vi "NM GlobalTest.vi"() -> ()   [LabVIEW 2010]
uses:
  C:/Program Files/National Instruments/LabVIEW 2010/vi.lib/ULx/ULx_LV.dll
  Program Files/National Instruments/LabVIEW 2010/vi.lib/ULx/ULx_LV.dll
  <vilib>/ULx/Create Channel.llb/ULx Create Channel (AI-Voltage-Basic).vi
  <vilib>/ULx/Create Channel.llb/ULx Create Channel (AI-Current-Basic).vi
  <vilib>/ULx/Create Channel.llb/ULx Create Channel (AI-Temperature).vi
  <vilib>/ULx/Create Channel.llb/ULx Create Channel (AO-Voltage-Basic).vi
  <vilib>/ULx/Create Channel.llb/ULx Create Channel (AO-Current-Basic).vi
  <vilib>/ULx/Create Channel.llb/ULx Create Channel (DI-Digital Input).vi
  <vilib>/ULx/Create Channel.llb/ULx Create Channel (DO-Digital Output).vi
  <vilib>/ULx/Create Channel.llb/ULx Create Channel (CI-Frequency).vi
  <vilib>/ULx/Create Channel.llb/ULx Create Channel (CI-Period).vi
  <vilib>/ULx/Create Channel.llb/ULx Create Channel (CI-Count Edges).vi
  <vilib>/ULx/Create Channel.llb/ULx Create Channel (CI-Position-Angular Encoder).vi
  <vilib>/ULx/Create Channel.llb/ULx Create Channel (CO-Pulse Generation-Frequency).vi
  <vilib>/ULx/Create Channel.llb/ULx Create Channel (CO-Pulse Generation-Time).vi
  <vilib>/ULx/Create Channel.llb/ULx Create Channel (CO-Pulse Generation-Ticks).vi
  <vilib>/ULx/Create Channel.llb/ULx Create Channel (CompI-Analog Input-Voltage).vi
  <vilib>/ULx/Create Channel.llb/ULx Create Channel (CompI-Analog Input-Temperature).vi
  <vilib>/ULx/Create Channel.llb/ULx Create Channel (CompI-Digital Input).vi
  <vilib>/ULx/Create Channel.llb/ULx Create Channel (CompI-Counter Input-Count Edges).vi
  <vilib>/ULx/Create Channel.llb/ULx Create Channel (CompO-Analog Output-Voltage).vi
  <vilib>/ULx/Create Channel.llb/ULx Create Channel (CompO-Digital Output).vi
  <vilib>/ULx/Timing.llb/ULx Timing (Sample Clock).vi
  <vilib>/ULx/Timing.llb/ULx Timing (Use Waveform).vi
  <vilib>/ULx/Timing.llb/ULx Timing (Implicit).vi
  <vilib>/ULx/Trigger.llb/ULx Basic Trigger (None).vi
  <vilib>/ULx/Trigger.llb/ULx Basic Trigger (Digital Edge).vi
  <vilib>/ULx/Trigger.llb/ULx Basic Trigger (Digital Level).vi
  <vilib>/ULx/Trigger.llb/ULx Basic Trigger (Analog Edge).vi
  <vilib>/ULx/Trigger.llb/ULx Basic Trigger (Digital Pattern).vi
  <vilib>/ULx/Trigger.llb/ULx Gated Trigger (None).vi
  <vilib>/ULx/Trigger.llb/ULx Gated Trigger (Digital Level).vi
  <vilib>/ULx/Trigger.llb/ULx Gated Trigger (Analog Level).vi
  <vilib>/ULx/Trigger.llb/ULx Gated Trigger (Analog Window).vi
  <vilib>/ULx/Trigger.llb/ULx Gated Trigger (Analog Hysteresis).vi
  <vilib>/ULx/Trigger.llb/ULx Composite Trigger Start (None).vi
  <vilib>/ULx/Trigger.llb/ULx Composite Trigger Start (ExtTTL).vi
  <vilib>/ULx/Trigger.llb/ULx Composite Trigger Start (Analog HW).vi
  <vilib>/ULx/Trigger.llb/ULx Composite Trigger Start (Analog SW).vi
  <vilib>/ULx/Trigger.llb/ULx Composite Trigger Start (Digital Pattern).vi
  <vilib>/ULx/Trigger.llb/ULx Composite Trigger Start (Counter).vi
  <vilib>/ULx/Trigger.llb/ULx Composite Trigger Stop (None).vi
  <vilib>/ULx/Trigger.llb/ULx Composite Trigger Stop (Analog SW).vi
  <vilib>/ULx/Trigger.llb/ULx Composite Trigger Stop (Digital Pattern).vi
  <vilib>/ULx/Trigger.llb/ULx Composite Trigger Stop (Counter).vi
  <vilib>/ULx/Write.llb/ULx Write (Analog 1D DBL 1Chan 1Samp).vi
  <vilib>/ULx/Write.llb/ULx Write (Analog Wfm 1Chan 1Samp).vi
  <vilib>/ULx/Write.llb/ULx Write (Analog 1D DBL 1Chan NSamp).vi
  <vilib>/ULx/Write.llb/ULx Write (Analog Wfm 1Chan NSamp).vi
  <vilib>/ULx/Write.llb/ULx Write (Analog 1D DBL NChan 1Samp).vi
  <vilib>/ULx/Write.llb/ULx Write (Analog 1D Wfm NChan 1Samp).vi
  <vilib>/ULx/Write.llb/ULx Write (Analog 2D DBL NChan NSamp).vi
  <vilib>/ULx/Write.llb/ULx Write (Analog 1D Wfm NChan NSamp).vi
  <vilib>/ULx/Write.llb/ULx Write (Digital 1D Bool NChan 1Samp 1Line).vi
  <vilib>/ULx/Write.llb/ULx Write (Digital 2D Bool NChan 1Samp NLine).vi
  <vilib>/ULx/Write.llb/ULx Write (Digital 1D U8 NChan 1Samp).vi
  <vilib>/ULx/Write.llb/ULx Write (Digital 1D U16 NChan 1Samp).vi
  <vilib>/ULx/Write.llb/ULx Write (Digital 1D U32 NChan 1Samp).vi
  <vilib>/ULx/Write.llb/ULx Write (Digital 1D Wfm NChan 1Samp).vi
  <vilib>/ULx/Write.llb/ULx Write (Digital 2D U8 NChan NSamp).vi
  <vilib>/ULx/Write.llb/ULx Write (Digital 2D U16 NChan NSamp).vi
  <vilib>/ULx/Write.llb/ULx Write (Digital 2D U32 NChan NSamp).vi
  <vilib>/ULx/Write.llb/ULx Write (Digital 1D Wfm NChan NSamp).vi
  <vilib>/ULx/Write.llb/ULx Write (Digital Bool 1Line 1Point).vi
  <vilib>/ULx/Write.llb/ULx Write (Digital 1D Bool 1Chan 1Samp).vi
  <vilib>/ULx/Write.llb/ULx Write (Digital U8 1Chan 1Samp).vi
  <vilib>/ULx/Write.llb/ULx Write (Digital U16 1Chan 1Samp).vi
  <vilib>/ULx/Write.llb/ULx Write (Digital U32 1Chan 1Samp).vi
  <vilib>/ULx/Write.llb/ULx Write (Digital Wfm 1Chan 1Samp).vi
  <vilib>/ULx/Write.llb/ULx Write (Digital 1D U8 1Chan NSamp).vi
  <vilib>/ULx/Write.llb/ULx Write (Digital 1D U16 1Chan NSamp).vi
  <vilib>/ULx/Write.llb/ULx Write (Digital 1D U32 1Chan NSamp).vi
  <vilib>/ULx/Write.llb/ULx Write (Digital Wfm 1Chan NSamp).vi
  <vilib>/ULx/Write.llb/ULx Write (Counter 1D Frequency NChan 1Samp).vi
  <vilib>/ULx/Write.llb/ULx Write (Counter 1D Time NChan 1Samp).vi
  <vilib>/ULx/Write.llb/ULx Write (Counter 1D Ticks NChan 1Samp).vi
  <vilib>/ULx/Write.llb/ULx Write (Counter Frequency 1Chan 1Samp).vi
  <vilib>/ULx/Write.llb/ULx Write (Counter Time 1Chan 1Samp).vi
  <vilib>/ULx/Write.llb/ULx Write (Counter Ticks 1Chan 1Samp).vi
  <vilib>/ULx/Write.llb/ULx Write (Composite 2D  NChan NSamp).vi
  <vilib>/ULx/Write.llb/ULx Write (Composite 1D Wfm NChan NSamp).vi
  <vilib>/ULx/Read.llb/ULx Read (Analog DBL 1Chan 1Samp).vi
  <vilib>/ULx/Read.llb/ULx Read (Analog Wfm 1Chan 1Samp).vi
  <vilib>/ULx/Read.llb/ULx Read (Analog 1D DBL 1Chan NSamp).vi
  <vilib>/ULx/Read.llb/ULx Read (Analog Wfm 1Chan NSamp).vi
  <vilib>/ULx/Read.llb/ULx Read (Analog 1D DBL NChan 1Samp).vi
  <vilib>/ULx/Read.llb/ULx Read (Analog 1D Wfm NChan 1Samp).vi
  <vilib>/ULx/Read.llb/ULx Read (Analog 2D DBL NChan NSamp).vi
  <vilib>/ULx/Read.llb/ULx Read (Analog 1D Wfm NChan NSamp).vi
  <vilib>/ULx/Read.llb/ULx Read (Digital 1D Bool NChan 1Samp 1Line).vi
  <vilib>/ULx/Read.llb/ULx Read (Digital 2D Bool NChan 1Samp NLine).vi
  <vilib>/ULx/Read.llb/ULx Read (Digital 1D U8 NChan 1Samp).vi
  <vilib>/ULx/Read.llb/ULx Read (Digital 1D U16 NChan 1Samp).vi
  <vilib>/ULx/Read.llb/ULx Read (Digital 1D U32 NChan 1Samp).vi
  <vilib>/ULx/Read.llb/ULx Read (Digital 1D Wfm NChan 1Samp).vi
  <vilib>/ULx/Read.llb/ULx Read (Digital 2D U8 NChan NSamp).vi
  <vilib>/ULx/Read.llb/ULx Read (Digital 2D U16 NChan NSamp).vi
  <vilib>/ULx/Read.llb/ULx Read (Digital 2D U32 NChan NSamp).vi
  <vilib>/ULx/Read.llb/ULx Read (Digital 1D Wfm NChan NSamp).vi
  <vilib>/ULx/Read.llb/ULx Read (Digital Bool 1Line 1Point).vi
  <vilib>/ULx/Read.llb/ULx Read (Digital 1D Bool 1Chan 1Samp).vi
  <vilib>/ULx/Read.llb/ULx Read (Digital U8 1Chan 1Samp).vi
  <vilib>/ULx/Read.llb/ULx Read (Digital U16 1Chan 1Samp).vi
  <vilib>/ULx/Read.llb/ULx Read (Digital U32 1Chan 1Samp).vi
  <vilib>/ULx/Read.llb/ULx Read (Digital Wfm 1Chan 1Samp).vi
  <vilib>/ULx/Read.llb/ULx Read (Digital 1D U8 1Chan NSamp).vi
  <vilib>/ULx/Read.llb/ULx Read (Digital 1D U16 1Chan NSamp).vi
  <vilib>/ULx/Read.llb/ULx Read (Digital 1D U32 1Chan NSamp).vi
  <vilib>/ULx/Read.llb/ULx Read (Digital Wfm 1Chan NSamp).vi
  <vilib>/ULx/Read.llb/ULx Read (Counter DBL 1Chan 1Samp).vi
  <vilib>/ULx/Read.llb/ULx Read (Counter U32 1Chan 1Samp).vi
  <vilib>/ULx/Read.llb/ULx Read (Counter 1D DBL 1Chan NSamp).vi
  <vilib>/ULx/Read.llb/ULx Read (Counter 1D U32 1Chan NSamp).vi
  <vilib>/ULx/Read.llb/ULx Read (Counter 1D DBL NChan 1Samp).vi
  <vilib>/ULx/Read.llb/ULx Read (Counter 1D U32 NChan 1Samp).vi
  <vilib>/ULx/Read.llb/ULx Read (Counter 2D DBL NChan NSamp).vi
  <vilib>/ULx/Read.llb/ULx Read (Counter 2D U32 NChan NSamp).vi
  <vilib>/ULx/Read.llb/ULx Read (Composite 2D NChan NSamp).vi
  <vilib>/ULx/Read.llb/ULx Read (Composite 1DWfm NChan NSamp).vi
panel:
  in  "Plots and Errors":enum32{"Error", "Plots"}(tab)
  out "message 2":string
  out "Single Channel\n  1-D Array":dbl[](graph)
  out "Multi-channel\n  2-D Array":dbl[][](graph)
  out "Single Channel \n  Waveform":waveform(dbl)(graph)
  out "Multi-channel\n  Waveform":waveform(dbl)[](graph)
  out "Multi-channel\n  Unsigned 8-bit":u8[][](graph)
  out "Multi-channel\n  Unsigned 32-bit":u32[][](graph)
  out "Multi-channel\n  Unsigned 16-bit":u16[][](graph)
  out "Single Channel\n  Unsigned 8-bit":u8[](graph)
  out "Single Channel\n  Unsigned 16-bit":u16[](graph)
  out "Single Channel\n  Unsigned 32-bit":u32[](graph)
  out "Single\n  Channel\n  Waveform":digitalwaveform(graph)
  out "Multi-\n  channel\n  Waveform":digitalwaveform[](graph)
  in  "Once":bool
  out "Stop Time":u32
  in  "Once":bool=TRUE
  in  "Once":bool=TRUE
  in  "Once":bool=TRUE
  in  "Active Channels":string
  in  "Data":bool
  in  "Tab Control 2":enum32{"Page 2"}(tab)
  in  "freq":dbl=5.0 format="%.2f"
  in  "sig type":T1(ring)
  in  "ampl":dbl=4.0 format="%0.2p"
  in  "samps":dbl=1000.0 format="%#.4p"
  in  "Chans":u32=1
  in  "offset":dbl format="%0.2p"
  in  "Tab Control 3":enum32{"Page 2"}(tab)
  in  "index":i32
  in  "freq":dbl=5.0 format="%0.2p"
  in  "atude":dbl=4.0 format="%0.2p"
  in  "signal type":T1(ring)
  in  "samples":dbl=100.0 max=40000.0
  in  "Mod Array":bool
  in  "Change":bool
  out "TC":bool
  in  "NI\nTC":bool
  out "task \ndone?":bool
  in  "Once":bool=TRUE
  in  "Once":bool=TRUE
  in  "Once":bool=TRUE
  out "Props":bool
  in  "Props":bool
  in  "GetSet":enum32{"Get Properties", "Set Properties"}(tab)
  out "Done":bool
  out "ErrorCode":i32
  in  "GetLev":T2(tab)
  out "AutoStart":bool
  in  "Avail":bool=TRUE
  out "Available Samples":u32 format="%#.4p"
  in  "AutoS":bool=TRUE
  out "CurrReadPos":dbl format="%#_4p"
  in  "Position":bool=TRUE
  out "OverWrite (Obs)":bool=TRUE
  in  "OWrite":bool
  out "ReadAllAvailSamp":bool
  in  "ReadAll":bool=TRUE
  out "TotalPerAcquired":dbl format="%#_3p"
  in  "Total":bool=TRUE
  out "RawData":bool
  out "NumberOfBoolsPer":u32
  in  "Raw":bool=TRUE
  in  "Bools":bool=TRUE
  in  "Read when Available Samples is greater than this":u32=1000 format="%#.4p"
  in  "y 2":bool
  out "AutoStatus":bool
  out "String 2":string="> this."
  in  "Space 2":bool=TRUE
  in  "WrtPos":bool=TRUE
  out "CurrentWritePosition":u32 format="%#.3p"
  out "Regenerate":bool
  in  "Reg 2":bool=TRUE
  out "SpaceAvailable":u32 format="%#.4p"
  out "Generated":dbl format="%#_4p"
  in  "Space":bool=TRUE
  in  "Gen":bool=TRUE
  out "BooleansPer":u32
  in  "Bools 2":bool=TRUE
  in  "GetWProps":enum32{"ULx", "DAQmx"}(tab)
  in  "RelTo":bool=TRUE
  in  "Offset 2":bool=TRUE
  out "CWP - Generated":u32 format="%#.4p"
  in  "Start when \"SpaceAvailable\"":u32=700 format="%#.4p"
  in  "TrigLib":enum32{"ULx", "DAQmx"}(tab)
  in  "GtULxTrgP":enum32{"Basic", "Gated", "Start", "Stop"}(tab)
  in  "Edge":bool=TRUE
  out "Edge":i32
  in  "Type":bool=TRUE
  out "Type":i32
  in  "Other":bool=TRUE
  out "AnalogLevel":dbl
  out "DigitalLevel":i32
  out "PretriggerCount":i32
  out "Slope":i32
  out "AnalogLevel":dbl
  out "DigitalLevel":i32
  out "When":i32
  out "WindowBottom":dbl
  out "WindowTop":dbl
  out "HighThreshold":dbl
  out "LowThreshold":dbl
  out "Position":i32
  out "Type":i32
  out "Hysteresis":i32
  out "AnalogHWSense":i32
  out "AnalogSWSense":i32
  out "CounterChannelSense":i32
  out "DigitalPatternSense":i32
  out "ExtTTLSense":i32
  out "Level":dbl
  out "TriggerChannelStr":string
  out "PretriggerCount":i32
  out "Channel":i32
  out "Variance":dbl
  out "Type":i32
  out "AnalogSWSense":i32
  out "CounterChannelSense":i32
  out "DigitalPatternSense":i32
  out "Level":dbl
  out "Channel":i32
  out "TriggerChannelStr":string
  out "Type":i32
  out "Variance":dbl
  out "Mode":i32
  in  "GetmxTrgPrp":enum32{"Start", "Pause", "Reference"}(tab)
  in  "GetTmgPrp":enum32{"ULx", "DAQmx"}(tab)
  in  "Burst":bool=TRUE
  out "BurstIO":bool
  in  "SIO":bool=TRUE
  out "SingleIO":bool
  out "DI.Word Xfer":bool
  in  "DiWord":bool=TRUE
  out "DO.Word Xfer":bool
  in  "DoWord":bool=TRUE
  out "Timing.ActualRate":sgl format="%#.6p"
  in  "Actual Rate":bool=TRUE
  out "DI.DWord (obs)":bool
  out "DO.DWord (obs)":bool
  in  "UFlow":bool=TRUE
  out "Channel.AI.Temp.Units":i32
  in  "Units":bool=TRUE
  in  "GetCiPrp":enum32{"ULx", "DAQmx"}(tab)
  in  "CIType":T3(tab)
  out "MeasurementTime":dbl
  out "StartingEdge":i32
  out "Units":i32
  out "Units":i32
  out "StartingEdge":i32
  out "MeasurementTime":dbl
  out "MccDirection":i32
  out "Edge":i32
  out "InitialCount":u32
  out "Gate Function":i32
  out "Max":u64
  out "Range Limit":bool
  out "Min":u64
  out "Output":bool
  out "Val 0":u64
  out "Val 1":u64
  out "Recycle":bool
  out "InvertGate":bool
  out "ClearOnRead":bool
  out "InitialState":i32
  out "DecodingType":i32
  out "InitialAngle":dbl
  out "PulsesPerRev":i32
  out "Units":i32
  out "ZIndexMode":i32
  in  "GetmxCIPrp":T3(tab)
  in  "GetCOPrp":enum32{"ULx", "DAQmx"}(tab)
  out "Frequency":dbl
  out "DutyCycle":dbl
  out "HighTicks":u32
  out "LowTicks":u32
  out "HighTime":dbl
  out "LowTime":dbl
  in  "Chans":bool=TRUE
  in  "Done 2":bool=TRUE
  in  "Err":bool=TRUE
  in  "Restart\nWhen\nDone":bool
  out "IT Done":bool
  out "NumChans":u32
  out "DevName":string
  in  "SetLev":T2(tab)=enum."Write"
  in  "Read.AutoStart":bool
  in  "Auto":bool
  in  "OWrite":bool
  in  "Overwrite (Obs)":bool=TRUE
  in  "ReadAll 2":bool
  in  "ReadAllAvailSamp":bool
  in  "AutoStatus 2":bool=TRUE
  in  "CurrentWritePosition":u32
  in  "WrtPos":bool
  in  "Regenerate":bool
  in  "Reg":bool
  in  "SetWProps":enum32{"ULx", "DAQmx"}(tab)
  in  "Rel":bool
  in  "Offset 3":bool
  in  "BurstIO 3":bool
  in  "SingleIO 3":bool
  in  "DIWord":bool
  in  "DIWord":bool
  in  "DOWord 2":bool
  in  "DOWord":bool
  in  "DIDWord":bool
  in  "DODWord":bool
  in  "MinMax":bool
  in  "Set Dir":bool
  in  "Gate":bool
  in  "ClearOnRead 2":bool
  in  "ClearOnRead":bool
  in  "RangeLimit":bool
  in  "RangeLimOn":bool
  in  "MaxLimit":u64
  in  "MinLimit":u64
  in  "Output":bool
  in  "Out0":u64
  in  "Out1":u64
  in  "OutputOn":bool
  in  "Recycle":bool
  in  "NoRecycle":bool
  in  "Gate Function 2":i32(ring) items=["Disabled", "Gate Counter", "Trigger Counter", "Count Direction", "Clear Count"]
  in  "Invert Gate":bool
  in  "Invert Gate":bool
  in  "MccDirection":i32
  in  "Mcc Direction":bool
  in  "MccEdge":i32
  in  "Mcc Edge":bool
  in  "Initial State":i32
  in  "Init State":bool
  in  "DutyCycle":dbl=0.5
  in  "Frequency":dbl=1.0 format="%_3f"
  in  "Freq 3":bool
  in  "Duty":bool
  out "Wait":bool
  in  "timeout":dbl=10.0 format="%.1g"
  in  "Wait":bool
  in  "Loop":u32=10
  in  "Clear\nError":bool
  out "Start 2":bool
  in  "Start":bool
  in  "Start":bool
  in  "Clear":bool
  in  "Stop":bool
  out "Idle 3":bool
  in  "Idle 2":bool
  in  "timeout":dbl=10.0 format="%.1g"
  in  "ReadType":T4(tab)
  in  "ARead":T5(tab)=enum."sCnS1D"
  out "data 35":dbl format="%_8g"
  out "data 36":waveform(dbl)={"t0"=timestamp(3286981568.47913 s since 1904-01-01), "dt"=10.0, "Y"=[0.0], "attributes"=variant("NI_ChannelName"=variant(string ""))}
  out "data 37":dbl[](array[numeric])
  in  "samples per":i32=-1
  out "data 38":waveform(dbl)
  in  "samples per":i32=-1
  out "data 39":dbl[](array[numeric])
  out "data 40":waveform(dbl)[](array[waveform])
  out "data 41":dbl[][](array[numeric])
  in  "samples per":i32=-1
  out "data 42":waveform(dbl)[](array[waveform])
  in  "samples per":i32=-1
  in  "nCOrsCDin":enum32{"Multi-Channel", " Single Channel"}(tab)
  in  "nCDIn":T6(tab)
  out "data 47":bool[](array[boolean])
  out "data 48":bool[][](array[boolean])
  out "data 49":u8[](array[numeric]) format="%x"
  out "data 50":u16[](array[numeric]) format="%x"
  out "data 51":u32[](array[numeric]) format="%x"
  out "data 52":digitalwaveform[](array[waveform])
  out "data 53":u8[][](array[numeric]) format="%x"
  in  "samples per":i32=-1
  out "data 54":u16[][](array[numeric]) format="%x"
  in  "samples per":i32=-1
  out "data 55":u32[][](array[numeric]) format="%x"
  in  "samples per":i32=-1
  out "data 56":digitalwaveform[](array[waveform])
  in  "samples per":i32=-1
  in  "sCDin":T7(tab)
  out "data 57":bool
  out "data 58":bool[](array[boolean])
  out "data 59":u8 format="%x"
  out "data 60":u16 format="%x"
  out "data 43":u32 format="%08x"
  out "data 62":digitalwaveform(waveform)
  out "data 63":u8[](array[numeric]) format="%x"
  in  "samples per":i32=-1
  out "data 64":u16[](array[numeric]) format="%x"
  in  "samples per":i32=-1
  out "data 65":u32[](array[numeric]) format="%x"
  in  "samples per":i32=-1
  out "data 66":digitalwaveform(waveform)
  in  "samples per":i32=-1
  in  "CtrRead":T8(tab)
  out "data 67":dbl format="%#_10f"
  out "Gauge":dbl(knob) scale=0.0..360.0
  out "data 68":u32 format="%x"
  out "data 69":dbl[](array[numeric]) format="%_6g"
  in  "samples per":i32=-1
  out "data 70":u32[](array[numeric])
  in  "samples per":i32=-1
  out "data 71":dbl[](array[numeric])
  out "data 72":u32[](array[numeric])
  out "data 73":dbl[][](array[numeric])
  in  "samples per":i32=-1
  out "data 74":u32[][](array[numeric])
  in  "samples per":i32=-1
  in  "CompRd":enum32{"2D", "1D Waveform"}(tab)
  out "analog data 4":dbl[][](array[numeric])
  out "digital data 3":u32[][](array[numeric]) format="%#.0f"
  out "counter data":u32[][](array[numeric])
  in  "Dig/Ctr":bool
  out "analog data 3":waveform(dbl)[](array[waveform])
  out "digital data 4":digitalwaveform[](array[waveform])
  in  "samples":i32=-1
  out "Read":bool
  in  "Read":bool
  in  "Item":u32=10
  out "Clear":bool
  out "Stop":bool
  out "Status":bool
  out "Write":bool
  out "Start":bool
  out "Trigger":bool
  out "Timing":bool
  out "CreateChans":bool
  in  "Start":bool
  in  "Clear":bool
  in  "Stop":bool
  out "String":string
  in  "TO":dbl=10.0 format="%.1g"
  out "Written":u32 format="%#.6p"
  in  "AutoStart":bool
  in  "If Cleared":bool=TRUE
  in  "Once":bool=TRUE
  in  "CreateChans":bool=TRUE
  in  "TaskType 2":T4(tab)
  in  "AWrite":T9(tab)=enum."sCnS1D"
  in  "data 2":dbl(slide) min=-5.05 max=5.05 scale=-5.05..5.05
  in  "data":waveform(dbl)={"t0"=timestamp(0 s since 1904-01-01), "dt"=0.0, "Y"=[]}
  out "data 3":dbl[](array[numeric]) format="%0.2f"
  out "data 4":waveform(dbl)
  in  "data 5":dbl[](array[numeric]) format="%0.2f"
  in  "data 6":waveform(dbl)[](array[waveform])
  out "data 7":dbl[][](array[numeric])
  out "data 8":waveform(dbl)[](array[waveform])
  in  "nOrsDChan":enum32{"Multi-Channel", "Single Channel"}(tab)
  in  "nDWrite":T6(tab)
  in  "data 12":bool[](array[boolean])
  in  "data 13":bool[][](array[boolean])
  in  "data 14":u8[](array[numeric]) format="%x"
  in  "data 15":u16[](array[numeric]) format="%x"
  in  "data 16":u32[](array[numeric]) format="%x"
  in  "data 17":digitalwaveform[](array[waveform])
  in  "data 18":u8[][](array[numeric]) format="%x"
  in  "data 19":u16[][](array[numeric])
  in  "data 20":u32[][](array[numeric]) format="%x"
  in  "data 21":digitalwaveform[](array[waveform])
  in  "sDWrite":T7(tab)
  in  "data 22":bool
  in  "data 23":bool[](array[boolean])
  in  "data 24":u8 format="%x"
  in  "data 25":u16 format="%x"
  in  "data 26":u32 format="%x"
  in  "data 27":digitalwaveform(waveform)={"t0"=timestamp(0 s since 1904-01-01), "dt"=0.0, "Y"={"transitions"=[], "data"=[]}, "error"={"status"=FALSE, "code"=37421928, "source"=""}}
  out "data 28":u8[](array[numeric])
  out "data 29":u16[](array[numeric]) format="%x"
  out "data 30":u32[](array[numeric]) format="%x"
  in  "data 31":digitalwaveform(waveform)={"t0"=timestamp(0 s since 1904-01-01), "dt"=0.0, "Y"={"transitions"=[], "data"=[]}, "error"={"status"=FALSE, "code"=37421928, "source"=""}}
  in  "nOrsCChan":enum32{"Multi-Channel", "Single Channel"}(tab)=enum."Single Channel"
  in  "nCtrWrite":enum32{"Frequency", "Time", "Ticks"}(tab)
  in  "data 32":cluster{"duty cycle":dbl, "frequency":dbl}[](array[cluster])
  in  "data 34":cluster{"high time":dbl, "low time":dbl}[](array[cluster])
  in  "data 33":cluster{"high ticks":u32, "low ticks":u32}[](array[cluster])
  in  "sCtrWrite":enum32{"Frequency", "Time", "Ticks"}(tab)
  in  "frequency":dbl=1.0 format="%_6g"
  in  "duty cycle":dbl=0.5 format="%_6g"
  in  "high time":dbl=0.01 format="%_6g"
  in  "low time":dbl=0.01 format="%_6g"
  in  "high ticks":u32=100
  in  "low ticks":u32=100
  in  "CompWrite":enum32{"2D", "1D Waveform"}(tab)
  out "DblArray 2":dbl[][](array[numeric])
  out "u32Array":u32[][](array[numeric])
  out "u32Plot":u32[][](graph)
  in  "Plot":bool
  in  "digital data 2":digitalwaveform[](array[waveform])
  out "WfmArray":waveform(dbl)[](array[waveform])
  in  "Write":bool
  in  "SelLib":enum32{"ULx", "DAQMx"}(tab)
  out "NumberOfChannels":u32
  out "Task":i32 format="%x"
  out "ToString":string
  in  "TaskType":T10(tab)
  in  "AChan":enum32{"ULx", "DAQmx"}(tab)
  in  "AnalogType":T11(tab)
  in  "min 3":dbl=-5.0
  in  "max 3":dbl=5.0
  in  "min 2":dbl=-5.0
  in  "max 2":dbl=5.0
  in  "min":dbl=-5.0
  in  "max":dbl=5.0
  in  "physical channels 3":refnum<k21>
  in  "physical channels 2":refnum<k21>
  in  "ULx":refnum<k21>
  in  "min 5":dbl=-0.01 format="%_4f"
  in  "max 5":dbl=0.01 format="%_4g"
  in  "min 4":dbl=-0.01 format="%_4f"
  in  "max 4":dbl=0.01 format="%_4g"
  in  "min":dbl=-0.01 format="%_4f"
  in  "max":dbl=0.01 format="%_4g"
  in  "physical channels 6":refnum<k21>
  in  "physical channels 5":refnum<k21>
  in  "ULx":refnum<k21>
  in  "units 3":i32(ring) items=["degC", "degF", "kelvin", "raw"]
  in  "units 2":i32(ring) items=["degC", "degF", "kelvin", "raw"]
  in  "units":i32(ring) items=["degC", "degF", "kelvin", "raw"]
  in  "physical channels 9":refnum<k21>
  in  "physical channels 8":refnum<k21>
  in  "ULx":refnum<k21>
  in  "physical channels 12":refnum<k21>
  in  "min 7":dbl=-5.0
  in  "max 7":dbl=5.0
  in  "physical channels 11":refnum<k21>
  in  "min 8":dbl=-5.0
  in  "max 8":dbl=5.0
  in  "min":dbl=-5.0
  in  "max":dbl=5.0
  in  "ULx":refnum<k21>
  in  "min 10":dbl=-10.0
  in  "max 10":dbl=10.0
  in  "min 11":dbl=-10.0
  in  "max 11":dbl=10.0
  in  "min":dbl=-10.0
  in  "max":dbl=10.0
  in  "physical channels 15":refnum<k21>
  in  "physical channels 14":refnum<k21>
  in  "ULx":refnum<k21>
  in  "DChan":enum32{"ULx", "DAQmx"}(tab)
  in  "DigitalType":enum32{"Digital Input", "Digital Output"}(tab)
  in  "line grouping 3":i32(ring)=1 items=["OneChannelForEachLine", "OneChannelForAllLines"]
  in  "line grouping 2":i32(ring)=1 items=["OneChannelForEachLine", "OneChannelForAllLines"]
  in  "line grouping":i32(ring)=1 items=["OneChannelForEachLine", "OneChannelForAllLines"]
  in  "lines 3":refnum<k21>
  in  "lines 2":refnum<k21>
  in  "ULx":refnum<k21>
  in  "line grouping 6":i32(ring)=1 items=["OneChannelForEachLine", "OneChannelForAllLines"]
  in  "line grouping 5":i32(ring)=1 items=["OneChannelForEachLine", "OneChannelForAllLines"]
  in  "line grouping":i32(ring)=1 items=["OneChannelForEachLine", "OneChannelForAllLines"]
  in  "lines 6":refnum<k21>
  in  "lines 5":refnum<k21>
  in  "ULx":refnum<k21>
  in  "CtrChan":enum32{"ULx", "DAQmx"}(tab)
  in  "CounterType":T12(tab)
  in  "measure time 3":dbl=0.01 format="%.3f"
  in  "measure time 2":dbl=0.01 format="%.3f"
  in  "measure time":dbl=0.01 format="%.7f"
  in  "starting edge 3":i32(ring) items=["Rising", "Falling"]
  in  "starting edge 2":i32(ring) items=["Rising", "Falling"]
  in  "starting edge":i32(ring) items=["Rising", "Falling"]
  in  "units 6":i32(ring) items=["Hz", "Ticks"]
  in  "units 5":i32(ring) items=["Hz", "Ticks"]
  in  "units":i32(ring) items=["Hz", "Ticks"]
  in  "counters 3":refnum<k21>
  in  "counters 2":refnum<k21>
  in  "ULx":refnum<k21>
  in  "measure time 5":dbl=0.01 format="%.3f"
  in  "measure time 4":dbl=0.01 format="%.3f"
  in  "measure time":dbl=0.01 format="%.5f"
  in  "starting edge 6":i32(ring) items=["Rising", "Falling"]
  in  "starting edge 5":i32(ring) items=["Rising", "Falling"]
  in  "starting edge":i32(ring) items=["Rising", "Falling"]
  in  "units 9":i32(ring) items=["Seconds", "Ticks"]
  in  "units 8":i32(ring) items=["Seconds", "Ticks"]
  in  "units":i32(ring) items=["Seconds", "Ticks"]
  in  "counters 6":refnum<k21>
  in  "counters 5":refnum<k21>
  in  "ULx":refnum<k21>
  in  "edge 3":i32(ring) items=["Rising", "Falling"]
  in  "edge 2":i32(ring) items=["Rising", "Falling"]
  in  "edge":i32(ring) items=["Rising", "Falling"]
  in  "direction 3":i32(ring) items=["CountUp", "CountDown"]
  in  "direction 2":i32(ring) items=["CountUp", "CountDown"]
  in  "initial count 3":u32
  in  "direction":i32(ring) items=["CountUp", "CountDown"]
  in  "initial count 2":u32
  in  "initial count":u32
  in  "counters 9":refnum<k21>
  in  "counters 8":refnum<k21>
  in  "ULx":refnum<k21>
  in  "pulses per 2":u32=360
  in  "initial angle\npulses per":dbl
  in  "type 2":i32(ring) items=["X1", "X2", "X4"]
  in  "index mode 2":i32(ring) items=["Disabled"=0, "LatchCounter"=8, "ResetCounter"=32]
  in  "units 11":i32(ring) items=["Degrees", "Radians", "Ticks"]
  in  "counters 11":refnum<k21>
  in  "initial angle\npulses per":dbl
  in  "pulses per":u32=360
  in  "type":i32(ring) items=["X1", "X2", "X4"]
  in  "index mode":i32(ring) items=["Disabled"=0, "LatchCounter"=8, "ResetCounter"=32]
  in  "units 10":i32(ring) items=["Degrees", "Radians", "Ticks"]
  in  "ULx":refnum<k21>
  in  "duty cycle 3":dbl=0.5 format="%.6f"
  in  "duty cycle 2":dbl=0.5 format="%.6f"
  in  "frequency 3":dbl=1.0 format="%.6f"
  in  "frequency 2":dbl=1.0 format="%.6f"
  in  "duty cycle":dbl=0.5 format="%.6f"
  in  "frequency":dbl=1.0 format="%.6f"
  in  "counters 14":refnum<k21>
  in  "counters 13":refnum<k21>
  in  "ULx":refnum<k21>
  in  "low time 3":dbl=0.01 format="%.6f"
  in  "high time 3":dbl=0.01 format="%.6f"
  in  "low time 2":dbl=0.01 format="%.6f"
  in  "high time 2":dbl=0.01 format="%.6f"
  in  "low time":dbl=0.01 format="%.8f"
  in  "high time":dbl=0.01 format="%.8f"
  in  "counters 19":refnum<k21>
  in  "counters 18":refnum<k21>
  in  "ULx":refnum<k21>
  in  "low ticks 3":u32=100
  in  "high ticks 3":u32=100
  in  "low ticks 2":u32=100
  in  "high ticks 2":u32=100
  in  "low ticks":u32=100
  in  "high ticks":u32=100
  in  "counters 20":refnum<k21>
  in  "counters 16":refnum<k21>
  in  "ULx":refnum<k21>
  in  "CompIn":enum32{"ULx", "DAQmx"}(tab)
  in  "CompType":T13(tab)
  in  "min 12":dbl=-5.0
  in  "max 12":dbl=5.0
  in  "min 9":dbl=-5.0
  in  "max 9":dbl=5.0
  in  "min":dbl=-5.0
  in  "max":dbl=5.0
  in  "physical channels 18":refnum<k21>
  in  "physical channels 17":refnum<k21>
  in  "ULx":refnum<k21>
  in  "units 12":i32(ring) items=["degC", "degF", "kelvin", "raw"]
  in  "units 7":i32(ring) items=["degC", "degF", "kelvin", "raw"]
  in  "units":i32(ring) items=["degC", "degF", "kelvin", "raw"]
  in  "physical channels 21":refnum<k21>
  in  "physical channels 20":refnum<k21>
  in  "ULx":refnum<k21>
  in  "ports 3":refnum<k21>
  in  "ports 2":refnum<k21>
  in  "ULx":refnum<k21>
  in  "edge 6":i32(ring) items=["Rising", "Falling"]
  in  "direction 6":i32(ring) items=["CountUp", "CountDown"]
  in  "initial count 6":u32
  in  "edge 5":i32(ring) items=["Rising", "Falling"]
  in  "direction 5":i32(ring) items=["CountUp", "CountDown"]
  in  "initial count 5":u32
  in  "edge":i32(ring) items=["Rising", "Falling"]
  in  "direction":i32(ring) items=["CountUp", "CountDown"]
  in  "initial count":u32
  in  "counters 23":refnum<k21>
  in  "counters 22":refnum<k21>
  in  "ULx":refnum<k21>
  in  "initial angle\npulses per":dbl
  in  "pulses per 4":dbl=24.0
  in  "type 4":dbl(ring)=2.0 items=["X1", "X2", "X4"]
  in  "z index mode 2":i32(ring) items=["Disabled"=0, "LatchCounter"=8, "ResetCounter"=32]
  in  "units 14":i32(ring) items=["Degrees", "Radians", "Ticks"]
  in  "initial angle\npulses per":dbl
  in  "pulses per 3":dbl=24.0
  in  "type":dbl(ring)=2.0 items=["X1", "X2", "X4"]
  in  "z index mode":i32(ring) items=["Disabled"=0, "LatchCounter"=8, "ResetCounter"=32]
  in  "units":i32(ring) items=["Degrees", "Radians", "Ticks"]
  in  "counters 25":refnum<k21>
  in  "ULx":refnum<k21>
  in  "ULx":refnum<k21>
  in  "physical channels 29":refnum<k21>
  in  "physical channels 30":refnum<k21>
  in  "max":dbl=5.0
  in  "min":dbl=-5.0
  in  "max 15":dbl=5.0
  in  "min 15":dbl=-5.0
  in  "max 18":dbl=5.0
  in  "min 18":dbl=-5.0
  in  "CompOut":enum32{"ULx", "DAQmx"}(tab)
  in  "CompOType":enum32{"AO Volts", "Digital Out", "AO Volts 2"}(tab)
  in  "min 14":dbl=-5.0
  in  "max 14":dbl=5.0
  in  "min 13":dbl=-5.0
  in  "max 13":dbl=5.0
  in  "min":dbl=-5.0
  in  "max":dbl=5.0
  in  "physical channels 24":refnum<k21>
  in  "physical channels 23":refnum<k21>
  in  "ULx":refnum<k21>
  in  "ports 6":refnum<k21>
  in  "ports 5":refnum<k21>
  in  "ULx":refnum<k21>
  in  "min 17":dbl=-5.0
  in  "max 17":dbl=5.0
  in  "min 16":dbl=-5.0
  in  "max 16":dbl=5.0
  in  "min":dbl=-5.0
  in  "max":dbl=5.0
  in  "physical channels 27":refnum<k21>
  in  "physical channels 26":refnum<k21>
  in  "ULx":refnum<k21>
  out "# of Loops":i32
  in  "Status\nLoop":bool
  out "Task Cleared":bool
  out "Task Stopped":bool
  in  "TrigType":enum32{"Basic", "Gated", "Start", "Stop"}(tab)
  in  "BasicType":T14(tab)
  in  "TrgEdge":enum32{"ULx", "DAQmx"}(tab)
  in  "ULx edge":i32(ring) items=["Rising", "Falling"]
  in  "pretrigger samples per channel":u32
  in  "pretrigger samples per channel":u32
  in  "level":i32(ring)=1 items=["Low", "High"]
  in  "chan":refnum<k21>
  in  "sensitivity":i32(ring) items=["AbovePattern", "BelowPattern", "EqualPattern", "NotEqualPattern"]
  in  "pattern":u64=32768 format="%04x"
  in  "mask":u64=65535 format="%04x"
  in  "pretrig samps":u32
  in  "pretrigger samples per channel":u32
  in  "level":dbl
  in  "slope":i32(ring) items=["Rising", "Falling"]
  in  "GatedType":T15(tab)
  in  "Level 3":i32(ring) items=["High", "Low"]
  in  "level":dbl
  in  "position":i32(ring) items=["Above", "Below"]
  in  "top":dbl=0.5
  in  "bottom":dbl
  in  "When":i32(ring) items=["InsideWindow", "OutsideWindow"]
  in  "hyst":i32(ring) items=["Negative", "Positive"]
  in  "low":dbl
  in  "high":dbl=0.5
  in  "StartType":T16(tab)
  in  "trigger sensitivity":i32(ring) items=["RisingEdge", "FallingEdge"]
  in  "variance":dbl
  in  "Level":dbl
  in  "sensitivity":i32(ring) items=["AboveLevel", "BelowLevel", "RisingEdge", "FallingEdge"]
  in  "trigger channel":refnum<k21>
  in  "pretrigger samples":u32
  in  "variance":dbl
  in  "Level":dbl
  in  "sensitivity":i32(ring) items=["AboveLevel", "BelowLevel", "RisingEdge", "FallingEdge"]
  in  "trigger channel":refnum<k21>
  in  "pretrigger samples":u32
  in  "variance":dbl
  in  "level":dbl
  in  "trigger sensitivity":i32(ring) items=["AboveLevel", "BelowLevel", "EqualLevel", "NotEqualLevel"]
  in  "trigger channel":refnum<k21>
  in  "pretrigger samples":u32
  in  "variance":dbl
  in  "level":dbl
  in  "trigger sensitivity":i32(ring) items=["AboveLevel", "BelowLevel", "EqualLevel", "NotEqualLevel"]
  in  "StopType":enum32{"None", "ASftwr", "DPtrn", "Ctr"}(tab)
  in  "trigger channel":refnum<k21>
  in  "variance":dbl
  in  "level":dbl
  in  "trigger sensitivity":i32(ring) items=["AboveLevel", "BelowLevel", "EqualLevel", "NotEqualLevel", "RisingEdge", "FallingEdge"]
  in  "trigger channel":refnum<k21>
  in  "level":dbl
  in  "variance":dbl
  in  "trigger sensitivity":i32(ring) items=["AboveLevel", "BelowLevel", "EqualLevel", "NotEqualLevel", "RisingEdge", "FallingEdge"]
  in  "trigger channel":refnum<k21>
  in  "trigger sensitivity":i32(ring) items=["AboveLevel", "BelowLevel", "EqualLevel", "NotEqualLevel", "RisingEdge", "FallingEdge"]
  in  "level":dbl
  in  "variance":dbl
  in  "Trig":bool caption="(F5)"
  in  "Start":bool
  in  "Timing":bool caption="(F4)"
  in  "Tab Control":enum32{"Clock", "Waveform", "Implicit"}(tab)
  in  "UDClock":enum32{"ULx", "DAQmx"}(tab)
  in  "samples per":i32=1000 format="%#.4p"
  in  "sample mode":i32(ring) items=["FiniteSamples", "ContinuousSamples"]
  in  "clock source":i32(ring) items=["OnboardClock", "ExternalClock", "NoClock"]
  in  "rate":dbl=1000.0 format="%#.4p"
  in  "TmgWfm":enum32{"ULx", "DAQmx"}(tab)
  in  "waveform":waveform(dbl)={"t0"=timestamp(0 s since 1904-01-01), "dt"=0.0, "Y"=[]}
  in  "sample mode 3":i32(ring) items=["FiniteSamples", "ContinuousSamples"]
  in  "TmgImp":enum32{"ULx", "DAQmx"}(tab)
  in  "samples per channel":i32=1000 format="%#.4p"
  in  "sample mode":i32(ring) items=["FiniteSamples", "ContinuousSamples"]
  out "Idle":bool
  in  "Idle":bool=TRUE
  in  "Submit":bool
  in  "stop":bool
  in  "Stop":bool
  in  "Clear":bool
  # "Current Task"
  # "Delays"
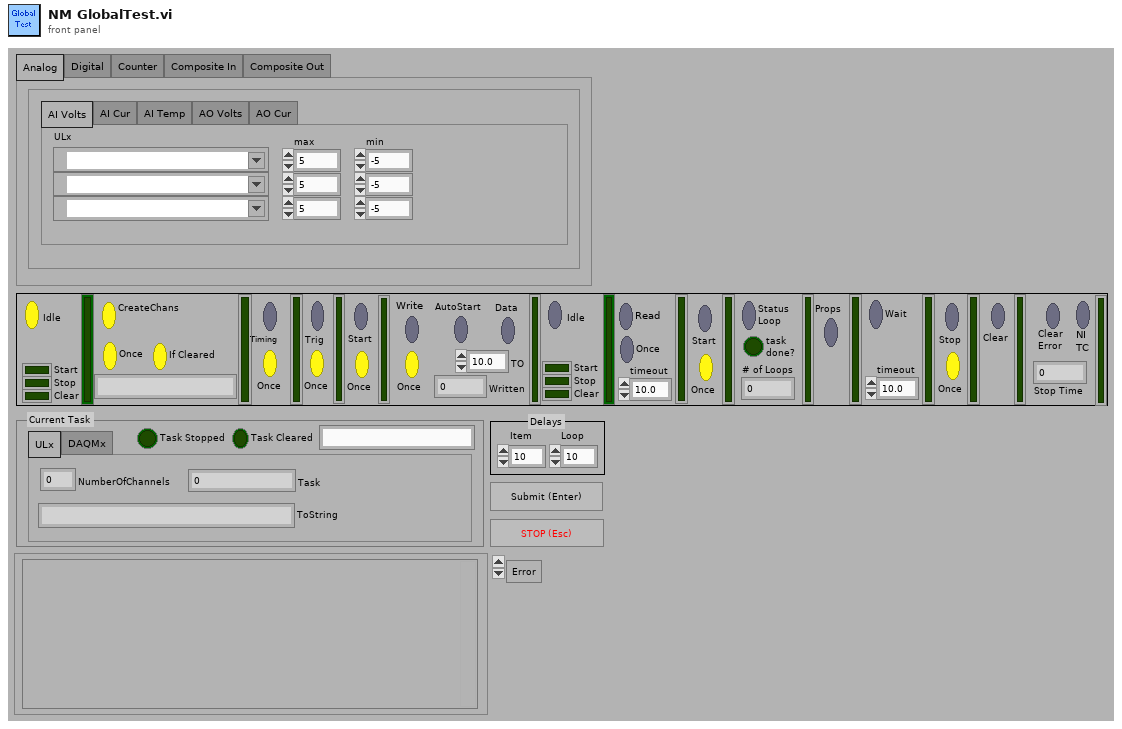
[diagram p1: front panel]
types:
  T1 = enum16{"Sine Wave", "Triangle Wave", "Square Wave", "Sawtooth Wave"}
  T2 = enum32{"Read", "Write", "Trigger", "Timing", "AI", "CI", "CO"}
  T3 = enum32{"Frequency", "Period", "Edges", "Encoder"}
  T4 = enum32{"Analog", "Digital", "Counter", "Composite"}
  T5 = enum32{"sCsSDbl", "sCsSWfm", "sCnS1D", "sCnSWfm", "nCsSDbl", "nCsSWfm", "nCnS2D", "nCnS1DWfm", "2DI16", "2DI32", "2DU16", "2DU32"}
  T6 = enum32{"nCsSBool", "nCsS2D", "nCsSU8", "nCsSU16", "nCsSU32", "nCsSWv", "nCnSU8", "nCnSU16", "nCnSU32", "nCnSWv"}
  T7 = enum32{"sCsSBool", "sCsS1D", "sCsSU8", "sCsSU16", "sCsSU32", "sCsSWv", "sCnSU8", "sCnSU16", "sCnSU32", "sCnSWv"}
  T8 = enum32{"sCsSDbl", "sCsSU32", "sCnSDbl", "sCnSU32", "nCsSDbl", "nCsSU32", "nCnSDbl", "nCnSU32"}
  T9 = enum32{"sCsSDbl", "sCsSWfm", "sCnS1D", "sCnSWfm", "nCsSDbl", "nCsSWfm", "nCnS2D", "nCnS1DWfm", "2DI16", "2DI32", "2DU16"}
  T10 = enum32{"Analog", "Digital", "Counter", "Composite In", "Composite Out"}
  T11 = enum32{"AI Volts", "AI Cur", "AI Temp", "AO Volts", "AO Cur"}
  T12 = enum32{"Freq In", "Period In", "Edge In", "Position In", "Freq Out", "Time Out", "Ticks Out"}
  T13 = enum32{"AI Volts", "AI Temp", "Digital In", "Counter In", "Encoder In", "AI Volts 2"}
  T14 = enum32{"None", "DEdge", "DLevel", "DPtrn", "AEdge"}
  T15 = enum32{"None", "DLevel", "ALevel", "AWindow", "AHyst"}
  T16 = enum32{"None", "ExtTTL", "AHdwr", "ASftwr", "DPtrn", "Ctr"}
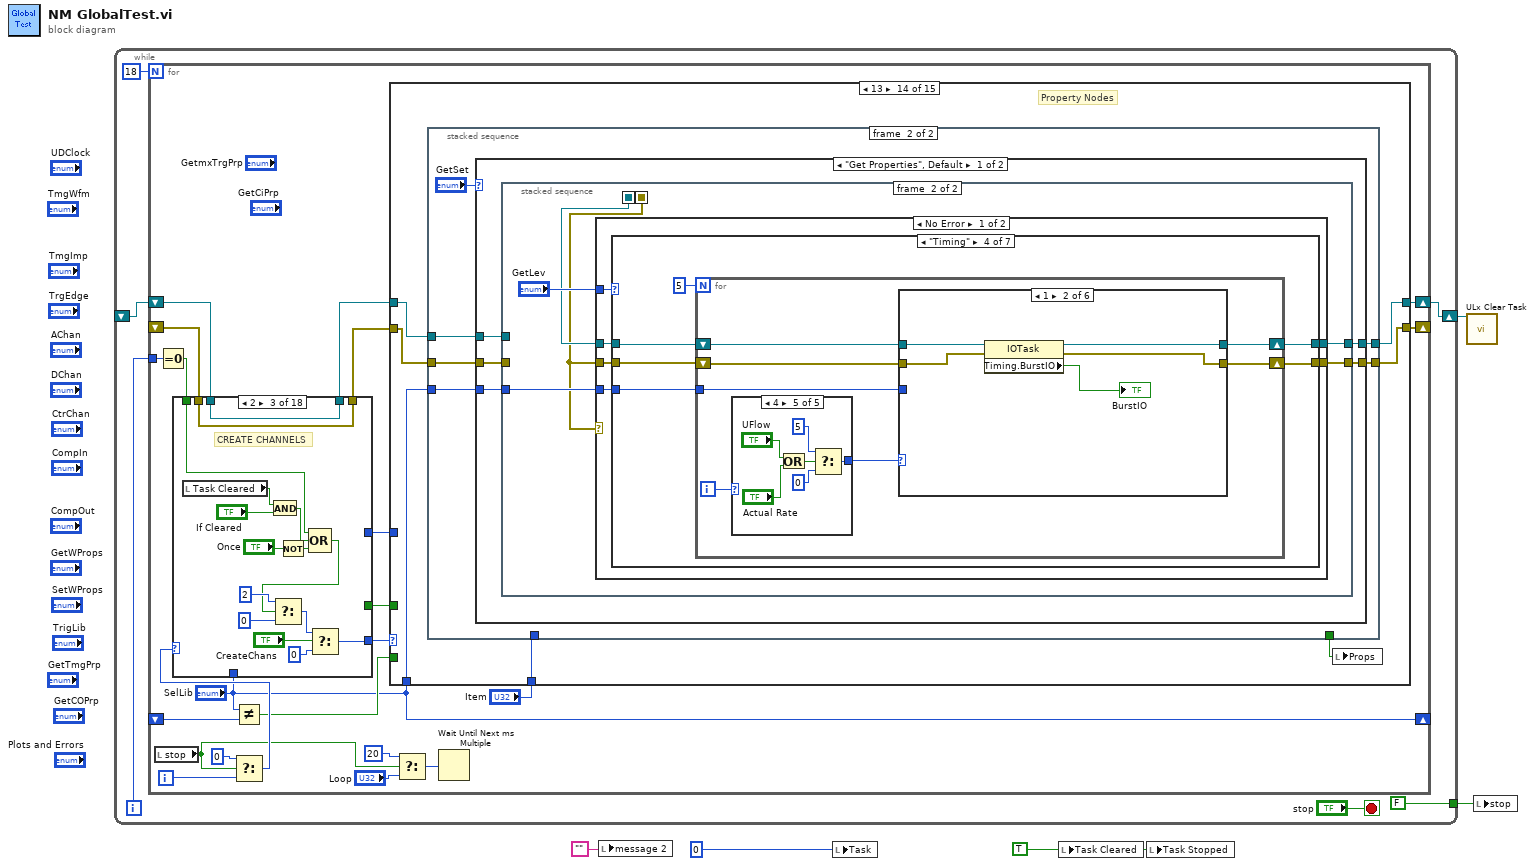
[diagram p0: block diagram]
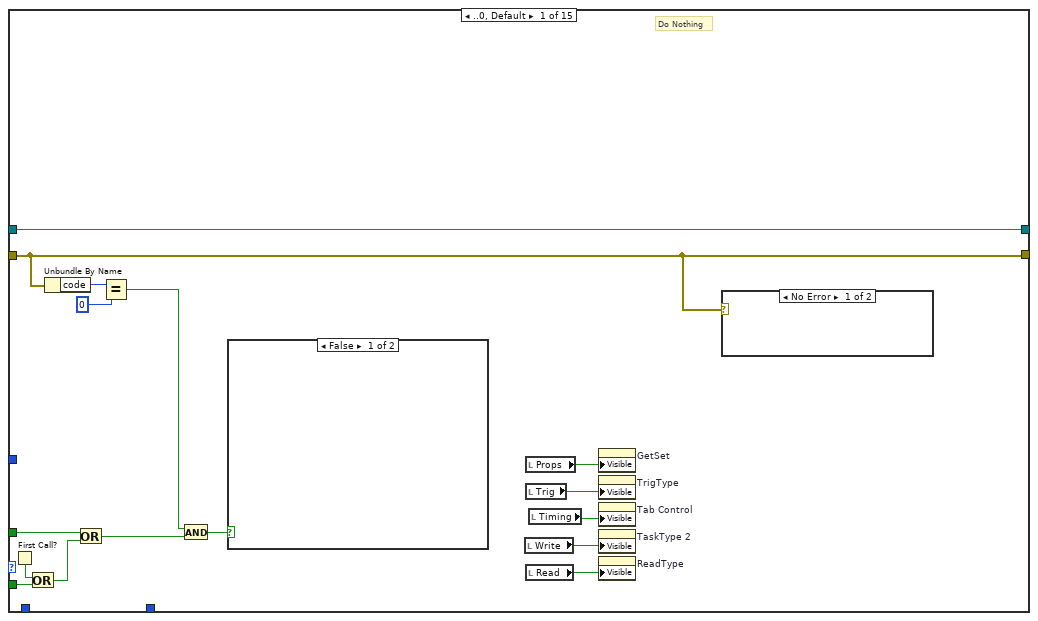
[diagram p2: hidden frame]
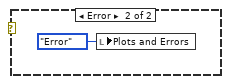
[diagram p3: hidden frame]
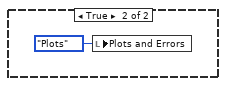
[diagram p4: hidden frame]
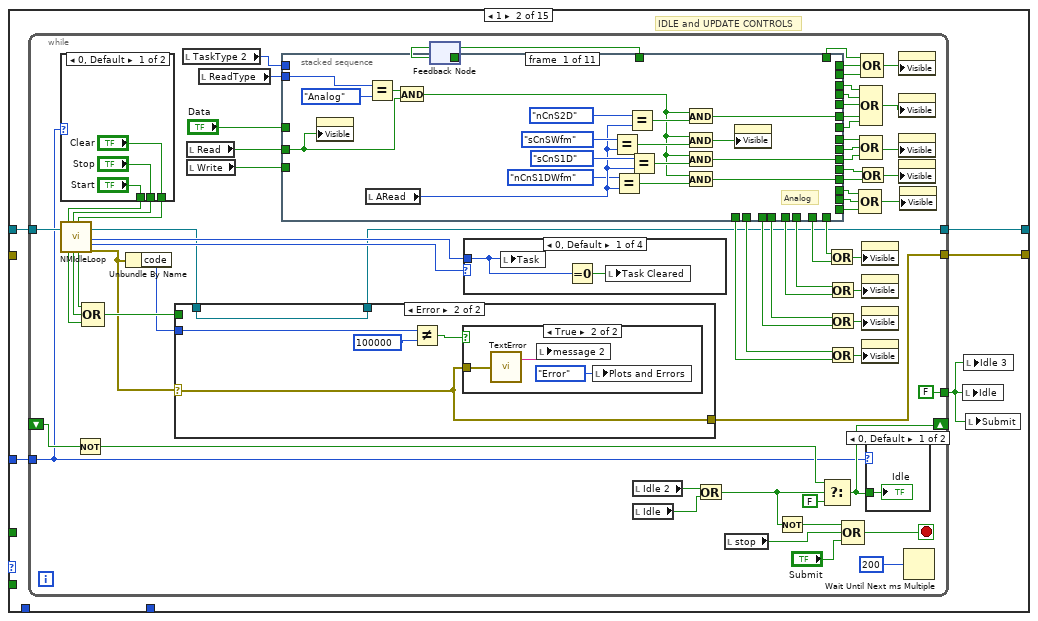
[diagram p5: hidden frame]
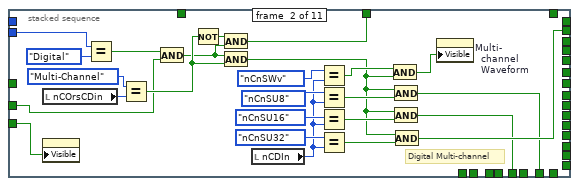
[diagram p6: hidden frame]
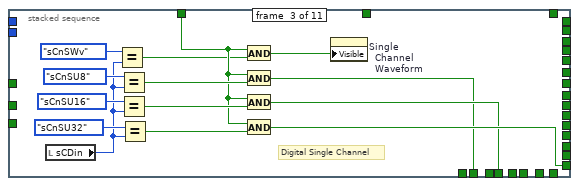
[diagram p7: hidden frame]
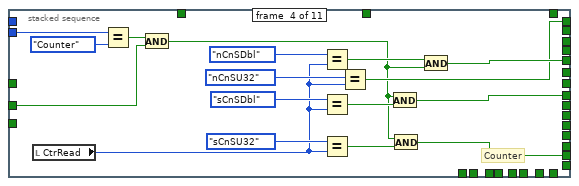
[diagram p8: hidden frame]
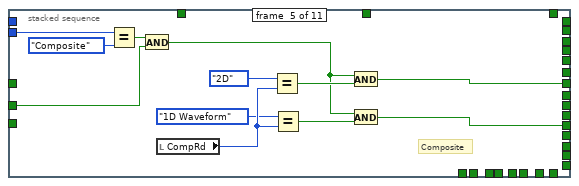
[diagram p9: hidden frame]
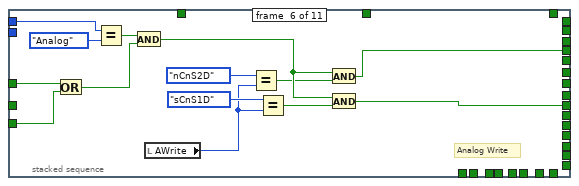
[diagram p10: hidden frame]
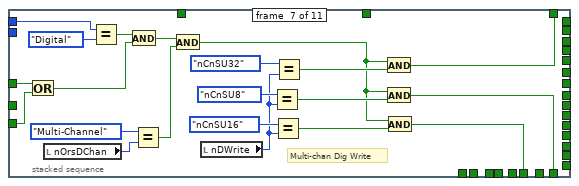
[diagram p11: hidden frame]
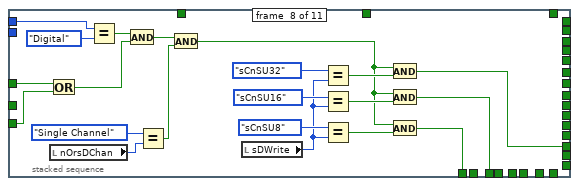
[diagram p12: hidden frame]
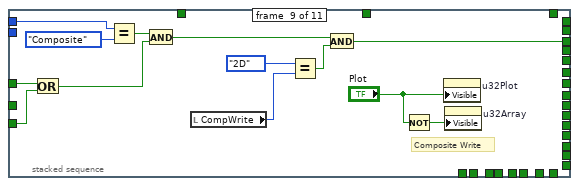
[diagram p13: hidden frame]
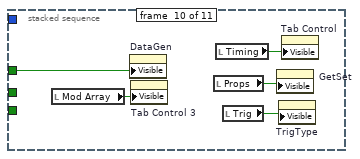
[diagram p14: hidden frame]
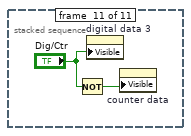
[diagram p15: hidden frame]
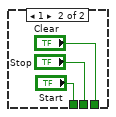
[diagram p16: hidden frame]
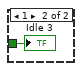
[diagram p17: hidden frame]
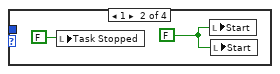
[diagram p18: hidden frame]
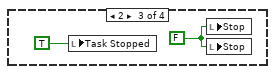
[diagram p19: hidden frame]
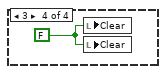
[diagram p20: hidden frame]
diagram:
  w4 = TRUE ("Task Cleared")
  n1 = while {
    tunnel: [FALSE ("stop")] -> w5
    shift-right: [w8] -> w2
    shift-left: _ -> [w6]
    i -> [w9]
    stop <- "stop" stop-if-true
    n2 = for {
      N: 18 -> [_]
      tunnel: w9 -> [w33]
      shift-right: [w30] -> _
      shift-left: _ -> [w20]
      shift-right: [w32] -> w8
      shift-left: w6 -> [w21]
      shift-right: ["SelLib"] -> _
      shift-left: _ -> [w17]
      i -> [w28]
      n3 = local read "stop"() -> (w23:bool)
      n4 = Equal To 0?(x=w33) -> (x = 0?=w22:bool)
      n5 = Not Equal?(x="SelLib", y=w17) -> (x != y?=w16:bool)
      n6 = Select(t=0, s=w23, f=w28) -> (s? t:f=w27:i32)
      n7 = case shown="2" w27 {
        tunnel: [0 ("f") w2825 w2841 3 ("f") w2849 w2855 w2861 w2867 w2873 w2879 w2886 w2893 w2898 w2904 w2911 w2921 w2925 0 ("f")] -> w31
        tunnel: w22 -> [_ _ w2834 _ _ _ _ _ _ _ _ _ _ _ _ _ _ _]
        tunnel: w21 -> [w2818 w2821 w2828 w2843 w2846 w2852 w2858 w2864 w2870 w2877 w2883 w2890 w2896 w2902 w2908 w2919 w2924 w2930]
        tunnel: "SelLib" -> [_ _ _ _ _ _ _ _ _ _ _ _ _ _ _ _ _ _]
        tunnel: w20 -> [w2813 w2822 w2829 w2845 w2847 w2853 w2859 w2865 w2871 w2878 w2884 w2891 w2897 w2903 w2909 w2916 w2929 w2932]
        tunnel: [_ 0 ("f") _ _ _ _ _ _ 1 ("f") _ 1 ("f") _ _ _ _ _ _ _] -> w18
        tunnel: [w2815 w2822 w2829 w2845 w2847 w2853 w2859 w2865 w2871 w2878 w2884 w2891 w2897 w2903 w2909 w2915 w2929 w2931] -> w15
        tunnel: [w2816 _ _ _ _ _ _ _ _ _ _ _ _ _ _ _ _ _] -> w13
        tunnel: [w2814 w2821 w2828 w2843 w2846 w2852 w2858 w2864 w2870 w2877 w2883 w2890 w2896 w2902 w2908 w2914 w2924 w2930] -> w12
        frame 0, Default {
          # "Do Nothing"
          n8 = case shown="Error" w2813 {
            frame No Error {
            }
            frame Error {
              n9 = local write "Idle"(TRUE ("Idle")) -> ()
            }
          }
          n10 = call "ULxTaskInfo.vi"("task in"=w2818, "error in (no error)"=w2813) -> ("task in 2"=w2814:refnum<k24>, "Task"=w2817:i32, "error out"=w2815:errorcluster)  [unwired: 2 out]
          n11 = Equal To 0?(x=w2817) -> (x = 0?=w2816:bool)
          n12 = local write "Task Cleared"(w2816) -> ()
        }
        frame 1 {
          # "IDLE and UPDATE CONTROLS"
          n13 = Select(t=1, s="Idle", f=0) -> (s? t:f=w2825:i32)
        }
        frame 2 {
          # "CREATE CHANNELS"
          n14 = local read "Task Cleared"() -> (w2839:bool)
          n15 = And(x=w2839, y="If Cleared") -> (x .and. y?=w2835:bool)
          n16 = Not(x="Once") -> (.not. x?=w2836:bool)
          n17 = Compound Arithmetic op=OR(w2834, w2835, w2836) -> (w2831:bool)
          n18 = Select(t=2, s=w2831, f=0) -> (s? t:f=w2830:i32)
          n19 = Select(t=w2830, s="CreateChans", f=0) -> (s? t:f=w2841:i32)
        }
        frame 3 {
          # "Channel Info"
        }
        frame 4 {
          # "TIMING"
          n20 = Select(t=4, s="Timing", f=0) -> (s? t:f=w2849:i32)
        }
        frame 5 {
          # "TRIGGERING"
          n21 = Select(t=5, s="Trig", f=0) -> (s? t:f=w2855:i32)
        }
        frame 6 {
          # "START"
          n22 = Select(t=6, s="Start", f=0) -> (s? t:f=w2861:i32)
        }
        frame 7 {
          # "WRITE"
          n23 = Select(t=7, s="Write", f=0) -> (s? t:f=w2867:i32)
        }
        frame 8 {
          # "IDLE and UPDATE CONTROLS"
          n24 = Select(t=1, s="Idle 2", f=0) -> (s? t:f=w2873:i32)
        }
        frame 9 {
          # "READ"
          n25 = Select(t=11, s="Read", f=0) -> (s? t:f=w2879:i32)
        }
        frame 10 {
          # "START"
          n26 = Select(t=6, s="Start", f=0) -> (s? t:f=w2886:i32)
        }
        frame 11 {
          # "STATUS"
          n27 = Select(t=8, s="Status\nLoop", f=0) -> (s? t:f=w2893:i32)
        }
        frame 12 {
          # "Property Nodes"
          n28 = Select(t=13, s="Props", f=0) -> (s? t:f=w2898:i32)
        }
        frame 13 {
          # "WAIT"
          n29 = Select(t=12, s="Wait", f=0) -> (s? t:f=w2904:i32)
        }
        frame 14 {
          # "STOP"
          n30 = Select(t=9, s="Stop", f=0) -> (s? t:f=w2911:i32)
        }
        frame 15 {
          # "CLEAR"
          n31 = call "TextError.vi"("error in"=w2916) -> ("message"=w2918:string)  [unwired: 1 in]
          n32 = local write "message 2"(w2918) -> ()
          n33 = call "ULxTaskInfo.vi"("task in"=w2919, "error in (no error)"=w2916) -> ("task in 2"=w2914:refnum<k24>, "Task"=w2917:i32, "error out"=w2915:errorcluster)  [unwired: 2 out]
          n34 = local write "Task"(w2917) -> ()
          n35 = Select(t=10, s="Clear", f=0) -> (s? t:f=w2921:i32)
        }
        frame 16 {
          # "Task Control"
          n36 = Select(t=14, s="NI\nTC", f=0) -> (s? t:f=w2925:i32)
        }
        frame 17 {
          n37 = case shown="True" "Clear\nError" {
            tunnel: w2932 -> [w2935 w2937]
            tunnel: [w2935 w2936] -> w2931
            frame False {
            }
            frame True {
              n38 = local write "Clear\nError"(FALSE) -> ()
              n39 = call <vilib>:"Clear Errors.vi"("error in (no error)"=w2937) -> ("error out"=w2936:errorcluster)  [unwired: 6 in]
            }
          }
        }
      }
      n40 = case shown="13" w31 {
        tunnel: "SelLib" -> [_ _ w342 w826 w855 w885 _ w1090 w1534 _ _ w1611 w1934 w1958 _]
        tunnel: w12 -> [w49 w56 w341 w829 w854 w887 w1062 w1089 w1538 w1573 w1602 w1613 w1937 w1956 w2809]
        tunnel: [w49 w55 w339 w818 w852 w894 w1054 w1087 w1536 w1570 _ w1610 w1936 w1954 w2809] -> w32
        tunnel: [w38 w52 w340 w817 w851 w893 w1053 w1086 w1535 w1566 w1599 w1609 w1935 w1955 w2804] -> w30
        tunnel: w15 -> [w38 _ w331 w828 w853 w886 w1061 w1088 w1537 w1569 w1601 w1612 w1938 w1957 w2804]
        tunnel: "Item" -> [_ _ w335 _ w849 w883 w1059 w1085 w1533 w1576 w1597 w1608 w1930 w1953 w2806]
        tunnel: w18 -> [_ w54 _ _ _ _ w1058 _ _ _ _ _ _ _ _]
        tunnel: w16 -> [w44 _ _ _ _ _ _ _ _ _ _ _ _ _ _]
        tunnel: w13 -> [w39 _ _ _ _ _ _ _ _ _ _ _ _ _ _]
        frame ..0, Default {
          # "Do Nothing"
          n41 = First Call?() -> (First Call?: T/F=w43:bool)
          n42 = Or(x=w43, y=w44) -> (x .or. y?=w41:bool)
          n43 = Unbundle By Name(w38) -> ("code"=w37:i32)
          n44 = Or(x=w39, y=w41) -> (x .or. y?=w40:bool)
          n45 = Equal?(x=w37, y=0) -> (x = y?=w34:bool)
          n46 = And(x=w34, y=w40) -> (x .and. y?=w35:bool)
          n47 = case shown="False" w35 {
            frame False {
            }
            frame True {
              n48 = local write "Plots and Errors"(enum32{"Error", "Plots"}."Plots" ("Plots and Errors")) -> ()
            }
          }
          n49 = local read "Write"() -> (w48:bool)
          n50 = local read "Props"() -> (w42:bool)
          n51 = local read "Trig"() -> (w46:bool)
          n52 = local read "Read"() -> (w45:bool)
          n53 = local read "Timing"() -> (w47:bool)
          n54 = property on="GetSet" class="TabCtl (strict)"("Visible"=w42) -> ()  [unwired: 2 in, 2 out]
          n55 = property on="TrigType" class="TabCtl (strict)"("Visible"=w46) -> ()  [unwired: 2 in, 2 out]
          n56 = property on="Tab Control" class="TabCtl (strict)"("Visible"=w47) -> ()  [unwired: 2 in, 2 out]
          n57 = property on="TaskType 2" class="TabCtl (strict)"("Visible"=w48) -> ()  [unwired: 2 in, 2 out]
          n58 = property on="ReadType" class="TabCtl (strict)"("Visible"=w45) -> ()  [unwired: 2 in, 2 out]
          n59 = case shown="No Error" w38 {
            frame No Error {
            }
            frame Error {
              n60 = local write "Plots and Errors"(enum32{"Error", "Plots"}."Error" ("Plots and Errors")) -> ()
            }
          }
        }
        frame 1 {
          # "IDLE and UPDATE CONTROLS"
          n61 = while {
            shift-right: [w109] -> _
            shift-left: _ -> [w122]
            tunnel: [FALSE ("f")] -> w53
            tunnel: w56 -> [w112]
            tunnel: [w57] -> w55
            tunnel: w54 -> [w105]
            tunnel: [w60] -> w52
            stop <- w124 stop-if-true
            n62 = case shown="0, Default" w105 {
              tunnel: ["Clear" "Clear"] -> w118
              tunnel: ["Stop" "Stop"] -> w117
              tunnel: ["Start" "Start"] -> w116
              frame 0, Default {
              }
              frame 1 {
              }
            }
            n63 = call "NMIdleLoop.vi"("ULx task in"=w112, "Start"=w116, "ExStop"=w117, "ExClear"=w118) -> ("Task Start"=w113:bool, "Task Stop"=w114:bool, "Task Clear"=w115:bool, "ULx task out"=w61:refnum<k24>, "Task"=w64:i32, "Function"=w110:i32, "error out"=w62:errorcluster)  [unwired: 9 in]
            n64 = Not(x=w122) -> (.not. x?=w121:bool)
            n65 = Compound Arithmetic op=OR(w115, w114, w113) -> (w111:bool)
            n66 = Unbundle By Name(w62) -> ("code"=w63:i32)
            n67 = case shown="Error" w62 {
              selector: w62 -> [w307 w324]
              tunnel: w111 -> [w309 _]
              tunnel: w63 -> [w308 w325]
              tunnel: w61 -> [w303 w323]
              tunnel: [w306 w324] -> w60
              tunnel: [w305 w323] -> w57
              frame No Error {
                n68 = Not A Number/Path/Refnum?(number/path/refnum=w303) -> (NaN/Path/Refnum?=w304:bool)
                n69 = case shown="False" w304 {
                  tunnel: w307 -> [w313 w315]
                  tunnel: w303 -> [w312 w316]
                  tunnel: [w311 w315] -> w306
                  tunnel: [w310 w316] -> w305
                  frame False {
                    n70 = call <vilib>:"ULx Is Task Done.vi"("task in"=w312, "error in"=w313) -> ("task out"=w310:refnum<k24>, "task done?"=w314:bool, "error out"=w311:errorcluster)  [unwired: 11 in]
                    n71 = local write "Task Stopped"(w314) -> ()
                  }
                  frame True {
                  }
                }
                n72 = case shown="True" w309 {
                  tunnel: w306 -> [_ w321]
                  tunnel: w308 -> [_ w318]
                  frame False {
                  }
                  frame True {
                    n73 = Not Equal?(x=w318, y=0) -> (x != y?=w317:bool)
                    n74 = call "TextError.vi"("error in"=w321) -> ("message"=w320:string)  [unwired: 1 in]
                    n75 = local write "message 2"(w320) -> ()
                    n76 = case shown="True" w317 {
                      frame False {
                      }
                      frame True {
                        n77 = local write "Plots and Errors"(enum32{"Error", "Plots"}."Error" ("Plots and Errors")) -> ()
                      }
                    }
                  }
                }
              }
              frame Error {
                n78 = Not Equal?(x=w325, y=100000) -> (x != y?=w326:bool)
                n79 = case shown="True" w326 {
                  tunnel: w324 -> [_ w330]
                  frame False {
                  }
                  frame True {
                    n80 = call "TextError.vi"("error in"=w330) -> ("message"=w329:string)  [unwired: 1 in]
                    n81 = local write "message 2"(w329) -> ()
                    n82 = local write "Plots and Errors"(enum32{"Error", "Plots"}."Error" ("Plots and Errors")) -> ()
                  }
                }
              }
            }
            n83 = local read "TaskType 2"() -> (w92:T4)
            n84 = local read "Read"() -> (w103:bool)
            n85 = local read "Write"() -> (w104:bool)
            n86 = local read "ReadType"() -> (w102:T4)
            n87 = feedback #1() -> (w100:bool)  [unwired: 1 in]
            n88 = stacked-sequence {
              tunnel: w104 -> [_ w155 _ _ _ w213 w227 w249 w269 _ _]
              tunnel: w103 -> [w126 w151 _ w184 w200 _ _ _ _ _ _]
              tunnel: w102 -> [w139 w167 _ w198 w210 _ _ _ _ _ _]
              tunnel: [_ w156 _ _ _ _ _ _ _ _ _] -> w101
              tunnel: w100 -> [_ _ w171 _ _ _ _ _ _ _ _]
              tunnel: [w131 _ _ _ _ _ _ _ _ _ _] -> w89
              tunnel: [_ _ _ w195 _ _ _ _ _ _ _] -> w91
              tunnel: [_ _ w176 _ _ _ _ _ _ _ _] -> w70
              tunnel: [_ _ _ w192 _ _ _ _ _ _ _] -> w69
              tunnel: [w130 _ _ _ _ _ _ _ _ _ _] -> w98
              tunnel: [_ _ _ w189 _ _ _ _ _ _ _] -> w97
              tunnel: [_ w152 _ _ _ _ _ _ _ _ _] -> w80
              tunnel: [_ _ _ w186 _ _ _ _ _ _ _] -> w79
              tunnel: [_ _ _ _ w206 _ _ _ _ _ _] -> w99
              tunnel: [w127 _ _ _ _ _ _ _ _ _ _] -> w94
              tunnel: [_ _ _ _ w202 _ _ _ _ _ _] -> w93
              tunnel: w92 -> [_ _ _ _ _ w224 w244 w264 w279 _ _]
              tunnel: [_ _ _ _ _ w220 _ _ _ _ _] -> w88
              tunnel: [_ _ _ _ _ w215 _ _ _ _ _] -> w87
              tunnel: [_ w150 _ _ _ _ _ _ _ _ _] -> w85
              tunnel: [_ w149 _ _ _ _ _ _ _ _ _] -> w83
              tunnel: [_ _ _ _ _ _ w237 _ _ _ _] -> w86
              tunnel: [_ _ _ _ _ _ w234 _ _ _ _] -> w81
              tunnel: [_ _ _ _ _ _ w229 _ _ _ _] -> w77
              tunnel: [_ _ w175 _ _ _ _ _ _ _ _] -> w75
              tunnel: [_ _ w174 _ _ _ _ _ _ _ _] -> w73
              tunnel: [_ _ _ _ _ _ _ w258 _ _ _] -> w72
              tunnel: [_ _ _ _ _ _ _ w255 _ _ _] -> w71
              tunnel: [_ _ _ _ _ _ _ w250 _ _ _] -> w67
              tunnel: [_ _ _ _ _ _ _ _ w273 _ _] -> w66
              tunnel: "Data" -> [_ _ _ _ _ w214 w228 w248 w270 w281 _]
              frame #0 {
                # "Analog"
                n89 = property on="ReadType" class="TabCtl (strict)"("Visible"=w126) -> ()  [unwired: 2 in, 2 out]
                n90 = local read "ARead"() -> (w129:T5)
                n91 = Equal?(x=w139, y=T4."Analog" ("ReadType")) -> (x = y?=w133:bool)
                n92 = And(x=w133, y=w126) -> (x .and. y?=w132:bool)
                n93 = Equal?(x=T5."sCnSWfm" ("ARead"), y=w129) -> (x = y?=w137:bool)
                n94 = Equal?(x=T5."nCnS1DWfm" ("ARead"), y=w129) -> (x = y?=w134:bool)
                n95 = Equal?(x=T5."nCnS2D" ("ARead"), y=w129) -> (x = y?=w138:bool)
                n96 = Equal?(x=T5."sCnS1D" ("ARead"), y=w129) -> (x = y?=w135:bool)
                n97 = And(x=w132, y=w138) -> (x .and. y?=w130:bool)
                n98 = And(x=w132, y=w137) -> (x .and. y?=w136:bool)
                n99 = And(x=w132, y=w135) -> (x .and. y?=w131:bool)
                n100 = And(x=w132, y=w134) -> (x .and. y?=w127:bool)
                n101 = property on="Single Channel \n  Waveform" class="WFGraph (strict)"("Visible"=w136) -> ()  [unwired: 2 in, 2 out]
              }
              frame #1 {
                # "Digital Multi-channel"
                n102 = local read "nCOrsCDin"() -> (w166:enum32{"Multi-Channel", " Single Channel"})
                n103 = property on="TaskType 2" class="TabCtl (strict)"("Visible"=w155) -> ()  [unwired: 2 in, 2 out]
                n104 = Equal?(x=w167, y=T4."Digital" ("ReadType")) -> (x = y?=w154:bool)
                n105 = Equal?(x=enum32{"Multi-Channel", " Single Channel"}."Multi-Channel" ("nCOrsCDin"), y=w166) -> (x = y?=w158:bool)
                n106 = And(x=w154, y=w151) -> (x .and. y?=w153:bool)
                n107 = Not(x=w158) -> (.not. x?=w157:bool)
                n108 = And(x=w157, y=w153) -> (x .and. y?=w156:bool)
                n109 = And(x=w153, y=w158) -> (x .and. y?=w145:bool)
                n110 = local read "nCDIn"() -> (w148:T6)
                n111 = Equal?(x=T6."nCnSWv" ("nCDIn"), y=w148) -> (x = y?=w146:bool)
                n112 = Equal?(x=T6."nCnSU8" ("nCDIn"), y=w148) -> (x = y?=w163:bool)
                n113 = Equal?(x=T6."nCnSU16" ("nCDIn"), y=w148) -> (x = y?=w159:bool)
                n114 = Equal?(x=T6."nCnSU32" ("nCDIn"), y=w148) -> (x = y?=w161:bool)
                n115 = And(x=w146, y=w145) -> (x .and. y?=w144:bool)
                n116 = And(x=w145, y=w163) -> (x .and. y?=w150:bool)
                n117 = And(x=w145, y=w159) -> (x .and. y?=w149:bool)
                n118 = And(x=w145, y=w161) -> (x .and. y?=w152:bool)
                n119 = property on="Multi-\n  channel\n  Waveform" class="DigitalGraph (strict)"("Visible"=w144) -> ()  [unwired: 2 in, 2 out]
              }
              frame #2 {
                # "Digital Single Channel"
                n120 = local read "sCDin"() -> (w173:T7)
                n121 = Equal?(x=T7."sCnSWv" ("sCDin"), y=w173) -> (x = y?=w170:bool)
                n122 = Equal?(x=T7."sCnSU8" ("sCDin"), y=w173) -> (x = y?=w181:bool)
                n123 = Equal?(x=T7."sCnSU16" ("sCDin"), y=w173) -> (x = y?=w179:bool)
                n124 = Equal?(x=T7."sCnSU32" ("sCDin"), y=w173) -> (x = y?=w177:bool)
                n125 = And(x=w171, y=w170) -> (x .and. y?=w169:bool)
                n126 = And(x=w171, y=w181) -> (x .and. y?=w174:bool)
                n127 = And(x=w171, y=w179) -> (x .and. y?=w175:bool)
                n128 = And(x=w171, y=w177) -> (x .and. y?=w176:bool)
                n129 = property on="Single\n  Channel\n  Waveform" class="DigitalGraph (strict)"("Visible"=w169) -> ()  [unwired: 2 in, 2 out]
              }
              frame #3 {
                # "Counter"
                n130 = local read "CtrRead"() -> (w187:T8)
                n131 = Equal?(x=w198, y=T4."Counter" ("ReadType")) -> (x = y?=w185:bool)
                n132 = And(x=w185, y=w184) -> (x .and. y?=w183:bool)
                n133 = Equal?(x=T8."nCnSDbl" ("CtrRead"), y=w187) -> (x = y?=w190:bool)
                n134 = Equal?(x=T8."sCnSDbl" ("CtrRead"), y=w187) -> (x = y?=w196:bool)
                n135 = Equal?(x=T8."sCnSU32" ("CtrRead"), y=w187) -> (x = y?=w193:bool)
                n136 = Equal?(x=T8."nCnSU32" ("CtrRead"), y=w187) -> (x = y?=w186:bool)
                n137 = And(x=w183, y=w196) -> (x .and. y?=w195:bool)
                n138 = And(x=w183, y=w193) -> (x .and. y?=w192:bool)
                n139 = And(x=w190, y=w183) -> (x .and. y?=w189:bool)
              }
              frame #4 {
                # "Composite"
                n140 = Equal?(x=w210, y=T4."Composite" ("ReadType")) -> (x = y?=w209:bool)
                n141 = And(x=w209, y=w200) -> (x .and. y?=w201:bool)
                n142 = local read "CompRd"() -> (w205:enum32{"2D", "1D Waveform"})
                n143 = Equal?(x=enum32{"2D", "1D Waveform"}."2D" ("CompRd"), y=w205) -> (x = y?=w207:bool)
                n144 = Equal?(x=enum32{"2D", "1D Waveform"}."1D Waveform" ("CompRd"), y=w205) -> (x = y?=w203:bool)
                n145 = And(x=w201, y=w207) -> (x .and. y?=w206:bool)
                n146 = And(x=w201, y=w203) -> (x .and. y?=w202:bool)
              }
              frame #5 {
                # "Analog Write"
                n147 = Or(x=w214, y=w213) -> (x .or. y?=w212:bool)
                n148 = Equal?(x=w224, y=T4."Analog" ("TaskType 2")) -> (x = y?=w222:bool)
                n149 = And(x=w222, y=w212) -> (x .and. y?=w217:bool)
                n150 = local read "AWrite"() -> (w218:T9)
                n151 = Equal?(x=T9."nCnS2D" ("AWrite"), y=w218) -> (x = y?=w216:bool)
                n152 = Equal?(x=T9."sCnS1D" ("AWrite"), y=w218) -> (x = y?=w221:bool)
                n153 = And(x=w217, y=w216) -> (x .and. y?=w215:bool)
                n154 = And(x=w217, y=w221) -> (x .and. y?=w220:bool)
              }
              frame #6 {
                # "Multi-chan Dig Write"
                n155 = Or(x=w228, y=w227) -> (x .or. y?=w226:bool)
                n156 = local read "nOrsDChan"() -> (w242:enum32{"Multi-Channel", "Single Channel"})
                n157 = Equal?(x=w244, y=T4."Digital" ("TaskType 2")) -> (x = y?=w245:bool)
                n158 = And(x=w245, y=w226) -> (x .and. y?=w238:bool)
                n159 = Equal?(x=enum32{"Multi-Channel", "Single Channel"}."Multi-Channel" ("nOrsDChan"), y=w242) -> (x = y?=w239:bool)
                n160 = And(x=w238, y=w239) -> (x .and. y?=w230:bool)
                n161 = local read "nDWrite"() -> (w232:T6)
                n162 = Equal?(x=T6."nCnSU8" ("nDWrite"), y=w232) -> (x = y?=w240:bool)
                n163 = Equal?(x=T6."nCnSU16" ("nDWrite"), y=w232) -> (x = y?=w236:bool)
                n164 = Equal?(x=T6."nCnSU32" ("nDWrite"), y=w232) -> (x = y?=w231:bool)
                n165 = And(x=w230, y=w231) -> (x .and. y?=w229:bool)
                n166 = And(x=w230, y=w240) -> (x .and. y?=w237:bool)
                n167 = And(x=w230, y=w236) -> (x .and. y?=w234:bool)
              }
              frame #7 {
                n168 = Or(x=w248, y=w249) -> (x .or. y?=w247:bool)
                n169 = local read "nOrsDChan"() -> (w262:enum32{"Multi-Channel", "Single Channel"})
                n170 = Equal?(x=w264, y=T4."Digital" ("TaskType 2")) -> (x = y?=w266:bool)
                n171 = And(x=w266, y=w247) -> (x .and. y?=w265:bool)
                n172 = Equal?(x=enum32{"Multi-Channel", "Single Channel"}."Single Channel" ("nOrsDChan"), y=w262) -> (x = y?=w261:bool)
                n173 = And(x=w265, y=w261) -> (x .and. y?=w251:bool)
                n174 = local read "sDWrite"() -> (w252:T7)
                n175 = Equal?(x=T7."sCnSU32" ("sDWrite"), y=w252) -> (x = y?=w254:bool)
                n176 = Equal?(x=T7."sCnSU16" ("sDWrite"), y=w252) -> (x = y?=w257:bool)
                n177 = Equal?(x=T7."sCnSU8" ("sDWrite"), y=w252) -> (x = y?=w259:bool)
                n178 = And(x=w251, y=w254) -> (x .and. y?=w250:bool)
                n179 = And(x=w251, y=w257) -> (x .and. y?=w255:bool)
                n180 = And(x=w251, y=w259) -> (x .and. y?=w258:bool)
              }
              frame #8 {
                # "Composite Write"
                n181 = Or(x=w270, y=w269) -> (x .or. y?=w268:bool)
                n182 = Equal?(x=w279, y=T4."Composite" ("TaskType 2")) -> (x = y?=w278:bool)
                n183 = And(x=w278, y=w268) -> (x .and. y?=w274:bool)
                n184 = local read "CompWrite"() -> (w276:enum32{"2D", "1D Waveform"})
                n185 = Equal?(x=enum32{"2D", "1D Waveform"}."2D" ("CompWrite"), y=w276) -> (x = y?=w275:bool)
                n186 = And(x=w274, y=w275) -> (x .and. y?=w273:bool)
                n187 = Not(x="Plot") -> (.not. x?=w272:bool)
                n188 = property on="u32Plot" class="WFGraph (strict)"("Visible"="Plot") -> ()  [unwired: 2 in, 2 out]
                n189 = property on="u32Array" class="Arr (strict)"("Visible"=w272) -> ()  [unwired: 2 in, 2 out]
              }
              frame #9 {
                n190 = local read "Mod Array"() -> (w283:bool)
                n191 = property on="DataGen" class="TabCtl (strict)"("Visible"=w281) -> ()  [unwired: 2 in, 2 out]
                n192 = property on="Tab Control 3" class="TabCtl (strict)"("Visible"=w283) -> ()  [unwired: 2 in, 2 out]
                n193 = local read "Props"() -> (w284:bool)
                n194 = local read "Timing"() -> (w285:bool)
                n195 = local read "Trig"() -> (w282:bool)
                n196 = property on="GetSet" class="TabCtl (strict)"("Visible"=w284) -> ()  [unwired: 2 in, 2 out]
                n197 = property on="TrigType" class="TabCtl (strict)"("Visible"=w282) -> ()  [unwired: 2 in, 2 out]
                n198 = property on="Tab Control" class="TabCtl (strict)"("Visible"=w285) -> ()  [unwired: 2 in, 2 out]
              }
              frame #10 {
                n199 = Not(x="Dig/Ctr") -> (.not. x?=w286:bool)
                n200 = property on="digital data 3" class="Arr (strict)"("Visible"="Dig/Ctr") -> ()  [unwired: 2 in, 2 out]
                n201 = property on="counter data" class="Arr (strict)"("Visible"=w286) -> ()  [unwired: 2 in, 2 out]
              }
            }
            n202 = feedback-in #1(w101) -> ()
            n203 = case shown="0, Default" w110 {
              tunnel: w64 -> [w296 _ _ _]
              frame 0, Default {
                n204 = local write "Task"(w296) -> ()
                n205 = Equal To 0?(x=w296) -> (x = 0?=w297:bool)
                n206 = local write "Task Cleared"(w297) -> ()
              }
              frame 1 {
                w299 = FALSE ("Start 2")
                n207 = local write "Task Stopped"(FALSE ("Task Stopped")) -> ()
                n208 = local write "Start"(w299) -> ()
                n209 = local write "Start"(w299) -> ()
              }
              frame 2 {
                w301 = FALSE ("Stop")
                n210 = local write "Task Stopped"(TRUE ("Task Stopped")) -> ()
                n211 = local write "Stop"(w301) -> ()
                n212 = local write "Stop"(w301) -> ()
              }
              frame 3 {
                w302 = FALSE ("Clear")
                n213 = local write "Clear"(w302) -> ()
                n214 = local write "Clear"(w302) -> ()
              }
            }
            n215 = local read "Idle 2"() -> (w106:bool)
            n216 = local read "Idle"() -> (w108:bool)
            n217 = Or(x=w106, y=w108) -> (x .or. y?=w107:bool)
            n218 = local read "stop"() -> (w59:bool)
            n219 = Not(x=w107) -> (.not. x?=w58:bool)
            n220 = Select(t=w121, s=w107, f=FALSE) -> (s? t:f=w109:bool)
            n221 = Or(x=w86, y=w85) -> (x .or. y?=w84:bool)
            n222 = Or(x=w81, y=w83) -> (x .or. y?=w82:bool)
            n223 = Or(x=w75, y=w71) -> (x .or. y?=w76:bool)
            n224 = Or(x=w73, y=w72) -> (x .or. y?=w74:bool)
            n225 = Compound Arithmetic op=OR(w58, w59, "Submit") -> (w124:bool)
            n226 = Or(x=w93, y=w94) -> (x .or. y?=w95:bool)
            n227 = Compound Arithmetic op=OR(w67, w69, w70) -> (w68:bool)
            n228 = Compound Arithmetic op=OR(w66, w87, w97, w98, w99) -> (w96:bool)
            n229 = Compound Arithmetic op=OR(w91, w88, w89) -> (w90:bool)
            n230 = Compound Arithmetic op=OR(w77, w79, w80) -> (w78:bool)
            n231 = property on="Multi-channel\n  Unsigned 8-bit" class="WFGraph (strict)"("Visible"=w84) -> ()  [unwired: 2 in, 2 out]
            n232 = property on="Multi-channel\n  Unsigned 16-bit" class="WFGraph (strict)"("Visible"=w82) -> ()  [unwired: 2 in, 2 out]
            n233 = property on="Single Channel\n  Unsigned 16-bit" class="WFGraph (strict)"("Visible"=w76) -> ()  [unwired: 2 in, 2 out]
            n234 = property on="Single Channel\n  Unsigned 8-bit" class="WFGraph (strict)"("Visible"=w74) -> ()  [unwired: 2 in, 2 out]
            n235 = case shown="0, Default" w105 {
              tunnel: w109 -> [w294 w295]
              frame 0, Default {
                "Idle" <- w294
              }
              frame 1 {
                "Idle 3" <- w295
              }
            }
            n236 = property on="Multi-channel\n  Unsigned 32-bit" class="WFGraph (strict)"("Visible"=w78) -> ()  [unwired: 2 in, 2 out]
            n237 = property on="Multi-channel\n  2-D Array" class="WFGraph (strict)"("Visible"=w96) -> ()  [unwired: 2 in, 2 out]
            n238 = property on="Single Channel\n  1-D Array" class="WFGraph (strict)"("Visible"=w90) -> ()  [unwired: 2 in, 2 out]
            n239 = property on="Multi-channel\n  Waveform" class="WFGraph (strict)"("Visible"=w95) -> ()  [unwired: 2 in, 2 out]
            n240 = property on="Single Channel\n  Unsigned 32-bit" class="WFGraph (strict)"("Visible"=w68) -> ()  [unwired: 2 in, 2 out]
            n241 = Wait Until Next ms Multiple(millisecond multiple=u32 200) -> ()  [unwired: 1 out]
          }
          n242 = local write "Idle"(w53) -> ()
          n243 = local write "Idle 3"(w53) -> ()
          n244 = local write "Submit"(w53) -> ()
        }
        frame 2 {
          # "CREATE CHANNELS"
          n245 = case shown="\"Counter\"" "TaskType" {
            tunnel: [w354 w457 w492 w638 w750] -> w339
            tunnel: [w353 w456 w494 w639 w752] -> w338
            tunnel: [w352 w455 w493 w640 w751] -> w337
            tunnel: w342 -> [_ _ _ _ _]
            tunnel: w341 -> [_ _ _ _ _]
            tunnel: [w351 w454 w491 w637 w749] -> w332
            tunnel: w331 -> [w343 _ _ _ _]
            frame "Analog", Default {
              n246 = case shown="\"AI Cur\"" "AnalogType" {
                tunnel: [w360 w387 w405 w424 w443] -> w352
                tunnel: [w359 w388 w406 w425 w444] -> w353
                tunnel: [w358 w394 w412 w431 w450] -> w354
                tunnel: ["ULx" "ULx" "ULx" "ULx" "ULx"] -> w351
                tunnel: [-5.0 ("min") -5.0 ("min") -5.0 ("min") "min" "min"] -> w345
                tunnel: [5.0 ("max") 5.0 ("max") 5.0 ("max") "max" "max"] -> w346
                tunnel: w343 -> [_ _ _ _ _]
                frame "AI Volts", Default {
                  n247 = call-poly <vilib>:"ULx Create Virtual Channel.vi"("maximum value"="max", "minimum value"="min", "physical channels"="ULx") -> ("task out"=w375:refnum<k24>, "error out"=w365:errorcluster)  [unwired: 11 in]
                  n248 = call "TrapBlankChan.vi"("error in (no error)"=w365) -> ("error out"=w364:errorcluster)  [unwired: 9 in, 1 out]
                  n249 = call-poly <vilib>:"ULx Create Virtual Channel.vi"("task in"=w375, "maximum value"="max 2", "minimum value"="min 2", "physical channels"="physical channels 2", "error in"=w364) -> ("task out"=w374:refnum<k24>, "error out"=w363:errorcluster)  [unwired: 9 in]
                  n250 = call "TrapBlankChan.vi"("error in (no error)"=w363) -> ("error out"=w362:errorcluster)  [unwired: 9 in, 1 out]
                  n251 = call-poly <vilib>:"ULx Create Virtual Channel.vi"("task in"=w374, "maximum value"="max 3", "minimum value"="min 3", "physical channels"="physical channels 3", "error in"=w362) -> ("task out"=w358:refnum<k24>, "error out"=w361:errorcluster)  [unwired: 9 in]
                  n252 = call "TrapBlankChan.vi"("error in (no error)"=w361) -> ("message"=w360:string, "error out"=w359:errorcluster)  [unwired: 9 in]
                }
                frame "AI Cur" {
                  n253 = call-poly <vilib>:"ULx Create Virtual Channel.vi"("maximum value"="max", "minimum value"="min", "physical channels"="ULx") -> ("task out"=w396:refnum<k24>, "error out"=w393:errorcluster)  [unwired: 11 in]
                  n254 = call "TrapBlankChan.vi"("error in (no error)"=w393) -> ("error out"=w392:errorcluster)  [unwired: 9 in, 1 out]
                  n255 = call-poly <vilib>:"ULx Create Virtual Channel.vi"("task in"=w396, "maximum value"="max 4", "minimum value"="min 4", "physical channels"="physical channels 5", "error in"=w392) -> ("task out"=w395:refnum<k24>, "error out"=w391:errorcluster)  [unwired: 9 in]
                  n256 = call "TrapBlankChan.vi"("error in (no error)"=w391) -> ("error out"=w390:errorcluster)  [unwired: 9 in, 1 out]
                  n257 = call-poly <vilib>:"ULx Create Virtual Channel.vi"("task in"=w395, "maximum value"="max 5", "minimum value"="min 5", "physical channels"="physical channels 6", "error in"=w390) -> ("task out"=w394:refnum<k24>, "error out"=w389:errorcluster)  [unwired: 9 in]
                  n258 = call "TrapBlankChan.vi"("error in (no error)"=w389) -> ("message"=w387:string, "error out"=w388:errorcluster)  [unwired: 9 in]
                }
                frame "AI Temp" {
                  n259 = call-poly <vilib>:"ULx Create Virtual Channel.vi"("physical channels"="ULx", "units"="units") -> ("task out"=w414:refnum<k24>, "error out"=w411:errorcluster)  [unwired: 12 in]
                  n260 = call "TrapBlankChan.vi"("error in (no error)"=w411) -> ("error out"=w410:errorcluster)  [unwired: 9 in, 1 out]
                  n261 = call-poly <vilib>:"ULx Create Virtual Channel.vi"("task in"=w414, "physical channels"="physical channels 8", "units"="units 2", "error in"=w410) -> ("task out"=w413:refnum<k24>, "error out"=w409:errorcluster)  [unwired: 10 in]
                  n262 = call "TrapBlankChan.vi"("error in (no error)"=w409) -> ("error out"=w408:errorcluster)  [unwired: 9 in, 1 out]
                  n263 = call-poly <vilib>:"ULx Create Virtual Channel.vi"("task in"=w413, "physical channels"="physical channels 9", "units"="units 3", "error in"=w408) -> ("task out"=w412:refnum<k24>, "error out"=w407:errorcluster)  [unwired: 10 in]
                  n264 = call "TrapBlankChan.vi"("error in (no error)"=w407) -> ("message"=w405:string, "error out"=w406:errorcluster)  [unwired: 9 in]
                }
                frame "AO Volts" {
                  n265 = call-poly <vilib>:"ULx Create Virtual Channel.vi"("maximum value"="max", "minimum value"="min", "physical channels"="ULx") -> ("task out"=w433:refnum<k24>, "error out"=w430:errorcluster)  [unwired: 11 in]
                  n266 = call "TrapBlankChan.vi"("error in (no error)"=w430) -> ("error out"=w429:errorcluster)  [unwired: 9 in, 1 out]
                  n267 = call-poly <vilib>:"ULx Create Virtual Channel.vi"("task in"=w433, "maximum value"="max 8", "minimum value"="min 8", "physical channels"="physical channels 11", "error in"=w429) -> ("task out"=w432:refnum<k24>, "error out"=w428:errorcluster)  [unwired: 9 in]
                  n268 = call "TrapBlankChan.vi"("error in (no error)"=w428) -> ("error out"=w427:errorcluster)  [unwired: 9 in, 1 out]
                  n269 = call-poly <vilib>:"ULx Create Virtual Channel.vi"("task in"=w432, "maximum value"="max 7", "minimum value"="min 7", "physical channels"="physical channels 12", "error in"=w427) -> ("task out"=w431:refnum<k24>, "error out"=w426:errorcluster)  [unwired: 9 in]
                  n270 = call "TrapBlankChan.vi"("error in (no error)"=w426) -> ("message"=w424:string, "error out"=w425:errorcluster)  [unwired: 9 in]
                }
                frame "AO Cur" {
                  n271 = call-poly <vilib>:"ULx Create Virtual Channel.vi"("maximum value"="max", "minimum value"="min", "physical channels"="ULx") -> ("task out"=w452:refnum<k24>, "error out"=w449:errorcluster)  [unwired: 11 in]
                  n272 = call "TrapBlankChan.vi"("error in (no error)"=w449) -> ("error out"=w448:errorcluster)  [unwired: 9 in, 1 out]
                  n273 = call-poly <vilib>:"ULx Create Virtual Channel.vi"("task in"=w452, "maximum value"="max 11", "minimum value"="min 11", "physical channels"="physical channels 14", "error in"=w448) -> ("task out"=w451:refnum<k24>, "error out"=w447:errorcluster)  [unwired: 9 in]
                  n274 = call "TrapBlankChan.vi"("error in (no error)"=w447) -> ("error out"=w446:errorcluster)  [unwired: 9 in, 1 out]
                  n275 = call-poly <vilib>:"ULx Create Virtual Channel.vi"("task in"=w451, "maximum value"="max 10", "minimum value"="min 10", "physical channels"="physical channels 15", "error in"=w446) -> ("task out"=w450:refnum<k24>, "error out"=w445:errorcluster)  [unwired: 9 in]
                  n276 = call "TrapBlankChan.vi"("error in (no error)"=w445) -> ("message"=w443:string, "error out"=w444:errorcluster)  [unwired: 9 in]
                }
              }
              n277 = Multiply(x=w346, y=1.01) -> (x*y=w348:dbl)
              n278 = Multiply(x=1.01, y=w345) -> (x*y=w347:dbl)
              n279 = property on="data 2" class="Slide (strict)"("Scale.Maximum"=w348) -> ()  [unwired: 2 in, 2 out]
              n280 = property on="data 2" class="Slide (strict)"("Scale.Minimum"=w347) -> ()  [unwired: 2 in, 2 out]
            }
            frame "Digital" {
              n281 = case shown="\"Digital Output\"" "DigitalType" {
                tunnel: [w466 w480] -> w455
                tunnel: [w465 w481] -> w456
                tunnel: [w464 w487] -> w457
                tunnel: ["ULx" "ULx"] -> w454
                frame "Digital Input", Default {
                  n282 = call-poly <vilib>:"ULx Create Virtual Channel.vi"("lines"="ULx", "line grouping"="line grouping") -> ("task out"=w473:refnum<k24>, "error out"=w471:errorcluster)  [unwired: 12 in]
                  n283 = call "TrapBlankChan.vi"("error in (no error)"=w471) -> ("error out"=w470:errorcluster)  [unwired: 9 in, 1 out]
                  n284 = call-poly <vilib>:"ULx Create Virtual Channel.vi"("task in"=w473, "lines"="lines 2", "line grouping"="line grouping 2", "error in"=w470) -> ("task out"=w472:refnum<k24>, "error out"=w469:errorcluster)  [unwired: 10 in]
                  n285 = call "TrapBlankChan.vi"("error in (no error)"=w469) -> ("error out"=w468:errorcluster)  [unwired: 9 in, 1 out]
                  n286 = call-poly <vilib>:"ULx Create Virtual Channel.vi"("task in"=w472, "lines"="lines 3", "line grouping"="line grouping 3", "error in"=w468) -> ("task out"=w464:refnum<k24>, "error out"=w467:errorcluster)  [unwired: 10 in]
                  n287 = call "TrapBlankChan.vi"("error in (no error)"=w467) -> ("message"=w466:string, "error out"=w465:errorcluster)  [unwired: 9 in]
                }
                frame "Digital Output" {
                  n288 = call-poly <vilib>:"ULx Create Virtual Channel.vi"("lines"="ULx", "line grouping"="line grouping") -> ("task out"=w489:refnum<k24>, "error out"=w486:errorcluster)  [unwired: 12 in]
                  n289 = call "TrapBlankChan.vi"("error in (no error)"=w486) -> ("error out"=w485:errorcluster)  [unwired: 9 in, 1 out]
                  n290 = call-poly <vilib>:"ULx Create Virtual Channel.vi"("task in"=w489, "lines"="lines 5", "line grouping"="line grouping 5", "error in"=w485) -> ("task out"=w488:refnum<k24>, "error out"=w484:errorcluster)  [unwired: 10 in]
                  n291 = call "TrapBlankChan.vi"("error in (no error)"=w484) -> ("error out"=w483:errorcluster)  [unwired: 9 in, 1 out]
                  n292 = call-poly <vilib>:"ULx Create Virtual Channel.vi"("task in"=w488, "lines"="lines 6", "line grouping"="line grouping 6", "error in"=w483) -> ("task out"=w487:refnum<k24>, "error out"=w482:errorcluster)  [unwired: 10 in]
                  n293 = call "TrapBlankChan.vi"("error in (no error)"=w482) -> ("message"=w480:string, "error out"=w481:errorcluster)  [unwired: 9 in]
                }
              }
            }
            frame "Counter" {
              n294 = case shown="\"Position In\"" "CounterType" {
                tunnel: [w509 w529 w551 w575 w589 w608 w627] -> w493
                tunnel: [w508 w530 w552 w576 w590 w609 w628] -> w494
                tunnel: [w507 w536 w558 w579 w596 w610 w629] -> w492
                tunnel: ["ULx" "ULx" "ULx" "ULx" "ULx" "ULx" "ULx"] -> w491
                frame "Freq In", Default {
                  n295 = call-poly <vilib>:"ULx Create Virtual Channel.vi"("counters"="ULx", "units"="units", "starting edge"="starting edge", "measurement time"="measure time") -> ("task out"=w516:refnum<k24>, "error out"=w514:errorcluster)  [unwired: 10 in]
                  n296 = call "TrapBlankChan.vi"("error in (no error)"=w514) -> ("error out"=w513:errorcluster)  [unwired: 9 in, 1 out]
                  n297 = call-poly <vilib>:"ULx Create Virtual Channel.vi"("task in"=w516, "counters"="counters 2", "units"="units 5", "error in"=w513, "starting edge"="starting edge 2", "measurement time"="measure time 2") -> ("task out"=w515:refnum<k24>, "error out"=w512:errorcluster)  [unwired: 8 in]
                  n298 = call "TrapBlankChan.vi"("error in (no error)"=w512) -> ("error out"=w511:errorcluster)  [unwired: 9 in, 1 out]
                  n299 = call-poly <vilib>:"ULx Create Virtual Channel.vi"("task in"=w515, "counters"="counters 3", "units"="units 6", "error in"=w511, "starting edge"="starting edge 3", "measurement time"="measure time 3") -> ("task out"=w507:refnum<k24>, "error out"=w510:errorcluster)  [unwired: 8 in]
                  n300 = call "TrapBlankChan.vi"("error in (no error)"=w510) -> ("message"=w509:string, "error out"=w508:errorcluster)  [unwired: 9 in]
                }
                frame "Period In" {
                  n301 = call-poly <vilib>:"ULx Create Virtual Channel.vi"("counters"="ULx", "units"="units", "starting edge"="starting edge", "measurement time"="measure time") -> ("task out"=w538:refnum<k24>, "error out"=w535:errorcluster)  [unwired: 10 in]
                  n302 = call "TrapBlankChan.vi"("error in (no error)"=w535) -> ("error out"=w534:errorcluster)  [unwired: 9 in, 1 out]
                  n303 = call-poly <vilib>:"ULx Create Virtual Channel.vi"("task in"=w538, "counters"="counters 5", "units"="units 8", "error in"=w534, "starting edge"="starting edge 5", "measurement time"="measure time 4") -> ("task out"=w537:refnum<k24>, "error out"=w533:errorcluster)  [unwired: 8 in]
                  n304 = call "TrapBlankChan.vi"("error in (no error)"=w533) -> ("error out"=w532:errorcluster)  [unwired: 9 in, 1 out]
                  n305 = call-poly <vilib>:"ULx Create Virtual Channel.vi"("task in"=w537, "counters"="counters 6", "units"="units 9", "error in"=w532, "starting edge"="starting edge 6", "measurement time"="measure time 5") -> ("task out"=w536:refnum<k24>, "error out"=w531:errorcluster)  [unwired: 8 in]
                  n306 = call "TrapBlankChan.vi"("error in (no error)"=w531) -> ("message"=w529:string, "error out"=w530:errorcluster)  [unwired: 9 in]
                }
                frame "Edge In" {
                  n307 = call-poly <vilib>:"ULx Create Virtual Channel.vi"("initial count"="initial count", "count direction"="direction", "edge"="edge", "counters"="ULx") -> ("task out"=w560:refnum<k24>, "error out"=w557:errorcluster)  [unwired: 10 in]
                  n308 = call "TrapBlankChan.vi"("error in (no error)"=w557) -> ("error out"=w556:errorcluster)  [unwired: 9 in, 1 out]
                  n309 = call-poly <vilib>:"ULx Create Virtual Channel.vi"("task in"=w560, "initial count"="initial count 2", "count direction"="direction 2", "edge"="edge 2", "counters"="counters 8", "error in"=w556) -> ("task out"=w559:refnum<k24>, "error out"=w555:errorcluster)  [unwired: 8 in]
                  n310 = call "TrapBlankChan.vi"("error in (no error)"=w555) -> ("error out"=w554:errorcluster)  [unwired: 9 in, 1 out]
                  n311 = call-poly <vilib>:"ULx Create Virtual Channel.vi"("task in"=w559, "initial count"="initial count 3", "count direction"="direction 3", "edge"="edge 3", "counters"="counters 9", "error in"=w554) -> ("task out"=w558:refnum<k24>, "error out"=w553:errorcluster)  [unwired: 8 in]
                  n312 = call "TrapBlankChan.vi"("error in (no error)"=w553) -> ("message"=w551:string, "error out"=w552:errorcluster)  [unwired: 9 in]
                }
                frame "Position In" {
                  n313 = call-poly <vilib>:"ULx Create Virtual Channel.vi"("decoding type"="type", "pulses per revolution"="pulses per", "initial angle"="initial angle\npulses per", "counters"="ULx", "units"="units 10", "z index mode"="index mode") -> ("task out"=w573:refnum<k24>, "error out"=w578:errorcluster)  [unwired: 8 in]
                  n314 = call "TrapBlankChan.vi"("error in (no error)"=w578) -> ("error out"=w574:errorcluster)  [unwired: 9 in, 1 out]
                  n315 = call-poly <vilib>:"ULx Create Virtual Channel.vi"("task in"=w573, "decoding type"="type 2", "pulses per revolution"="pulses per 2", "initial angle"="initial angle\npulses per", "counters"="counters 11", "units"="units 11", "error in"=w574, "z index mode"="index mode 2") -> ("task out"=w579:refnum<k24>, "error out"=w577:errorcluster)  [unwired: 6 in]
                  n316 = call "TrapBlankChan.vi"("error in (no error)"=w577) -> ("message"=w575:string, "error out"=w576:errorcluster)  [unwired: 9 in]
                }
                frame "Freq Out" {
                  n317 = call-poly <vilib>:"ULx Create Virtual Channel.vi"("frequency"="frequency", "duty cycle"="duty cycle", "counters"="ULx") -> ("task out"=w598:refnum<k24>, "error out"=w595:errorcluster)  [unwired: 11 in]
                  n318 = call "TrapBlankChan.vi"("error in (no error)"=w595) -> ("error out"=w594:errorcluster)  [unwired: 9 in, 1 out]
                  n319 = call-poly <vilib>:"ULx Create Virtual Channel.vi"("task in"=w598, "frequency"="frequency 2", "duty cycle"="duty cycle 2", "counters"="counters 13", "error in"=w594) -> ("task out"=w597:refnum<k24>, "error out"=w593:errorcluster)  [unwired: 9 in]
                  n320 = call "TrapBlankChan.vi"("error in (no error)"=w593) -> ("error out"=w592:errorcluster)  [unwired: 9 in, 1 out]
                  n321 = call-poly <vilib>:"ULx Create Virtual Channel.vi"("task in"=w597, "frequency"="frequency 3", "duty cycle"="duty cycle 3", "counters"="counters 14", "error in"=w592) -> ("task out"=w596:refnum<k24>, "error out"=w591:errorcluster)  [unwired: 9 in]
                  n322 = call "TrapBlankChan.vi"("error in (no error)"=w591) -> ("message"=w589:string, "error out"=w590:errorcluster)  [unwired: 9 in]
                }
                frame "Time Out" {
                  n323 = call-poly <vilib>:"ULx Create Virtual Channel.vi"("high time"="high time", "low time"="low time", "counters"="ULx") -> ("task out"=w617:refnum<k24>, "error out"=w615:errorcluster)  [unwired: 11 in]
                  n324 = call "TrapBlankChan.vi"("error in (no error)"=w615) -> ("error out"=w614:errorcluster)  [unwired: 9 in, 1 out]
                  n325 = call-poly <vilib>:"ULx Create Virtual Channel.vi"("task in"=w617, "high time"="high time 2", "low time"="low time 2", "counters"="counters 18", "error in"=w614) -> ("task out"=w616:refnum<k24>, "error out"=w613:errorcluster)  [unwired: 9 in]
                  n326 = call "TrapBlankChan.vi"("error in (no error)"=w613) -> ("error out"=w612:errorcluster)  [unwired: 9 in, 1 out]
                  n327 = call-poly <vilib>:"ULx Create Virtual Channel.vi"("task in"=w616, "high time"="high time 3", "low time"="low time 3", "counters"="counters 19", "error in"=w612) -> ("task out"=w610:refnum<k24>, "error out"=w611:errorcluster)  [unwired: 9 in]
                  n328 = call "TrapBlankChan.vi"("error in (no error)"=w611) -> ("message"=w608:string, "error out"=w609:errorcluster)  [unwired: 9 in]
                }
                frame "Ticks Out" {
                  n329 = call-poly <vilib>:"ULx Create Virtual Channel.vi"("high ticks"="high ticks", "low ticks"="low ticks", "counters"="ULx") -> ("task out"=w636:refnum<k24>, "error out"=w634:errorcluster)  [unwired: 11 in]
                  n330 = call "TrapBlankChan.vi"("error in (no error)"=w634) -> ("error out"=w633:errorcluster)  [unwired: 9 in, 1 out]
                  n331 = call-poly <vilib>:"ULx Create Virtual Channel.vi"("task in"=w636, "high ticks"="high ticks 2", "low ticks"="low ticks 2", "counters"="counters 16", "error in"=w633) -> ("task out"=w635:refnum<k24>, "error out"=w632:errorcluster)  [unwired: 9 in]
                  n332 = call "TrapBlankChan.vi"("error in (no error)"=w632) -> ("error out"=w631:errorcluster)  [unwired: 9 in, 1 out]
                  n333 = call-poly <vilib>:"ULx Create Virtual Channel.vi"("task in"=w635, "high ticks"="high ticks 3", "low ticks"="low ticks 3", "counters"="counters 20", "error in"=w631) -> ("task out"=w629:refnum<k24>, "error out"=w630:errorcluster)  [unwired: 9 in]
                  n334 = call "TrapBlankChan.vi"("error in (no error)"=w630) -> ("message"=w627:string, "error out"=w628:errorcluster)  [unwired: 9 in]
                }
              }
            }
            frame "Composite In" {
              n335 = stacked-sequence {
                seq-local: [w649 _ _ _ _ _] -> [_ w670 _ _ _ _]
                seq-local: [w648 _ _ _ _ _] -> [_ w669 _ _ _ _]
                seq-local: [_ w668 _ _ _ _] -> [_ _ w684 _ _ _]
                seq-local: [_ w667 _ _ _ _] -> [_ _ w681 _ _ _]
                seq-local: [_ _ w683 _ _ _] -> [_ _ _ w711 _ _]
                seq-local: [_ _ w682 _ _ _] -> [_ _ _ w710 _ _]
                seq-local: [_ _ _ w709 _ _] -> [_ _ _ _ w719 _]
                seq-local: [_ _ _ w708 _ _] -> [_ _ _ _ w721 _]
                seq-local: [_ _ _ _ w719 _] -> [_ _ _ _ _ w730]
                seq-local: [_ _ _ _ w725 _] -> [_ _ _ _ _ w729]
                seq-local: ["ULx" _ _ _ _ _] -> [_ w660 _ _ _ _]
                seq-local: [_ w659 _ _ _ _] -> [_ _ w679 _ _ _]
                seq-local: [_ _ w678 _ _ _] -> [_ _ _ w696 _ _]
                seq-local: [_ _ _ w694 _ _] -> [_ _ _ _ w724 _]
                seq-local: [_ _ _ _ w722 _] -> [_ _ _ _ _ w727]
                tunnel: [_ _ _ _ _ w731] -> w640
                tunnel: [_ _ _ _ _ w732] -> w639
                tunnel: [_ _ _ _ _ w733] -> w638
                tunnel: [_ _ _ _ _ w726] -> w637
                frame #0 {
                  # "Composite Analog Input"
                  n336 = call-poly <vilib>:"ULx Create Virtual Channel.vi"("maximum value"="max", "minimum value"="min", "physical channels"="ULx") -> ("task out"=w658:refnum<k24>, "error out"=w656:errorcluster)  [unwired: 11 in]
                  n337 = call "TrapBlankChan.vi"("error in (no error)"=w656) -> ("error out"=w655:errorcluster)  [unwired: 9 in, 1 out]
                  n338 = call-poly <vilib>:"ULx Create Virtual Channel.vi"("task in"=w658, "maximum value"="max 9", "minimum value"="min 9", "physical channels"="physical channels 17", "error in"=w655) -> ("task out"=w657:refnum<k24>, "error out"=w654:errorcluster)  [unwired: 9 in]
                  n339 = call "TrapBlankChan.vi"("error in (no error)"=w654) -> ("error out"=w653:errorcluster)  [unwired: 9 in, 1 out]
                  n340 = call-poly <vilib>:"ULx Create Virtual Channel.vi"("task in"=w657, "maximum value"="max 12", "minimum value"="min 12", "physical channels"="physical channels 18", "error in"=w653) -> ("task out"=w649:refnum<k24>, "error out"=w652:errorcluster)  [unwired: 9 in]
                  n341 = call "TrapBlankChan.vi"("error in (no error)"=w652) -> ("error out"=w648:errorcluster)  [unwired: 9 in, 1 out]
                }
                frame #1 {
                  # "Composite Temperature Input"
                  n342 = call "StringJoiner.vi"("string 2"="ULx", "string 1"=w660) -> ("concatenated string"=w659:string)
                  n343 = call-poly <vilib>:"ULx Create Virtual Channel.vi"("task in"=w670, "physical channels"="ULx", "units"="units", "error in"=w669) -> ("task out"=w677:refnum<k24>, "error out"=w675:errorcluster)  [unwired: 10 in]
                  n344 = call "TrapBlankChan.vi"("error in (no error)"=w675) -> ("error out"=w674:errorcluster)  [unwired: 9 in, 1 out]
                  n345 = call-poly <vilib>:"ULx Create Virtual Channel.vi"("task in"=w677, "physical channels"="physical channels 20", "units"="units 7", "error in"=w674) -> ("task out"=w676:refnum<k24>, "error out"=w673:errorcluster)  [unwired: 10 in]
                  n346 = call "TrapBlankChan.vi"("error in (no error)"=w673) -> ("error out"=w672:errorcluster)  [unwired: 9 in, 1 out]
                  n347 = call-poly <vilib>:"ULx Create Virtual Channel.vi"("task in"=w676, "physical channels"="physical channels 21", "units"="units 12", "error in"=w672) -> ("task out"=w668:refnum<k24>, "error out"=w671:errorcluster)  [unwired: 10 in]
                  n348 = call "TrapBlankChan.vi"("error in (no error)"=w671) -> ("error out"=w667:errorcluster)  [unwired: 9 in, 1 out]
                }
                frame #2 {
                  # "Composite Digital Input"
                  n349 = call "StringJoiner.vi"("string 2"="ULx", "string 1"=w679) -> ("concatenated string"=w678:string)
                  n350 = call-poly <vilib>:"ULx Create Virtual Channel.vi"("task in"=w684, "ports"="ULx", "error in"=w681) -> ("task out"=w693:refnum<k24>, "error out"=w691:errorcluster)  [unwired: 11 in]
                  n351 = call "TrapBlankChan.vi"("error in (no error)"=w691) -> ("error out"=w690:errorcluster)  [unwired: 9 in, 1 out]
                  n352 = call-poly <vilib>:"ULx Create Virtual Channel.vi"("task in"=w693, "ports"="ports 2", "error in"=w690) -> ("task out"=w692:refnum<k24>, "error out"=w689:errorcluster)  [unwired: 11 in]
                  n353 = call "TrapBlankChan.vi"("error in (no error)"=w689) -> ("error out"=w688:errorcluster)  [unwired: 9 in, 1 out]
                  n354 = call-poly <vilib>:"ULx Create Virtual Channel.vi"("task in"=w692, "ports"="ports 3", "error in"=w688) -> ("task out"=w683:refnum<k24>, "error out"=w687:errorcluster)  [unwired: 11 in]
                  n355 = call "TrapBlankChan.vi"("error in (no error)"=w687) -> ("error out"=w682:errorcluster)  [unwired: 9 in, 1 out]
                }
                frame #3 {
                  # "Composite Counter Edge Input"
                  n356 = call "StringJoiner.vi"("string 2"="ULx", "string 1"=w696) -> ("concatenated string"=w694:string)
                  n357 = call-poly <vilib>:"ULx Create Virtual Channel.vi"("task in"=w711, "initial count"="initial count", "count direction"="direction", "edge"="edge", "counters"="ULx", "error in"=w710) -> ("task out"=w718:refnum<k24>, "error out"=w716:errorcluster)  [unwired: 8 in]
                  n358 = call "TrapBlankChan.vi"("error in (no error)"=w716) -> ("error out"=w715:errorcluster)  [unwired: 9 in, 1 out]
                  n359 = call-poly <vilib>:"ULx Create Virtual Channel.vi"("task in"=w718, "initial count"="initial count 5", "count direction"="direction 5", "edge"="edge 5", "counters"="counters 22", "error in"=w715) -> ("task out"=w717:refnum<k24>, "error out"=w714:errorcluster)  [unwired: 8 in]
                  n360 = call "TrapBlankChan.vi"("error in (no error)"=w714) -> ("error out"=w713:errorcluster)  [unwired: 9 in, 1 out]
                  n361 = call-poly <vilib>:"ULx Create Virtual Channel.vi"("task in"=w717, "initial count"="initial count 6", "count direction"="direction 6", "edge"="edge 6", "counters"="counters 23", "error in"=w713) -> ("task out"=w709:refnum<k24>, "error out"=w712:errorcluster)  [unwired: 8 in]
                  n362 = call "TrapBlankChan.vi"("error in (no error)"=w712) -> ("error out"=w708:errorcluster)  [unwired: 9 in, 1 out]
                }
                frame #4 {
                  # "Composite Encoder Input"
                  n363 = call "StringJoiner.vi"("string 2"="ULx", "string 1"=w724) -> ("concatenated string"=w722:string)
                  n364 = call "TrapBlankChan.vi"("error in (no error)"=w721) -> ("error out"=w720:errorcluster)  [unwired: 9 in, 1 out]
                  n365 = call "TrapBlankChan.vi"("error in (no error)"=w720) -> ("error out"=w725:errorcluster)  [unwired: 9 in, 1 out]
                }
                frame #5 {
                  n366 = call "StringJoiner.vi"("string 2"="ULx", "string 1"=w727) -> ("concatenated string"=w726:string)
                  n367 = call-poly <vilib>:"ULx Create Virtual Channel.vi"("task in"=w730, "maximum value"="max", "minimum value"="min", "physical channels"="ULx", "error in"=w729) -> ("task out"=w748:refnum<k24>, "error out"=w746:errorcluster)  [unwired: 9 in]
                  n368 = call "TrapBlankChan.vi"("error in (no error)"=w746) -> ("error out"=w745:errorcluster)  [unwired: 9 in, 1 out]
                  n369 = call-poly <vilib>:"ULx Create Virtual Channel.vi"("task in"=w748, "maximum value"="max 15", "minimum value"="min 15", "physical channels"="physical channels 29", "error in"=w745) -> ("task out"=w747:refnum<k24>, "error out"=w744:errorcluster)  [unwired: 9 in]
                  n370 = call "TrapBlankChan.vi"("error in (no error)"=w744) -> ("error out"=w743:errorcluster)  [unwired: 9 in, 1 out]
                  n371 = call-poly <vilib>:"ULx Create Virtual Channel.vi"("task in"=w747, "maximum value"="max 18", "minimum value"="min 18", "physical channels"="physical channels 30", "error in"=w743) -> ("task out"=w733:refnum<k24>, "error out"=w742:errorcluster)  [unwired: 9 in]
                  n372 = call "TrapBlankChan.vi"("error in (no error)"=w742) -> ("message"=w731:string, "error out"=w732:errorcluster)  [unwired: 9 in]
                }
              }
            }
            frame "Composite Out" {
              n373 = stacked-sequence {
                seq-local: [w763 _ _] -> [_ w779 _]
                seq-local: [w762 _ _] -> [_ w778 _]
                seq-local: [_ w777 _] -> [_ _ w794]
                seq-local: [_ w776 _] -> [_ _ w793]
                seq-local: ["ULx" _ _] -> [_ w773 _]
                seq-local: [_ w771 _] -> [_ _ w789]
                tunnel: [_ _ w792] -> w750
                tunnel: [_ _ w791] -> w752
                tunnel: [_ _ w790] -> w751
                tunnel: [_ _ w787] -> w749
                frame #0 {
                  # "Composite Analog Output"
                  n374 = call-poly <vilib>:"ULx Create Virtual Channel.vi"("maximum value"="max", "minimum value"="min", "physical channels"="ULx") -> ("task out"=w770:refnum<k24>, "error out"=w768:errorcluster)  [unwired: 11 in]
                  n375 = call "TrapBlankChan.vi"("error in (no error)"=w768) -> ("error out"=w767:errorcluster)  [unwired: 9 in, 1 out]
                  n376 = call-poly <vilib>:"ULx Create Virtual Channel.vi"("task in"=w770, "maximum value"="max 13", "minimum value"="min 13", "physical channels"="physical channels 23", "error in"=w767) -> ("task out"=w769:refnum<k24>, "error out"=w766:errorcluster)  [unwired: 9 in]
                  n377 = call "TrapBlankChan.vi"("error in (no error)"=w766) -> ("error out"=w765:errorcluster)  [unwired: 9 in, 1 out]
                  n378 = call-poly <vilib>:"ULx Create Virtual Channel.vi"("task in"=w769, "maximum value"="max 14", "minimum value"="min 14", "physical channels"="physical channels 24", "error in"=w765) -> ("task out"=w763:refnum<k24>, "error out"=w764:errorcluster)  [unwired: 9 in]
                  n379 = call "TrapBlankChan.vi"("error in (no error)"=w764) -> ("error out"=w762:errorcluster)  [unwired: 9 in, 1 out]
                }
                frame #1 {
                  # "Composite Digital Output"
                  n380 = call "StringJoiner.vi"("string 2"="ULx", "string 1"=w773) -> ("concatenated string"=w771:string)
                  n381 = call-poly <vilib>:"ULx Create Virtual Channel.vi"("task in"=w779, "ports"="ULx", "error in"=w778) -> ("task out"=w786:refnum<k24>, "error out"=w784:errorcluster)  [unwired: 11 in]
                  n382 = call "TrapBlankChan.vi"("error in (no error)"=w784) -> ("error out"=w783:errorcluster)  [unwired: 9 in, 1 out]
                  n383 = call-poly <vilib>:"ULx Create Virtual Channel.vi"("task in"=w786, "ports"="ports 5", "error in"=w783) -> ("task out"=w785:refnum<k24>, "error out"=w782:errorcluster)  [unwired: 11 in]
                  n384 = call "TrapBlankChan.vi"("error in (no error)"=w782) -> ("error out"=w781:errorcluster)  [unwired: 9 in, 1 out]
                  n385 = call-poly <vilib>:"ULx Create Virtual Channel.vi"("task in"=w785, "ports"="ports 6", "error in"=w781) -> ("task out"=w777:refnum<k24>, "error out"=w780:errorcluster)  [unwired: 11 in]
                  n386 = call "TrapBlankChan.vi"("error in (no error)"=w780) -> ("error out"=w776:errorcluster)  [unwired: 9 in, 1 out]
                }
                frame #2 {
                  # "Repeat Composite Analog Output"
                  n387 = call "StringJoiner.vi"("string 2"="ULx", "string 1"=w789) -> ("concatenated string"=w787:string)
                  n388 = call-poly <vilib>:"ULx Create Virtual Channel.vi"("task in"=w794, "maximum value"="max", "minimum value"="min", "physical channels"="ULx", "error in"=w793) -> ("task out"=w809:refnum<k24>, "error out"=w807:errorcluster)  [unwired: 9 in]
                  n389 = call "TrapBlankChan.vi"("error in (no error)"=w807) -> ("error out"=w806:errorcluster)  [unwired: 9 in, 1 out]
                  n390 = call-poly <vilib>:"ULx Create Virtual Channel.vi"("task in"=w809, "maximum value"="max 16", "minimum value"="min 16", "physical channels"="physical channels 26", "error in"=w806) -> ("task out"=w808:refnum<k24>, "error out"=w805:errorcluster)  [unwired: 9 in]
                  n391 = call "TrapBlankChan.vi"("error in (no error)"=w805) -> ("error out"=w804:errorcluster)  [unwired: 9 in, 1 out]
                  n392 = call-poly <vilib>:"ULx Create Virtual Channel.vi"("task in"=w808, "maximum value"="max 17", "minimum value"="min 17", "physical channels"="physical channels 27", "error in"=w804) -> ("task out"=w792:refnum<k24>, "error out"=w803:errorcluster)  [unwired: 9 in]
                  n393 = call "TrapBlankChan.vi"("error in (no error)"=w803) -> ("message"=w790:string, "error out"=w791:errorcluster)  [unwired: 9 in]
                }
              }
            }
          }
          n394 = local write "Active Channels"(w332) -> ()
          n395 = case shown="Error" w338 {
            selector: w338 -> [w813 w816]
            tunnel: [w813 w816] -> w340
            tunnel: w337 -> [_ w815]
            frame No Error {
            }
            frame Error {
              n396 = local write "Plots and Errors"(enum32{"Error", "Plots"}."Error" ("Plots and Errors")) -> ()
              "message 2" <- w815
            }
          }
          n397 = for {
            N: 5 -> [_]
            tunnel: w335 -> [w811]
            tunnel: [FALSE] -> w334
            n398 = Wait Until Next ms Multiple(millisecond multiple=w811) -> ()  [unwired: 1 out]
            "CreateChans" <- TRUE
          }
          n399 = local write "CreateChans"(w334) -> ()
        }
        frame 3 {
          # "Channel Info"
          n400 = Not Equal?(x="", y="Active Channels") -> (x != y?=w822:bool)
          n401 = case shown="True" w822 {
            tunnel: w829 -> [w835 w840]
            tunnel: w828 -> [w834 w839]
            tunnel: [w835 w838] -> w827
            tunnel: [w834 w837] -> w821
            tunnel: w826 -> [_ _]
            tunnel: "Active Channels" -> [_ w836]
            frame False {
            }
            frame True {
              n402 = call "SetActiveChans.vi"("error in (no error)"=w839, "ActiveChannels"=w836, "task in"=w840) -> ("error out"=w837:errorcluster, "task out"=w838:refnum<k24>)
            }
          }
          n403 = local read "SelLib"() -> (w830:enum32{"ULx", "DAQMx"})
          n404 = case shown="\"ULx\", Default" w830 {
            tunnel: w827 -> [w846]
            tunnel: [w844] -> w831
            tunnel: w821 -> [w843]
            tunnel: [w842] -> w819
            tunnel: [w841] -> w820
            frame "ULx", Default {
              n405 = call "ULxTaskInfo.vi"("task in"=w846, "error in (no error)"=w843) -> ("task in 2"=w841:refnum<k24>, "Task"=w845:i32, "error out"=w842:errorcluster)  [unwired: 2 out]
              n406 = Number To Hexadecimal String(2:w845) -> (0:w844:string)  [unwired: 1 in]
            }
          }
          "String" <- w831
          n407 = call "ULxTaskInfo.vi"("task in"=w820, "error in (no error)"=w819) -> ("task in 2"=w818:refnum<k24>, "ToString"=→"ToString":string, "Task"=→"Task":i32, "error out"=w817:errorcluster, "NumberOfChannels"=→"NumberOfChannels":u32)
        }
        frame 4 {
          # "TIMING"
          n408 = for {
            N: 5 -> [_]
            tunnel: w849 -> [w859]
            tunnel: [FALSE] -> w848
            n409 = Wait Until Next ms Multiple(millisecond multiple=w859) -> ()  [unwired: 1 out]
            "Timing" <- TRUE
          }
          n410 = local write "Timing"(w848) -> ()
          n411 = case shown="\"Clock\", Default" "Tab Control" {
            tunnel: w854 -> [w868 w874 w880]
            tunnel: w853 -> [w867 w873 w879]
            tunnel: [w866 w872 w878] -> w852
            tunnel: [w865 w871 w877] -> w851
            tunnel: w855 -> [_ _ _]
            frame "Clock", Default {
              n412 = call-poly <vilib>:"ULx Timing.vi"("task in"=w868, "sample mode"="sample mode", "samples per channel"="samples per", "rate"="rate", "clock source"="clock source", "error in"=w867) -> ("task out"=w866:refnum<k24>, "error out"=w865:errorcluster)  [unwired: 8 in]
            }
            frame "Waveform" {
              n413 = call-poly <vilib>:"ULx Timing.vi"("task in"=w874, "sample mode"="sample mode 3", "waveform"="waveform", "error in"=w873) -> ("task out"=w872:refnum<k24>, "error out"=w871:errorcluster)  [unwired: 10 in]
            }
            frame "Implicit" {
              n414 = call-poly <vilib>:"ULx Timing.vi"("task in"=w880, "sample mode"="sample mode", "samples per channel"="samples per channel", "error in"=w879) -> ("task out"=w878:refnum<k24>, "error out"=w877:errorcluster)  [unwired: 10 in]
            }
          }
          n415 = case shown="True" "Once" {
            frame False {
            }
            frame True {
              n416 = local write "Timing"(FALSE ("Start")) -> ()
            }
          }
        }
        frame 5 {
          # "TRIGGERING"
          n417 = for {
            N: 5 -> [_]
            tunnel: w883 -> [w897]
            tunnel: [FALSE] -> w882
            n418 = Wait Until Next ms Multiple(millisecond multiple=w897) -> ()  [unwired: 1 out]
            "Trigger" <- TRUE
          }
          n419 = case shown="\"Basic\", Default" "TrigType" {
            tunnel: [w903 w942 w974 w1022] -> w893
            tunnel: [w904 w941 w975 w1023] -> w894
            tunnel: "BasicType" -> [w902 _ _ _]
            tunnel: "GatedType" -> [_ w940 _ _]
            tunnel: "StartType" -> [_ _ w976 _]
            tunnel: "StopType" -> [_ _ _ w1024]
            tunnel: w887 -> [w901 w939 w973 w1021]
            tunnel: w886 -> [w900 w938 w972 w1020]
            tunnel: w885 -> [w899 w937 _ _]
            frame "Basic", Default {
              n420 = case shown="\"DPtrn\"" w902 {
                tunnel: [w908 w914 w920 w927 w935] -> w904
                tunnel: [w907 w913 w919 w926 w933] -> w903
                tunnel: w901 -> [w906 w912 w917 w922 w936]
                tunnel: w900 -> [w905 w911 w916 w921 w934]
                tunnel: w899 -> [_ _ _ _ _]
                frame "None", Default {
                  n421 = call-poly <vilib>:"ULx Trigger.vi"("task in"=w906, "error in"=w905) -> ("task out"=w908:refnum<k24>, "error out"=w907:errorcluster)  [unwired: 16 in]
                }
                frame "DEdge" {
                  n422 = call-poly <vilib>:"ULx Trigger.vi"("task in"=w912, "edge"="ULx edge", "error in"=w911, "pretrigger samples per channel"="pretrigger samples per channel") -> ("task out"=w914:refnum<k24>, "error out"=w913:errorcluster)  [unwired: 14 in]
                }
                frame "DLevel" {
                  n423 = call-poly <vilib>:"ULx Trigger.vi"("task in"=w917, "level"="level", "error in"=w916, "pretrigger samples per channel"="pretrigger samples per channel") -> ("task out"=w920:refnum<k24>, "error out"=w919:errorcluster)  [unwired: 14 in]
                }
                frame "AEdge" {
                  n424 = call-poly <vilib>:"ULx Trigger.vi"("task in"=w922, "slope"="slope", "level"="level", "error in"=w921, "pretrigger samples per channel"="pretrigger samples per channel") -> ("task out"=w927:refnum<k24>, "error out"=w926:errorcluster)  [unwired: 13 in]
                }
                frame "DPtrn" {
                  n425 = call-poly <vilib>:"ULx Trigger.vi"("task in"=w936, "trigger channel"="chan", "trigger sensitivity"="sensitivity", "pattern"="pattern", "mask"="mask", "error in"=w934, "pretrigger samples per channel"="pretrig samps") -> ("task out"=w935:refnum<k24>, "error out"=w933:errorcluster)  [unwired: 11 in]
                }
              }
            }
            frame "Gated" {
              n426 = case shown="\"AWindow\"" w940 {
                tunnel: [w945 w951 w957 w963 w971] -> w942
                tunnel: [w946 w950 w956 w964 w970] -> w941
                tunnel: w939 -> [w944 w948 w953 w959 w966]
                tunnel: w938 -> [w943 w947 w952 w958 w965]
                tunnel: w937 -> [_ _ _ _ _]
                frame "None", Default {
                  n427 = call-poly <vilib>:"ULx Trigger.vi"("task in"=w944, "error in"=w943) -> ("task out"=w946:refnum<k24>, "error out"=w945:errorcluster)  [unwired: 16 in]
                }
                frame "DLevel" {
                  n428 = call-poly <vilib>:"ULx Trigger.vi"("task in"=w948, "level"="Level 3", "error in"=w947) -> ("task out"=w950:refnum<k24>, "error out"=w951:errorcluster)  [unwired: 15 in]
                }
                frame "ALevel" {
                  n429 = call-poly <vilib>:"ULx Trigger.vi"("task in"=w953, "position"="position", "level"="level", "error in"=w952) -> ("task out"=w956:refnum<k24>, "error out"=w957:errorcluster)  [unwired: 14 in]
                }
                frame "AWindow" {
                  n430 = call-poly <vilib>:"ULx Trigger.vi"("task in"=w959, "When"="When", "window bottom"="bottom", "window top"="top", "error in"=w958) -> ("task out"=w964:refnum<k24>, "error out"=w963:errorcluster)  [unwired: 13 in]
                }
                frame "AHyst" {
                  n431 = call-poly <vilib>:"ULx Trigger.vi"("task in"=w966, "hysteresis"="hyst", "low threshold"="low", "high threshold"="high", "error in"=w965) -> ("task out"=w970:refnum<k24>, "error out"=w971:errorcluster)  [unwired: 13 in]
                }
              }
            }
            frame "Start" {
              n432 = case shown="\"AHdwr\"" w976 {
                tunnel: [w979 w985 w992 w1000 w1009 w1019] -> w975
                tunnel: [w980 w984 w991 w1001 w1010 w1018] -> w974
                tunnel: w973 -> [w978 w982 w987 w994 w1003 w1012]
                tunnel: w972 -> [w977 w981 w986 w993 w1002 w1011]
                frame "None", Default {
                  n433 = call-poly <vilib>:"ULx Trigger.vi"("task in"=w978, "error in"=w977) -> ("task out"=w979:refnum<k24>, "error out"=w980:errorcluster)  [unwired: 16 in]
                }
                frame "ExtTTL" {
                  n434 = call-poly <vilib>:"ULx Trigger.vi"("task in"=w982, "trigger sensitivity"="trigger sensitivity", "error in"=w981) -> ("task out"=w985:refnum<k24>, "error out"=w984:errorcluster)  [unwired: 15 in]
                }
                frame "AHdwr" {
                  n435 = call-poly <vilib>:"ULx Trigger.vi"("task in"=w987, "trigger sensitivity"="sensitivity", "level"="Level", "variance"="variance", "error in"=w986) -> ("task out"=w992:refnum<k24>, "error out"=w991:errorcluster)  [unwired: 13 in]
                }
                frame "ASftwr" {
                  n436 = call-poly <vilib>:"ULx Trigger.vi"("task in"=w994, "trigger channel"="trigger channel", "trigger sensitivity"="sensitivity", "level"="Level", "variance"="variance", "error in"=w993, "pretrigger samples per channel"="pretrigger samples") -> ("task out"=w1000:refnum<k24>, "error out"=w1001:errorcluster)  [unwired: 11 in]
                }
                frame "DPtrn" {
                  n437 = call-poly <vilib>:"ULx Trigger.vi"("task in"=w1003, "trigger channel"="trigger channel", "trigger sensitivity"="trigger sensitivity", "pattern"="level", "variance"="variance", "error in"=w1002, "pretrigger samples per channel"="pretrigger samples") -> ("task out"=w1009:refnum<k24>, "error out"=w1010:errorcluster)  [unwired: 11 in]
                }
                frame "Ctr" {
                  n438 = call-poly <vilib>:"ULx Trigger.vi"("task in"=w1012, "trigger channel"="trigger channel", "trigger sensitivity"="trigger sensitivity", "count"="level", "variance"="variance", "error in"=w1011, "pretrigger samples per channel"="pretrigger samples") -> ("task out"=w1019:refnum<k24>, "error out"=w1018:errorcluster)  [unwired: 11 in]
                }
              }
            }
            frame "Stop" {
              n439 = case shown="\"None\", Default" w1024 {
                tunnel: [w1028 w1036 w1044 w1052] -> w1023
                tunnel: [w1027 w1035 w1043 w1051] -> w1022
                tunnel: w1021 -> [w1026 w1030 w1038 w1046]
                tunnel: w1020 -> [w1025 w1029 w1037 w1045]
                frame "None", Default {
                  n440 = call-poly <vilib>:"ULx Trigger.vi"("task in"=w1026, "error in"=w1025) -> ("task out"=w1028:refnum<k24>, "error out"=w1027:errorcluster)  [unwired: 16 in]
                }
                frame "ASftwr" {
                  n441 = call-poly <vilib>:"ULx Trigger.vi"("task in"=w1030, "trigger channel"="trigger channel", "trigger sensitivity"="trigger sensitivity", "level"="level", "variance"="variance", "error in"=w1029) -> ("task out"=w1036:refnum<k24>, "error out"=w1035:errorcluster)  [unwired: 12 in]
                }
                frame "DPtrn" {
                  n442 = call-poly <vilib>:"ULx Trigger.vi"("task in"=w1038, "trigger channel"="trigger channel", "trigger sensitivity"="trigger sensitivity", "pattern"="level", "variance"="variance", "error in"=w1037) -> ("task out"=w1044:refnum<k24>, "error out"=w1043:errorcluster)  [unwired: 12 in]
                }
                frame "Ctr" {
                  n443 = call-poly <vilib>:"ULx Trigger.vi"("task in"=w1046, "trigger channel"="trigger channel", "trigger sensitivity"="trigger sensitivity", "count"="level", "variance"="variance", "error in"=w1045) -> ("task out"=w1052:refnum<k24>, "error out"=w1051:errorcluster)  [unwired: 12 in]
                }
              }
            }
          }
          n444 = local write "Trigger"(w882) -> ()
          n445 = case shown="True" "Once" {
            frame False {
            }
            frame True {
              n446 = local write "Trig"(FALSE ("Start")) -> ()
            }
          }
        }
        frame 6 {
          # "START"
          n447 = for {
            N: 5 -> [_]
            tunnel: w1059 -> [w1068]
            tunnel: w1058 -> [w1067]
            tunnel: [FALSE] -> w1057
            n448 = case shown="1" w1067 {
              tunnel: TRUE -> [w1069 w1070]
              frame 0, Default {
                "Start" <- w1069
              }
              frame 1 {
                "Start 2" <- w1070
              }
            }
            n449 = Wait Until Next ms Multiple(millisecond multiple=w1068) -> ()  [unwired: 1 out]
          }
          n450 = call <vilib>:"ULx Start Task.vi"("task in"=w1062, "error in"=w1061) -> ("task out"=w1054:refnum<k24>, "error out"=w1053:errorcluster)  [unwired: 12 in]
          n451 = local write "Start"(w1057) -> ()
          n452 = local write "Start 2"(w1057) -> ()
          n453 = case shown="True" "Once" {
            frame False {
            }
            frame True {
              n454 = local write "Start"(FALSE ("Start")) -> ()
            }
          }
          n455 = case shown="True" "Once" {
            frame False {
            }
            frame True {
              n456 = local write "Start"(FALSE ("Start")) -> ()
            }
          }
        }
        frame 7 {
          # "WRITE"
          n457 = call "Complicated Function Generator.vi"("frequency"="freq", "signal type"="sig type", "offset"="offset", "amplitude"="ampl", "samples"="samps", "bufsize"="samps", "Chans"="Chans") -> ("Wave out"=w1081:waveform(dbl), "WfmArray"=w1079:waveform(dbl)[], "DblArray"=w1080:dbl[][], "DBL Out"=w1076:dbl[])  [unwired: 3 in, 2 out]
          n458 = property on="samples" class="DigNum (strict)"("Maximum"="samps") -> ()  [unwired: 2 in, 2 out]
          n459 = case shown="False" "Mod Array" {
            tunnel: "Chans" -> [_ w1098]
            tunnel: w1076 -> [w1092 w1097]
            tunnel: [w1092 w1093] -> w1075
            frame False {
            }
            frame True {
              n460 = call "Complicated Function Generator.vi"("frequency"="freq", "signal type"="signal type", "amplitude"="atude", "samples"="samples", "bufsize"="samples", "Chans"=w1098) -> ("DBL Out"=w1100:dbl[])  [unwired: 4 in, 5 out]
              n461 = Replace Array Subset(array=w1097, new element=w1100, index="index") -> (w1093:dbl[])
            }
          }
          n462 = stacked-sequence {
            tunnel: w1090 -> [_ w1123]
            tunnel: w1089 -> [_ w1115]
            tunnel: w1088 -> [_ w1114]
            tunnel: [_ w1119] -> w1087
            tunnel: [_ w1118] -> w1086
            tunnel: w1085 -> [w1102 _]
            tunnel: [_ FALSE] -> w1084
            tunnel: w1075 -> [_ w1109]
            tunnel: w1081 -> [_ w1113]
            tunnel: w1080 -> [_ w1112]
            tunnel: w1079 -> [_ w1111]
            tunnel: "samps" -> [_ w1110]
            tunnel: "sig type" -> [_ w1108]
            tunnel: "Chans" -> [_ w1106]
            frame #0 {
              n463 = for {
                N: 5 -> [_]
                tunnel: w1102 -> [w1105]
                n464 = Wait Until Next ms Multiple(millisecond multiple=w1105) -> ()  [unwired: 1 out]
                "Write" <- TRUE ("Write")
              }
            }
            frame #1 {
              n465 = case shown="\"Composite\"" "TaskType 2" {
                tunnel: w1114 -> [w1144 w1225 w1416 w1505]
                tunnel: w1115 -> [w1143 w1224 w1417 w1506]
                tunnel: w1123 -> [w1141 w1223 w1415 w1504]
                tunnel: [w1139 w1220 w1412 w1503] -> w1118
                tunnel: [w1140 w1221 w1413 w1502] -> w1119
                tunnel: "AutoStart" -> [w1138 w1219 w1411 w1501]
                tunnel: [w1137 w1217 w1409 w1499] -> w1121
                tunnel: "TO" -> [w1136 w1218 w1410 w1500]
                tunnel: w1109 -> [w1135 w1216 _ w1495]
                tunnel: w1113 -> [w1134 _ _ _]
                tunnel: w1112 -> [w1133 _ _ w1498]
                tunnel: w1111 -> [w1132 _ _ w1497]
                tunnel: w1110 -> [_ w1215 _ w1496]
                tunnel: w1106 -> [_ _ _ w1493]
                frame "Analog", Default {
                  n466 = case shown="\"nCnS2D\"" "AWrite" {
                    tunnel: [w1151 w1160 w1166 w1173 w1181 w1189 w1197 w1207 w1209 w1212 w1214] -> w1139
                    tunnel: [w1152 w1159 w1165 w1174 w1182 w1190 w1198 w1208 w1210 w1211 w1213] -> w1140
                    tunnel: w1143 -> [w1150 w1158 w1168 w1175 w1184 w1192 w1200 w1206 w1210 w1211 w1213]
                    tunnel: w1144 -> [w1149 w1157 w1167 w1176 w1183 w1191 w1199 w1205 w1209 w1212 w1214]
                    tunnel: w1141 -> [_ _ _ _ _ _ _ _ _ _ _]
                    tunnel: w1138 -> [w1147 w1155 w1164 w1172 w1178 w1186 w1196 w1204 _ _ _]
                    tunnel: [w1145 w1153 w1163 w1171 w1177 w1185 w1195 w1203 _ _ _] -> w1137
                    tunnel: w1136 -> [w1146 w1154 w1162 w1170 w1179 w1187 w1194 w1202 _ _ _]
                    tunnel: w1135 -> [_ _ w1161 _ _ _ _ _ _ _ _]
                    tunnel: w1134 -> [_ _ _ w1169 _ _ _ _ _ _ _]
                    tunnel: w1133 -> [_ _ _ _ _ _ w1193 _ _ _ _]
                    tunnel: w1132 -> [_ _ _ _ _ _ _ w1201 _ _ _]
                    frame "sCsSDbl", Default {
                      n467 = call-poly <vilib>:"ULx Write.vi"("task in"=w1150, "auto start"=w1147, "data"="data 2", "timeout"=w1146, "error in"=w1149) -> ("task out"=w1152:refnum<k24>, "number of samples written per channel"=w1145:u32, "error out"=w1151:errorcluster)  [unwired: 8 in]
                    }
                    frame "sCsSWfm" {
                      n468 = call-poly <vilib>:"ULx Write.vi"("task in"=w1158, "auto start"=w1155, "data"="data", "timeout"=w1154, "error in"=w1157) -> ("task out"=w1159:refnum<k24>, "number of samples written per channel"=w1153:u32, "error out"=w1160:errorcluster)  [unwired: 8 in]
                    }
                    frame "sCnS1D" {
                      n469 = local write "Single Channel\n  1-D Array"(w1161) -> ()
                      n470 = call-poly <vilib>:"ULx Write.vi"("task in"=w1168, "auto start"=w1164, "data"=w1161, "timeout"=w1162, "error in"=w1167) -> ("task out"=w1165:refnum<k24>, "number of samples written per channel"=w1163:u32, "error out"=w1166:errorcluster)  [unwired: 8 in]
                      "data 3" <- w1161
                    }
                    frame "sCnSWfm" {
                      n471 = call-poly <vilib>:"ULx Write.vi"("task in"=w1175, "auto start"=w1172, "data"=w1169, "timeout"=w1170, "error in"=w1176) -> ("task out"=w1174:refnum<k24>, "number of samples written per channel"=w1171:u32, "error out"=w1173:errorcluster)  [unwired: 8 in]
                      "data 4" <- w1169
                    }
                    frame "nCsSDbl" {
                      n472 = call-poly <vilib>:"ULx Write.vi"("task in"=w1184, "auto start"=w1178, "data"="data 5", "timeout"=w1179, "error in"=w1183) -> ("task out"=w1182:refnum<k24>, "number of samples written per channel"=w1177:u32, "error out"=w1181:errorcluster)  [unwired: 8 in]
                    }
                    frame "nCsSWfm" {
                      n473 = call-poly <vilib>:"ULx Write.vi"("task in"=w1192, "auto start"=w1186, "data"="data 6", "timeout"=w1187, "error in"=w1191) -> ("task out"=w1190:refnum<k24>, "number of samples written per channel"=w1185:u32, "error out"=w1189:errorcluster)  [unwired: 8 in]
                    }
                    frame "nCnS2D" {
                      n474 = local write "Multi-channel\n  2-D Array"(w1193) -> ()
                      n475 = call-poly <vilib>:"ULx Write.vi"("task in"=w1200, "auto start"=w1196, "data"=w1193, "timeout"=w1194, "error in"=w1199) -> ("task out"=w1198:refnum<k24>, "number of samples written per channel"=w1195:u32, "error out"=w1197:errorcluster)  [unwired: 8 in]
                      "data 7" <- w1193
                    }
                    frame "nCnS1DWfm" {
                      n476 = call-poly <vilib>:"ULx Write.vi"("task in"=w1206, "auto start"=w1204, "data"=w1201, "timeout"=w1202, "error in"=w1205) -> ("task out"=w1208:refnum<k24>, "number of samples written per channel"=w1203:u32, "error out"=w1207:errorcluster)  [unwired: 8 in]
                      "data 8" <- w1201
                    }
                    frame "2DI16" {
                    }
                    frame "2DI32" {
                    }
                    frame "2DU16" {
                    }
                  }
                }
                frame "Digital" {
                  n477 = case shown="\"Single Channel\"" "nOrsDChan" {
                    tunnel: w1225 -> [w1234 w1326]
                    tunnel: w1224 -> [w1233 w1327]
                    tunnel: w1223 -> [w1232 w1325]
                    tunnel: [w1230 w1324] -> w1221
                    tunnel: [w1229 w1323] -> w1220
                    tunnel: w1219 -> [w1227 w1322]
                    tunnel: w1218 -> [w1228 w1321]
                    tunnel: [w1226 w1320] -> w1217
                    tunnel: w1216 -> [_ w1318]
                    tunnel: w1215 -> [_ w1317]
                    frame "Multi-Channel", Default {
                      n478 = case shown="\"nCsSBool\", Default" "nDWrite" {
                        tunnel: [w1241 w1250 w1257 w1266 w1273 w1281 w1289 w1298 w1305 w1314] -> w1229
                        tunnel: [w1242 w1249 w1258 w1265 w1274 w1282 w1290 w1297 w1306 w1313] -> w1230
                        tunnel: w1232 -> [_ _ _ _ _ _ _ _ _ _]
                        tunnel: w1233 -> [w1240 w1248 w1255 w1263 w1271 w1279 w1287 w1295 w1304 w1312]
                        tunnel: w1234 -> [w1239 w1247 w1256 w1264 w1272 w1280 w1288 w1296 w1303 w1311]
                        tunnel: w1228 -> [w1237 w1245 w1253 w1261 w1269 w1277 w1285 w1293 w1301 w1309]
                        tunnel: w1227 -> [w1236 w1244 w1252 w1260 w1268 w1275 w1284 w1292 w1300 w1308]
                        tunnel: [w1235 w1243 w1251 w1259 w1267 w1276 w1283 w1291 w1299 w1307] -> w1226
                        frame "nCsSBool", Default {
                          n479 = call-poly <vilib>:"ULx Write.vi"("task in"=w1240, "auto start"=w1236, "data"="data 12", "timeout"=w1237, "error in"=w1239) -> ("task out"=w1242:refnum<k24>, "number of samples written per channel"=w1235:u32, "error out"=w1241:errorcluster)  [unwired: 8 in]
                        }
                        frame "nCsS2D" {
                          n480 = call-poly <vilib>:"ULx Write.vi"("task in"=w1248, "auto start"=w1244, "data"="data 13", "timeout"=w1245, "error in"=w1247) -> ("task out"=w1249:refnum<k24>, "number of samples written per channel"=w1243:u32, "error out"=w1250:errorcluster)  [unwired: 8 in]
                        }
                        frame "nCsSU8" {
                          n481 = call-poly <vilib>:"ULx Write.vi"("task in"=w1255, "auto start"=w1252, "data"="data 14", "timeout"=w1253, "error in"=w1256) -> ("task out"=w1258:refnum<k24>, "number of samples written per channel"=w1251:u32, "error out"=w1257:errorcluster)  [unwired: 8 in]
                        }
                        frame "nCsSU16" {
                          n482 = call-poly <vilib>:"ULx Write.vi"("task in"=w1263, "auto start"=w1260, "data"="data 15", "timeout"=w1261, "error in"=w1264) -> ("task out"=w1265:refnum<k24>, "number of samples written per channel"=w1259:u32, "error out"=w1266:errorcluster)  [unwired: 8 in]
                        }
                        frame "nCsSU32" {
                          n483 = call-poly <vilib>:"ULx Write.vi"("task in"=w1271, "auto start"=w1268, "data"="data 16", "timeout"=w1269, "error in"=w1272) -> ("task out"=w1274:refnum<k24>, "number of samples written per channel"=w1267:u32, "error out"=w1273:errorcluster)  [unwired: 8 in]
                        }
                        frame "nCsSWv" {
                          n484 = call-poly <vilib>:"ULx Write.vi"("task in"=w1279, "auto start"=w1275, "data"="data 17", "timeout"=w1277, "error in"=w1280) -> ("task out"=w1282:refnum<k24>, "number of samples written per channel"=w1276:u32, "error out"=w1281:errorcluster)  [unwired: 8 in]
                        }
                        frame "nCnSU8" {
                          n485 = call-poly <vilib>:"ULx Write.vi"("task in"=w1287, "auto start"=w1284, "data"="data 18", "timeout"=w1285, "error in"=w1288) -> ("task out"=w1290:refnum<k24>, "number of samples written per channel"=w1283:u32, "error out"=w1289:errorcluster)  [unwired: 8 in]
                        }
                        frame "nCnSU16" {
                          n486 = call-poly <vilib>:"ULx Write.vi"("task in"=w1295, "auto start"=w1292, "data"="data 19", "timeout"=w1293, "error in"=w1296) -> ("task out"=w1297:refnum<k24>, "number of samples written per channel"=w1291:u32, "error out"=w1298:errorcluster)  [unwired: 8 in]
                        }
                        frame "nCnSU32" {
                          n487 = call-poly <vilib>:"ULx Write.vi"("task in"=w1304, "auto start"=w1300, "data"="data 20", "timeout"=w1301, "error in"=w1303) -> ("task out"=w1306:refnum<k24>, "number of samples written per channel"=w1299:u32, "error out"=w1305:errorcluster)  [unwired: 8 in]
                        }
                        frame "nCnSWv" {
                          n488 = call-poly <vilib>:"ULx Write.vi"("task in"=w1312, "auto start"=w1308, "data"="data 21", "timeout"=w1309, "error in"=w1311) -> ("task out"=w1313:refnum<k24>, "number of samples written per channel"=w1307:u32, "error out"=w1314:errorcluster)  [unwired: 8 in]
                        }
                      }
                    }
                    frame "Single Channel" {
                      n489 = call "AtoDSigConvert.vi"("Samples"=w1317, "Array Input"=w1318) -> ("sCnSu32"=w1315:u32[], "sCnSu16"=w1316:u16[], "sCnSu8"=w1319:u8[])
                      n490 = case shown="\"sCnSWv\"" "sDWrite" {
                        tunnel: [w1335 w1344 w1351 w1360 w1367 w1375 w1383 w1392 w1399 w1408] -> w1323
                        tunnel: [w1336 w1343 w1352 w1359 w1368 w1376 w1384 w1391 w1400 w1407] -> w1324
                        tunnel: w1325 -> [_ _ _ _ _ _ _ _ _ _]
                        tunnel: w1327 -> [w1334 w1342 w1349 w1357 w1365 w1373 w1381 w1389 w1398 w1406]
                        tunnel: w1326 -> [w1333 w1341 w1350 w1358 w1366 w1374 w1382 w1390 w1397 w1405]
                        tunnel: w1322 -> [w1330 w1339 w1346 w1354 w1362 w1371 w1379 w1387 w1395 w1402]
                        tunnel: w1321 -> [w1331 w1338 w1347 w1355 w1363 w1369 w1380 w1388 w1396 w1403]
                        tunnel: [w1329 w1337 w1345 w1353 w1361 w1370 w1378 w1386 w1394 w1401] -> w1320
                        tunnel: w1319 -> [_ _ _ _ _ _ w1377 _ _ _]
                        tunnel: w1316 -> [_ _ _ _ _ _ _ w1385 _ _]
                        tunnel: w1315 -> [_ _ _ _ _ _ _ _ w1393 _]
                        frame "sCsSBool", Default {
                          n491 = call-poly <vilib>:"ULx Write.vi"("task in"=w1334, "auto start"=w1330, "data"="data 22", "timeout"=w1331, "error in"=w1333) -> ("task out"=w1336:refnum<k24>, "number of samples written per channel"=w1329:u32, "error out"=w1335:errorcluster)  [unwired: 8 in]
                        }
                        frame "sCsS1D" {
                          n492 = call-poly <vilib>:"ULx Write.vi"("task in"=w1342, "auto start"=w1339, "data"="data 23", "timeout"=w1338, "error in"=w1341) -> ("task out"=w1343:refnum<k24>, "number of samples written per channel"=w1337:u32, "error out"=w1344:errorcluster)  [unwired: 8 in]
                        }
                        frame "sCsSU8" {
                          n493 = call-poly <vilib>:"ULx Write.vi"("task in"=w1349, "auto start"=w1346, "data"="data 24", "timeout"=w1347, "error in"=w1350) -> ("task out"=w1352:refnum<k24>, "number of samples written per channel"=w1345:u32, "error out"=w1351:errorcluster)  [unwired: 8 in]
                        }
                        frame "sCsSU16" {
                          n494 = call-poly <vilib>:"ULx Write.vi"("task in"=w1357, "auto start"=w1354, "data"="data 25", "timeout"=w1355, "error in"=w1358) -> ("task out"=w1359:refnum<k24>, "number of samples written per channel"=w1353:u32, "error out"=w1360:errorcluster)  [unwired: 8 in]
                        }
                        frame "sCsSU32" {
                          n495 = call-poly <vilib>:"ULx Write.vi"("task in"=w1365, "auto start"=w1362, "data"="data 26", "timeout"=w1363, "error in"=w1366) -> ("task out"=w1368:refnum<k24>, "number of samples written per channel"=w1361:u32, "error out"=w1367:errorcluster)  [unwired: 8 in]
                        }
                        frame "sCsSWv" {
                          n496 = call-poly <vilib>:"ULx Write.vi"("task in"=w1373, "auto start"=w1371, "data"="data 27", "timeout"=w1369, "error in"=w1374) -> ("task out"=w1376:refnum<k24>, "number of samples written per channel"=w1370:u32, "error out"=w1375:errorcluster)  [unwired: 8 in]
                        }
                        frame "sCnSU8" {
                          n497 = local write "Single Channel\n  Unsigned 8-bit"(w1377) -> ()
                          n498 = call-poly <vilib>:"ULx Write.vi"("task in"=w1381, "auto start"=w1379, "data"=w1377, "timeout"=w1380, "error in"=w1382) -> ("task out"=w1384:refnum<k24>, "number of samples written per channel"=w1378:u32, "error out"=w1383:errorcluster)  [unwired: 8 in]
                          "data 28" <- w1377
                        }
                        frame "sCnSU16" {
                          n499 = local write "Single Channel\n  Unsigned 16-bit"(w1385) -> ()
                          n500 = call-poly <vilib>:"ULx Write.vi"("task in"=w1389, "auto start"=w1387, "data"=w1385, "timeout"=w1388, "error in"=w1390) -> ("task out"=w1391:refnum<k24>, "number of samples written per channel"=w1386:u32, "error out"=w1392:errorcluster)  [unwired: 8 in]
                          "data 29" <- w1385
                        }
                        frame "sCnSU32" {
                          n501 = local write "Single Channel\n  Unsigned 32-bit"(w1393) -> ()
                          n502 = call-poly <vilib>:"ULx Write.vi"("task in"=w1398, "auto start"=w1395, "data"=w1393, "timeout"=w1396, "error in"=w1397) -> ("task out"=w1400:refnum<k24>, "number of samples written per channel"=w1394:u32, "error out"=w1399:errorcluster)  [unwired: 8 in]
                          "data 30" <- w1393
                        }
                        frame "sCnSWv" {
                          n503 = call-poly <vilib>:"ULx Write.vi"("task in"=w1406, "auto start"=w1402, "data"="data 31", "timeout"=w1403, "error in"=w1405) -> ("task out"=w1407:refnum<k24>, "number of samples written per channel"=w1401:u32, "error out"=w1408:errorcluster)  [unwired: 8 in]
                        }
                      }
                    }
                  }
                }
                frame "Counter" {
                  n504 = case shown="\"Multi-Channel\", Default" "nOrsCChan" {
                    tunnel: w1417 -> [w1425 w1459]
                    tunnel: w1416 -> [w1424 w1458]
                    tunnel: w1415 -> [w1426 w1457]
                    tunnel: [w1422 w1455] -> w1413
                    tunnel: [w1421 w1454] -> w1412
                    tunnel: w1411 -> [w1420 w1453]
                    tunnel: w1410 -> [w1418 w1452]
                    tunnel: [w1419 w1451] -> w1409
                    frame "Multi-Channel", Default {
                      n505 = case shown="\"Frequency\", Default" "nCtrWrite" {
                        tunnel: w1425 -> [w1434 w1442 w1450]
                        tunnel: w1424 -> [w1433 w1441 w1449]
                        tunnel: w1426 -> [_ _ _]
                        tunnel: [w1431 w1439 w1447] -> w1422
                        tunnel: [w1430 w1438 w1446] -> w1421
                        tunnel: w1420 -> [w1429 w1437 w1445]
                        tunnel: [w1428 w1435 w1443] -> w1419
                        tunnel: w1418 -> [w1427 w1436 w1444]
                        frame "Frequency", Default {
                          n506 = call-poly <vilib>:"ULx Write.vi"("task in"=w1434, "auto start"=w1429, "data"="data 32", "timeout"=w1427, "error in"=w1433) -> ("task out"=w1431:refnum<k24>, "number of samples written per channel"=w1428:u32, "error out"=w1430:errorcluster)  [unwired: 8 in]
                        }
                        frame "Time" {
                          n507 = call-poly <vilib>:"ULx Write.vi"("task in"=w1442, "auto start"=w1437, "data"="data 34", "timeout"=w1436, "error in"=w1441) -> ("task out"=w1439:refnum<k24>, "number of samples written per channel"=w1435:u32, "error out"=w1438:errorcluster)  [unwired: 8 in]
                        }
                        frame "Ticks" {
                          n508 = call-poly <vilib>:"ULx Write.vi"("task in"=w1450, "auto start"=w1445, "data"="data 33", "timeout"=w1444, "error in"=w1449) -> ("task out"=w1447:refnum<k24>, "number of samples written per channel"=w1443:u32, "error out"=w1446:errorcluster)  [unwired: 8 in]
                        }
                      }
                    }
                    frame "Single Channel" {
                      n509 = case shown="\"Frequency\", Default" "sCtrWrite" {
                        tunnel: w1459 -> [w1468 w1477 w1486]
                        tunnel: w1458 -> [w1467 w1476 w1485]
                        tunnel: w1457 -> [_ _ _]
                        tunnel: [w1464 w1473 w1482] -> w1455
                        tunnel: [w1463 w1472 w1481] -> w1454
                        tunnel: w1453 -> [w1462 w1471 w1480]
                        tunnel: w1452 -> [w1461 w1470 w1479]
                        tunnel: [w1460 w1469 w1478] -> w1451
                        frame "Frequency", Default {
                          n510 = call-poly <vilib>:"ULx Write.vi"("task in"=w1468, "auto start"=w1462, "frequency"="frequency", "duty cycle"="duty cycle", "timeout"=w1461, "error in"=w1467) -> ("task out"=w1464:refnum<k24>, "number of samples written per channel"=w1460:u32, "error out"=w1463:errorcluster)  [unwired: 7 in]
                        }
                        frame "Time" {
                          n511 = call-poly <vilib>:"ULx Write.vi"("task in"=w1477, "auto start"=w1471, "high time"="high time", "low time"="low time", "timeout"=w1470, "error in"=w1476) -> ("task out"=w1473:refnum<k24>, "number of samples written per channel"=w1469:u32, "error out"=w1472:errorcluster)  [unwired: 7 in]
                        }
                        frame "Ticks" {
                          n512 = call-poly <vilib>:"ULx Write.vi"("task in"=w1486, "auto start"=w1480, "high ticks"="high ticks", "low ticks"="low ticks", "timeout"=w1479, "error in"=w1485) -> ("task out"=w1482:refnum<k24>, "number of samples written per channel"=w1478:u32, "error out"=w1481:errorcluster)  [unwired: 7 in]
                        }
                      }
                    }
                  }
                }
                frame "Composite" {
                  n513 = local read "ULx"() -> (w1491:refnum<k21>)
                  n514 = local read "ULx"() -> (w1487:refnum<k21>)
                  n515 = call "MultiChanAtoD.vi"("Array Input"=w1495, "Chans"=w1493, "Samples"=w1496) -> ("u32Array"=w1494:u32[][])  [unwired: 1 in, 5 out]
                  n516 = Equal?(x=w1487, y="") -> (x = y?=w1488:bool)
                  n517 = Equal?(x=w1491, y="") -> (x = y?=w1490:bool)
                  n518 = case shown="\"1D Waveform\"" "CompWrite" {
                    tunnel: w1506 -> [w1520 w1531]
                    tunnel: w1505 -> [w1519 w1530]
                    tunnel: w1504 -> [_ _]
                    tunnel: [w1518 w1528] -> w1503
                    tunnel: [w1517 w1529] -> w1502
                    tunnel: w1501 -> [w1516 w1527]
                    tunnel: w1500 -> [w1514 w1526]
                    tunnel: [w1515 w1525] -> w1499
                    tunnel: w1498 -> [w1513 _]
                    tunnel: w1497 -> [_ w1524]
                    tunnel: w1494 -> [w1511 _]
                    tunnel: w1490 -> [w1512 _]
                    tunnel: w1488 -> [w1509 _]
                    frame "2D", Default {
                      n519 = case shown="True" w1509 {
                        tunnel: w1511 -> [w1521 _]
                        tunnel: [w1521 _] -> w1510
                        frame False {
                        }
                        frame True {
                        }
                      }
                      "u32Array" <- w1510
                      "u32Plot" <- w1510
                      n520 = case shown="False" w1512 {
                        tunnel: w1513 -> [w1522 _]
                        tunnel: [w1522 _] -> w1508
                        frame False {
                        }
                        frame True {
                        }
                      }
                      "DblArray 2" <- w1508
                      n521 = local write "Multi-channel\n  2-D Array"(w1508) -> ()
                      n522 = call-poly <vilib>:"ULx Write.vi"("task in"=w1520, "auto start"=w1516, "analog data"=w1508, "digital data"=w1510, "timeout"=w1514, "error in"=w1519) -> ("task out"=w1517:refnum<k24>, "number of samples written per channel"=w1515:u32, "error out"=w1518:errorcluster)  [unwired: 7 in]
                    }
                    frame "1D Waveform" {
                      n523 = call-poly <vilib>:"ULx Write.vi"("task in"=w1531, "auto start"=w1527, "analog data"=w1524, "digital data"="digital data 2", "timeout"=w1526, "error in"=w1530) -> ("task out"=w1529:refnum<k24>, "number of samples written per channel"=w1525:u32, "error out"=w1528:errorcluster)  [unwired: 7 in]
                      "WfmArray" <- w1524
                    }
                  }
                }
              }
              "Written" <- w1121
              n524 = case shown="True" "Change" {
                tunnel: w1108 -> [_ w1124]
                frame False {
                }
                frame True {
                  n525 = Add(x=w1124, y=1) -> (x+y=w1129:i32)
                  n526 = Greater?(x=w1129, y=3 ("x")) -> (0:w1126:bool)
                  n527 = case shown="True" w1126 {
                    tunnel: [w1130 0] -> w1127
                    tunnel: w1129 -> [w1130 _]
                    frame False {
                    }
                    frame True {
                    }
                  }
                  n528 = property on="sig type" class="Enum (strict)"("Value"=w1127) -> ()  [unwired: 2 in, 2 out]
                }
              }
            }
          }
          n529 = case shown="True" "Once" {
            frame False {
            }
            frame True {
              n530 = local write "Write"(FALSE ("Write")) -> ()
            }
          }
          n531 = local write "Write"(w1084) -> ()
        }
        frame 8 {
          # "STATUS"
          n532 = stacked-sequence {
            seq-local: [w1542 _] -> [_ w1550]
            seq-local: [w1541 _] -> [_ w1549]
            tunnel: w1538 -> [w1542 _]
            tunnel: w1537 -> [w1541 _]
            tunnel: w1534 -> [_ w1545]
            tunnel: w1533 -> [w1539 _]
            tunnel: [_ w1548] -> w1536
            tunnel: [_ w1547] -> w1535
            tunnel: [_ FALSE ("Submit")] -> w1532
            frame #0 {
              n533 = for {
                N: 5 -> [_]
                tunnel: w1539 -> [w1543]
                n534 = Wait Until Next ms Multiple(millisecond multiple=w1543) -> ()  [unwired: 1 out]
                "Status" <- TRUE
              }
            }
            frame #1 {
              n535 = while {
                tunnel: w1550 -> [w1560]
                tunnel: w1549 -> [w1559]
                tunnel: [w1558] -> w1548
                tunnel: [w1555] -> w1547
                tunnel: w1545 -> [_]
                i -> [w1557]
                stop <- w1562 stop-if-true
                n536 = Wait Until Next ms Multiple(millisecond multiple=u32 300) -> ()  [unwired: 1 out]
                n537 = call <vilib>:"ULx Is Task Done.vi"("task in"=w1560, "error in"=w1559) -> ("task out"=w1558:refnum<k24>, "task done?"=w1552:bool, "error out"=w1555:errorcluster)  [unwired: 11 in]
                "task \ndone?" <- w1552
                n538 = call "TextError.vi"("error in"=w1555) -> ("message"=w1554:string)  [unwired: 1 in]
                n539 = local read "Status\nLoop"() -> (w1553:bool)
                n540 = local write "message 2"(w1554) -> ()
                n541 = Not(x=w1553) -> (.not. x?=w1551:bool)
                n542 = local read "Submit"() -> (w1563:bool)
                n543 = local read "stop"() -> (w1561:bool)
                n544 = Compound Arithmetic op=OR(w1552, w1551, w1561, w1563) -> (w1562:bool)
                "# of Loops" <- w1557
              }
            }
          }
          n545 = local write "Status"(w1532) -> ()
          n546 = local write "Submit"(w1532) -> ()
        }
        frame 9 {
          # "STOP"
          n547 = for {
            N: 5 -> [_]
            tunnel: w1576 -> [w1594]
            tunnel: [FALSE] -> w1575
            n548 = Wait Until Next ms Multiple(millisecond multiple=w1594) -> ()  [unwired: 1 out]
            "Stop" <- TRUE
          }
          n549 = flat-sequence {
            tunnel: w1573 -> [w1581]
            tunnel: [w1581] -> w1572
            tunnel: w1569 -> [w1580]
            tunnel: [w1580] -> w1568
            tunnel: [w1579] -> w1564
            tunnel: w1572 -> [w1586]
            tunnel: [w1585] -> w1571
            tunnel: w1568 -> [w1584]
            tunnel: [w1583] -> w1567
            tunnel: [w1582] -> w1565
            tunnel: w1564 -> [w1582]
            tunnel: w1571 -> [w1591]
            tunnel: [w1591] -> w1570
            tunnel: w1567 -> [w1590]
            tunnel: [w1590] -> w1566
            tunnel: w1565 -> [w1588]
            frame #0 {
              n550 = Tick Count (ms)() -> (millisecond timer value=w1579:u32)
            }
            frame #1 {
              n551 = call <vilib>:"ULx Stop Task.vi"("error in"=w1584, "task in"=w1586) -> ("error out"=w1583:errorcluster, "task out"=w1585:refnum<k24>)  [unwired: 8 in]
            }
            frame #2 {
              n552 = Tick Count (ms)() -> (millisecond timer value=w1589:u32)
              n553 = Subtract(x=w1589, y=w1588) -> (x-y=→"Stop Time":u32)
            }
          }
          n554 = local write "Stop"(w1575) -> ()
          n555 = case shown="True" "Once" {
            frame False {
            }
            frame True {
              n556 = local write "Stop"(FALSE ("Stop")) -> ()
            }
          }
          "Task Stopped" <- TRUE
        }
        frame 10 {
          # "CLEAR"
          n557 = for {
            N: 5 -> [_]
            tunnel: w1597 -> [w1604]
            tunnel: [FALSE] -> w1596
            n558 = Wait Until Next ms Multiple(millisecond multiple=w1604) -> ()  [unwired: 1 out]
            "Clear" <- TRUE
          }
          n559 = local write "Clear"(w1596) -> ()
          n560 = call <vilib>:"ULx Clear Task.vi"("task in"=w1602, "error in"=w1601) -> ("error out"=w1599:errorcluster)  [unwired: 13 in]
          "Task Cleared" <- TRUE
        }
        frame 11 {
          # "READ"
          n561 = stacked-sequence {
            tunnel: w1613 -> [_ w1625]
            tunnel: w1612 -> [_ w1624]
            tunnel: w1611 -> [_ w1623]
            tunnel: [_ w1622] -> w1610
            tunnel: [_ w1621] -> w1609
            tunnel: w1608 -> [w1615 _]
            tunnel: [_ FALSE] -> w1607
            frame #0 {
              n562 = for {
                N: 5 -> [_]
                tunnel: w1615 -> [w1618]
                n563 = Wait Until Next ms Multiple(millisecond multiple=w1618) -> ()  [unwired: 1 out]
                "Read" <- TRUE ("Write")
              }
            }
            frame #1 {
              n564 = case shown="\"Counter\"" "ReadType" {
                tunnel: w1625 -> [w1632 w1701 w1849 w1910]
                tunnel: w1624 -> [w1631 w1700 w1850 w1911]
                tunnel: w1623 -> [w1630 w1697 w1846 w1907]
                tunnel: [w1629 w1698 w1848 w1909] -> w1622
                tunnel: [w1628 w1699 w1847 w1908] -> w1621
                tunnel: "timeout" -> [w1627 w1696 w1845 w1905]
                frame "Analog", Default {
                  n565 = case shown="\"nCnS1DWfm\"" "ARead" {
                    tunnel: [w1638 w1645 w1651 w1659 w1665 w1671 w1679 w1687 w1689 w1691 w1693 w1695] -> w1628
                    tunnel: [w1639 w1644 w1652 w1658 w1666 w1672 w1680 w1686 w1688 w1690 w1692 w1694] -> w1629
                    tunnel: w1632 -> [w1637 w1643 w1649 w1656 w1663 w1669 w1677 w1684 w1688 w1690 w1692 w1694]
                    tunnel: w1631 -> [w1636 w1642 w1650 w1657 w1664 w1670 w1678 w1685 w1689 w1691 w1693 w1695]
                    tunnel: w1630 -> [_ _ _ _ _ _ _ _ _ _ _ _]
                    tunnel: w1627 -> [w1634 w1640 w1648 w1654 w1662 w1667 w1676 w1683 _ _ _ _]
                    frame "sCsSDbl", Default {
                      n566 = call-poly <vilib>:"ULx Read.vi"("task in"=w1637, "timeout"=w1634, "error in"=w1636) -> ("task out"=w1639:refnum<k24>, "data"=→"data 35":dbl, "error out"=w1638:errorcluster)  [unwired: 10 in]
                    }
                    frame "sCsSWfm" {
                      n567 = call-poly <vilib>:"ULx Read.vi"("task in"=w1643, "timeout"=w1640, "error in"=w1642) -> ("task out"=w1644:refnum<k24>, "data"=→"data 36":waveform(dbl), "error out"=w1645:errorcluster)  [unwired: 10 in]
                    }
                    frame "sCnS1D" {
                      n568 = call-poly <vilib>:"ULx Read.vi"("task in"=w1649, "number of samples per channel"="samples per", "timeout"=w1648, "error in"=w1650) -> ("task out"=w1652:refnum<k24>, "data"=w1646:dbl[], "error out"=w1651:errorcluster)  [unwired: 9 in]
                      "data 37" <- w1646
                      n569 = local write "Single Channel\n  1-D Array"(w1646) -> ()
                    }
                    frame "sCnSWfm" {
                      n570 = call-poly <vilib>:"ULx Read.vi"("task in"=w1656, "number of samples per channel"="samples per", "timeout"=w1654, "error in"=w1657) -> ("task out"=w1658:refnum<k24>, "data"=→"data 38" →"Single Channel \n  Waveform":waveform(dbl), "error out"=w1659:errorcluster)  [unwired: 9 in]
                    }
                    frame "nCsSDbl" {
                      n571 = call-poly <vilib>:"ULx Read.vi"("task in"=w1663, "timeout"=w1662, "error in"=w1664) -> ("task out"=w1666:refnum<k24>, "data"=→"data 39":dbl[], "error out"=w1665:errorcluster)  [unwired: 10 in]
                      n572 = property on="data 39" class="Arr (strict)"("Visible"=TRUE) -> ()  [unwired: 2 in, 2 out]
                    }
                    frame "nCsSWfm" {
                      n573 = call-poly <vilib>:"ULx Read.vi"("task in"=w1669, "timeout"=w1667, "error in"=w1670) -> ("task out"=w1672:refnum<k24>, "data"=→"data 40":waveform(dbl)[], "error out"=w1671:errorcluster)  [unwired: 10 in]
                    }
                    frame "nCnS2D" {
                      n574 = call-poly <vilib>:"ULx Read.vi"("task in"=w1677, "number of samples per channel"="samples per", "timeout"=w1676, "error in"=w1678) -> ("task out"=w1680:refnum<k24>, "data"=w1674:dbl[][], "error out"=w1679:errorcluster)  [unwired: 9 in]
                      "data 41" <- w1674
                      n575 = local write "Multi-channel\n  2-D Array"(w1674) -> ()
                      n576 = property on="Multi-channel\n  2-D Array" class="WFGraph (strict)"("Visible"=TRUE) -> ()  [unwired: 2 in, 2 out]
                    }
                    frame "nCnS1DWfm" {
                      n577 = call-poly <vilib>:"ULx Read.vi"("task in"=w1684, "number of samples per channel"="samples per", "timeout"=w1683, "error in"=w1685) -> ("task out"=w1686:refnum<k24>, "data"=w1681:waveform(dbl)[], "error out"=w1687:errorcluster)  [unwired: 9 in]
                      "data 42" <- w1681
                      n578 = local write "Multi-channel\n  Waveform"(w1681) -> ()
                    }
                    frame "2DI16" {
                    }
                    frame "2DI32" {
                    }
                    frame "2DU16" {
                    }
                    frame "2DU32" {
                    }
                  }
                }
                frame "Digital" {
                  n579 = case shown="\"Multi-Channel\", Default" "nCOrsCDin" {
                    tunnel: w1701 -> [w1708 w1779]
                    tunnel: w1700 -> [w1707 w1778]
                    tunnel: [w1704 w1775] -> w1698
                    tunnel: [w1705 w1776] -> w1699
                    tunnel: w1697 -> [w1706 w1777]
                    tunnel: w1696 -> [w1703 w1774]
                    frame "Multi-Channel", Default {
                      n580 = case shown="\"nCnSWv\"" "nCDIn" {
                        tunnel: [w1714 w1721 w1726 w1733 w1738 w1744 w1751 w1759 w1765 w1772] -> w1705
                        tunnel: [w1715 w1720 w1727 w1732 w1739 w1745 w1752 w1758 w1766 w1771] -> w1704
                        tunnel: w1706 -> [_ _ _ _ _ _ _ _ _ _]
                        tunnel: w1708 -> [w1712 w1718 w1723 w1729 w1735 w1742 w1749 w1756 w1764 w1770]
                        tunnel: w1707 -> [w1711 w1717 w1724 w1730 w1736 w1743 w1750 w1757 w1763 w1769]
                        tunnel: w1703 -> [w1710 w1716 w1722 w1728 w1734 w1741 w1748 w1755 w1762 w1768]
                        frame "nCsSBool", Default {
                          n581 = call-poly <vilib>:"ULx Read.vi"("task in"=w1712, "timeout"=w1710, "error in"=w1711) -> ("task out"=w1715:refnum<k24>, "data"=→"data 47":bool[], "error out"=w1714:errorcluster)  [unwired: 10 in]
                        }
                        frame "nCsS2D" {
                          n582 = call-poly <vilib>:"ULx Read.vi"("task in"=w1718, "timeout"=w1716, "error in"=w1717) -> ("task out"=w1720:refnum<k24>, "data"=→"data 48":bool[][], "error out"=w1721:errorcluster)  [unwired: 10 in]
                        }
                        frame "nCsSU8" {
                          n583 = call-poly <vilib>:"ULx Read.vi"("task in"=w1723, "timeout"=w1722, "error in"=w1724) -> ("task out"=w1727:refnum<k24>, "data"=→"data 49":u8[], "error out"=w1726:errorcluster)  [unwired: 10 in]
                        }
                        frame "nCsSU16" {
                          n584 = call-poly <vilib>:"ULx Read.vi"("task in"=w1729, "timeout"=w1728, "error in"=w1730) -> ("task out"=w1732:refnum<k24>, "data"=→"data 50":u16[], "error out"=w1733:errorcluster)  [unwired: 10 in]
                        }
                        frame "nCsSU32" {
                          n585 = call-poly <vilib>:"ULx Read.vi"("task in"=w1735, "timeout"=w1734, "error in"=w1736) -> ("task out"=w1739:refnum<k24>, "data"=→"data 51":u32[], "error out"=w1738:errorcluster)  [unwired: 10 in]
                        }
                        frame "nCsSWv" {
                          n586 = call-poly <vilib>:"ULx Read.vi"("task in"=w1742, "timeout"=w1741, "error in"=w1743) -> ("task out"=w1745:refnum<k24>, "data"=→"data 52":digitalwaveform[], "error out"=w1744:errorcluster)  [unwired: 10 in]
                        }
                        frame "nCnSU8" {
                          n587 = call-poly <vilib>:"ULx Read.vi"("task in"=w1749, "number of samples per channel"="samples per", "timeout"=w1748, "error in"=w1750) -> ("task out"=w1752:refnum<k24>, "data"=w1746:u8[][], "error out"=w1751:errorcluster)  [unwired: 9 in]
                          "data 53" <- w1746
                          n588 = local write "Multi-channel\n  Unsigned 8-bit"(w1746) -> ()
                        }
                        frame "nCnSU16" {
                          n589 = call-poly <vilib>:"ULx Read.vi"("task in"=w1756, "number of samples per channel"="samples per", "timeout"=w1755, "error in"=w1757) -> ("task out"=w1758:refnum<k24>, "data"=w1753:u16[][], "error out"=w1759:errorcluster)  [unwired: 9 in]
                          "data 54" <- w1753
                          n590 = local write "Multi-channel\n  Unsigned 16-bit"(w1753) -> ()
                        }
                        frame "nCnSU32" {
                          n591 = call-poly <vilib>:"ULx Read.vi"("task in"=w1764, "number of samples per channel"="samples per", "timeout"=w1762, "error in"=w1763) -> ("task out"=w1766:refnum<k24>, "data"=w1760:u32[][], "error out"=w1765:errorcluster)  [unwired: 9 in]
                          "data 55" <- w1760
                          n592 = local write "Multi-channel\n  Unsigned 32-bit"(w1760) -> ()
                        }
                        frame "nCnSWv" {
                          n593 = call-poly <vilib>:"ULx Read.vi"("task in"=w1770, "number of samples per channel"="samples per", "timeout"=w1768, "error in"=w1769) -> ("task out"=w1771:refnum<k24>, "data"=→"data 56" →"Multi-\n  channel\n  Waveform":digitalwaveform[], "error out"=w1772:errorcluster)  [unwired: 9 in]
                        }
                      }
                    }
                    frame " Single Channel" {
                      n594 = case shown="\"sCnSWv\"" "sCDin" {
                        tunnel: [w1785 w1792 w1797 w1804 w1809 w1815 w1822 w1830 w1836 w1844] -> w1776
                        tunnel: [w1786 w1791 w1798 w1803 w1810 w1816 w1823 w1829 w1837 w1843] -> w1775
                        tunnel: w1777 -> [_ _ _ _ _ _ _ _ _ _]
                        tunnel: w1779 -> [w1784 w1790 w1795 w1801 w1807 w1813 w1819 w1827 w1834 w1841]
                        tunnel: w1778 -> [w1783 w1789 w1796 w1802 w1808 w1814 w1820 w1828 w1833 w1840]
                        tunnel: w1774 -> [w1781 w1787 w1793 w1799 w1806 w1811 w1818 w1826 w1832 w1838]
                        frame "sCsSBool", Default {
                          n595 = call-poly <vilib>:"ULx Read.vi"("task in"=w1784, "timeout"=w1781, "error in"=w1783) -> ("task out"=w1786:refnum<k24>, "data"=→"data 57":bool, "error out"=w1785:errorcluster)  [unwired: 10 in]
                        }
                        frame "sCsS1D" {
                          n596 = call-poly <vilib>:"ULx Read.vi"("task in"=w1790, "timeout"=w1787, "error in"=w1789) -> ("task out"=w1791:refnum<k24>, "data"=→"data 58":bool[], "error out"=w1792:errorcluster)  [unwired: 10 in]
                        }
                        frame "sCsSU8" {
                          n597 = call-poly <vilib>:"ULx Read.vi"("task in"=w1795, "timeout"=w1793, "error in"=w1796) -> ("task out"=w1798:refnum<k24>, "data"=→"data 59":u8, "error out"=w1797:errorcluster)  [unwired: 10 in]
                        }
                        frame "sCsSU16" {
                          n598 = call-poly <vilib>:"ULx Read.vi"("task in"=w1801, "timeout"=w1799, "error in"=w1802) -> ("task out"=w1803:refnum<k24>, "data"=→"data 60":u16, "error out"=w1804:errorcluster)  [unwired: 10 in]
                        }
                        frame "sCsSU32" {
                          n599 = call-poly <vilib>:"ULx Read.vi"("task in"=w1807, "timeout"=w1806, "error in"=w1808) -> ("task out"=w1810:refnum<k24>, "data"=→"data 43":u32, "error out"=w1809:errorcluster)  [unwired: 10 in]
                        }
                        frame "sCsSWv" {
                          n600 = call-poly <vilib>:"ULx Read.vi"("task in"=w1813, "timeout"=w1811, "error in"=w1814) -> ("task out"=w1816:refnum<k24>, "data"=→"data 62":digitalwaveform, "error out"=w1815:errorcluster)  [unwired: 10 in]
                        }
                        frame "sCnSU8" {
                          n601 = call-poly <vilib>:"ULx Read.vi"("task in"=w1819, "number of samples per channel"="samples per", "timeout"=w1818, "error in"=w1820) -> ("task out"=w1823:refnum<k24>, "data"=w1817:u8[], "error out"=w1822:errorcluster)  [unwired: 9 in]
                          "data 63" <- w1817
                          n602 = local write "Single Channel\n  Unsigned 8-bit"(w1817) -> ()
                        }
                        frame "sCnSU16" {
                          n603 = call-poly <vilib>:"ULx Read.vi"("task in"=w1827, "number of samples per channel"="samples per", "timeout"=w1826, "error in"=w1828) -> ("task out"=w1829:refnum<k24>, "data"=w1824:u16[], "error out"=w1830:errorcluster)  [unwired: 9 in]
                          "data 64" <- w1824
                          n604 = local write "Single Channel\n  Unsigned 16-bit"(w1824) -> ()
                        }
                        frame "sCnSU32" {
                          n605 = call-poly <vilib>:"ULx Read.vi"("task in"=w1834, "number of samples per channel"="samples per", "timeout"=w1832, "error in"=w1833) -> ("task out"=w1837:refnum<k24>, "data"=w1831:u32[], "error out"=w1836:errorcluster)  [unwired: 9 in]
                          "data 65" <- w1831
                          n606 = local write "Single Channel\n  Unsigned 32-bit"(w1831) -> ()
                        }
                        frame "sCnSWv" {
                          n607 = call-poly <vilib>:"ULx Read.vi"("task in"=w1841, "number of samples per channel"="samples per", "timeout"=w1838, "error in"=w1840) -> ("task out"=w1843:refnum<k24>, "data"=→"data 66" →"Single\n  Channel\n  Waveform":digitalwaveform, "error out"=w1844:errorcluster)  [unwired: 9 in]
                        }
                      }
                    }
                  }
                }
                frame "Counter" {
                  n608 = case shown="\"sCsSDbl\", Default" "CtrRead" {
                    tunnel: w1849 -> [w1857 w1863 w1870 w1877 w1883 w1889 w1896 w1903]
                    tunnel: w1850 -> [w1856 w1862 w1869 w1876 w1882 w1888 w1895 w1902]
                    tunnel: [w1855 w1861 w1868 w1875 w1881 w1887 w1894 w1901] -> w1847
                    tunnel: [w1854 w1860 w1867 w1874 w1880 w1886 w1893 w1900] -> w1848
                    tunnel: w1846 -> [_ _ _ _ _ _ _ _]
                    tunnel: w1845 -> [w1853 w1858 w1865 w1872 w1878 w1884 w1891 w1898]
                    frame "sCsSDbl", Default {
                      n609 = call-poly <vilib>:"ULx Read.vi"("task in"=w1857, "timeout"=w1853, "error in"=w1856) -> ("task out"=w1854:refnum<k24>, "data"=→"data 67" →"Gauge":dbl, "error out"=w1855:errorcluster)  [unwired: 10 in]
                    }
                    frame "sCsSU32" {
                      n610 = call-poly <vilib>:"ULx Read.vi"("task in"=w1863, "timeout"=w1858, "error in"=w1862) -> ("task out"=w1860:refnum<k24>, "data"=→"data 68":u32, "error out"=w1861:errorcluster)  [unwired: 10 in]
                    }
                    frame "sCnSDbl" {
                      n611 = call-poly <vilib>:"ULx Read.vi"("task in"=w1870, "number of samples per channel"="samples per", "timeout"=w1865, "error in"=w1869) -> ("task out"=w1867:refnum<k24>, "data"=w1864:dbl[], "error out"=w1868:errorcluster)  [unwired: 9 in]
                      "data 69" <- w1864
                      n612 = local write "Single Channel\n  1-D Array"(w1864) -> ()
                    }
                    frame "sCnSU32" {
                      n613 = call-poly <vilib>:"ULx Read.vi"("task in"=w1877, "number of samples per channel"="samples per", "timeout"=w1872, "error in"=w1876) -> ("task out"=w1874:refnum<k24>, "data"=w1871:u32[], "error out"=w1875:errorcluster)  [unwired: 9 in]
                      "data 70" <- w1871
                      n614 = local write "Single Channel\n  Unsigned 32-bit"(w1871) -> ()
                    }
                    frame "nCsSDbl" {
                      n615 = call-poly <vilib>:"ULx Read.vi"("task in"=w1883, "timeout"=w1878, "error in"=w1882) -> ("task out"=w1880:refnum<k24>, "data"=→"data 71":dbl[], "error out"=w1881:errorcluster)  [unwired: 10 in]
                    }
                    frame "nCsSU32" {
                      (unwired) "No equivalent NI function."
                      n616 = call-poly <vilib>:"ULx Read.vi"("task in"=w1889, "timeout"=w1884, "error in"=w1888) -> ("task out"=w1886:refnum<k24>, "data"=→"data 72":u32[], "error out"=w1887:errorcluster)  [unwired: 10 in]
                    }
                    frame "nCnSDbl" {
                      n617 = call-poly <vilib>:"ULx Read.vi"("task in"=w1896, "number of samples per channel"="samples per", "timeout"=w1891, "error in"=w1895) -> ("task out"=w1893:refnum<k24>, "data"=w1890:dbl[][], "error out"=w1894:errorcluster)  [unwired: 9 in]
                      "data 73" <- w1890
                      n618 = local write "Multi-channel\n  2-D Array"(w1890) -> ()
                    }
                    frame "nCnSU32" {
                      (unwired) "No equivalent NI function."
                      n619 = call-poly <vilib>:"ULx Read.vi"("task in"=w1903, "number of samples per channel"="samples per", "timeout"=w1898, "error in"=w1902) -> ("task out"=w1900:refnum<k24>, "data"=w1897:u32[][], "error out"=w1901:errorcluster)  [unwired: 9 in]
                      "data 74" <- w1897
                      n620 = local write "Multi-channel\n  Unsigned 32-bit"(w1897) -> ()
                    }
                  }
                }
                frame "Composite" {
                  n621 = case shown="\"1D Waveform\"" "CompRd" {
                    tunnel: w1911 -> [w1920 w1927]
                    tunnel: w1910 -> [w1919 w1928]
                    tunnel: [w1918 w1925] -> w1909
                    tunnel: [w1917 w1926] -> w1908
                    tunnel: w1907 -> [_ _]
                    tunnel: w1905 -> [w1916 w1922]
                    tunnel: "samples" -> [w1915 w1921]
                    frame "2D", Default {
                      n622 = call-poly <vilib>:"ULx Read.vi"("task in"=w1919, "number of samples per channel"=w1915, "timeout"=w1916, "error in"=w1920) -> ("task out"=w1918:refnum<k24>, "analog data"=w1912:dbl[][], "digital data"=w1913:u32[][], "counter data"=→"counter data":dbl[][], "error out"=w1917:errorcluster)  [unwired: 7 in]
                      "analog data 4" <- w1912
                      "digital data 3" <- w1913
                      n623 = local write "Multi-channel\n  Unsigned 32-bit"(w1913) -> ()
                      n624 = local write "Multi-channel\n  2-D Array"(w1912) -> ()
                    }
                    frame "1D Waveform" {
                      n625 = call-poly <vilib>:"ULx Read.vi"("task in"=w1928, "number of samples per channel"=w1921, "timeout"=w1922, "error in"=w1927) -> ("task out"=w1925:refnum<k24>, "analog data"=→"analog data 3":waveform(dbl)[], "digital data"=→"digital data 4":digitalwaveform[], "error out"=w1926:errorcluster)  [unwired: 7 in, 1 out]
                    }
                  }
                }
              }
            }
          }
          n626 = case shown="True" "Once" {
            frame False {
            }
            frame True {
              n627 = local write "Read"(FALSE ("Read")) -> ()
            }
          }
          n628 = local write "Read"(w1607) -> ()
        }
        frame 12 {
          # "WAIT"
          n629 = flat-sequence {
            tunnel: w1934 -> [w1941]
            tunnel: w1937 -> [w1942]
            tunnel: w1938 -> [w1943]
            tunnel: [w1943] -> w1933
            tunnel: [w1942] -> w1932
            tunnel: [w1941] -> w1931
            tunnel: w1930 -> [w1939]
            tunnel: [w1949] -> w1936
            tunnel: [w1948] -> w1935
            tunnel: w1933 -> [w1951]
            tunnel: w1932 -> [w1950]
            tunnel: w1931 -> [_]
            tunnel: [FALSE] -> w1929
            frame #0 {
              n630 = for {
                N: 5 -> [_]
                tunnel: w1939 -> [w1944]
                n631 = Wait Until Next ms Multiple(millisecond multiple=w1944) -> ()  [unwired: 1 out]
                "Wait" <- TRUE
              }
            }
            frame #1 {
              n632 = call <vilib>:"ULx Wait Until Done.vi"("task in"=w1950, "timeout"="timeout", "error in"=w1951) -> ("task out"=w1949:refnum<k24>, "error out"=w1948:errorcluster)  [unwired: 11 in]
            }
          }
          n633 = local write "Wait"(w1929) -> ()
        }
        frame 13 {
          # "Property Nodes"
          n634 = stacked-sequence {
            tunnel: w1958 -> [_ w1968]
            tunnel: w1957 -> [_ w1967]
            tunnel: w1956 -> [_ w1966]
            tunnel: [_ w1965] -> w1955
            tunnel: [_ w1964] -> w1954
            tunnel: w1953 -> [w1960 _]
            tunnel: [FALSE _] -> w1952
            frame #0 {
              n635 = for {
                N: 5 -> [_]
                tunnel: w1960 -> [w1962]
                n636 = Wait Until Next ms Multiple(millisecond multiple=w1962) -> ()  [unwired: 1 out]
                "Props" <- TRUE
              }
            }
            frame #1 {
              n637 = case shown="\"Get Properties\", Default" "GetSet" {
                tunnel: w1966 -> [w1974 w2509]
                tunnel: w1968 -> [w1973 w2511]
                tunnel: w1967 -> [w1972 w2508]
                tunnel: [w1971 w2506] -> w1965
                tunnel: [w1970 w2510] -> w1964
                frame "Get Properties", Default {
                  n638 = stacked-sequence {
                    seq-local: [w1978 _] -> [_ w2058]
                    seq-local: [w1977 _] -> [_ w2056]
                    tunnel: w1974 -> [w1980 _]
                    tunnel: w1973 -> [w1976 w2060]
                    tunnel: w1972 -> [w1979 _]
                    tunnel: [_ w2059] -> w1971
                    tunnel: [_ w2057] -> w1970
                    frame #0 {
                      n639 = for {
                        N: 3 -> [_]
                        tunnel: w1976 -> [w1988]
                        shift-right: [w1984] -> w1978
                        shift-left: w1980 -> [w1982]
                        shift-right: [w1985] -> w1977
                        shift-left: w1979 -> [w1993]
                        i -> [w1992]
                        n640 = case shown="2" w1992 {
                          tunnel: [w2002 w2006 w2010] -> w1991
                          frame 0, Default {
                            n641 = Select(t=1, s="Chans", f=0) -> (s? t:f=w2002:i32)
                          }
                          frame 1 {
                            n642 = Select(t=2, s="Done 2", f=0) -> (s? t:f=w2006:i32)
                          }
                          frame 2 {
                            n643 = Select(t=3, s="Err", f=0) -> (s? t:f=w2010:i32)
                          }
                        }
                        n644 = Not A Number/Path/Refnum?(number/path/refnum=w1982) -> (NaN/Path/Refnum?=w1981:bool)
                        n645 = case shown="3" w1991 {
                          tunnel: w1982 -> [w2015 w2022 w2040 w2046]
                          tunnel: w1993 -> [w2014 w2020 w2039 w2047]
                          tunnel: [w2015 w2021 w2038 w2044] -> w1987
                          tunnel: [w2014 w2023 w2037 w2043] -> w1986
                          tunnel: w1988 -> [_ _ _ _]
                          tunnel: [_ w2019 _ _] -> w1989
                          tunnel: w1981 -> [_ w2017 _ w2042]
                          frame 0, Default {
                          }
                          frame 1 {
                            n646 = case shown="False" w2017 {
                              tunnel: w2022 -> [w2024 w2033]
                              tunnel: [w2026 u32 0 ("NumberOfChannels")] -> w2018
                              tunnel: [w2027 w2034] -> w2023
                              tunnel: [w2028 w2033] -> w2021
                              tunnel: w2020 -> [w2030 w2034]
                              tunnel: [w2029 TRUE ("Done")] -> w2019
                              tunnel: [w2025 ""] -> w2016
                              frame False {
                                n647 = call "TaskProps.vi"("task in"=w2024, "error in (no error)"=w2030) -> ("task out"=w2028:refnum<k24>, "NumberOfChannels"=w2026:u32, "Done"=w2029:bool, "error out"=w2027:errorcluster, "DeviceName"=w2025:string)  [unwired: 1 in]
                              }
                              frame True {
                              }
                            }
                            "Done" <- w2019
                            "NumChans" <- w2018
                            "DevName" <- w2016
                          }
                          frame 2 {
                            n648 = call <vilib>:"ULx Is Task Done.vi"("task in"=w2040, "error in"=w2039) -> ("task out"=w2038:refnum<k24>, "task done?"=→"IT Done":bool, "error out"=w2037:errorcluster)  [unwired: 11 in]
                          }
                          frame 3 {
                            n649 = case shown="False" w2042 {
                              tunnel: w2046 -> [w2052 w2055]
                              tunnel: w2047 -> [w2051 w2054]
                              tunnel: [w2050 0 ("ErrorCode")] -> w2045
                              tunnel: [w2049 w2054] -> w2041
                              tunnel: [w2048 w2055] -> w2044
                              frame False {
                                n650 = property class="IOTask"(reference=w2052, error in=w2051) -> (reference out=w2048:refnum<k24>, error out=w2049:errorcluster, "ErrorCode"=w2050:i32)
                              }
                              frame True {
                              }
                            }
                            "ErrorCode" <- w2045
                            n651 = call <vilib>:"ULx Get Error Info.vi"("error in"=w2041, "ErrorCode"=w2045, "task in"=w2044) -> ("error out"=w2043:errorcluster)  [unwired: 8 in]
                          }
                        }
                        n652 = And(x=w1989, y="Restart\nWhen\nDone") -> (x .and. y?=w1990:bool)
                        n653 = case shown="False" w1990 {
                          tunnel: w1988 -> [_ _]
                          tunnel: w1987 -> [w1995 w1999]
                          tunnel: w1986 -> [w1994 w2001]
                          tunnel: [w1994 w2000] -> w1985
                          tunnel: [w1995 w1998] -> w1984
                          frame False {
                          }
                          frame True {
                            n654 = call <vilib>:"ULx Stop Task.vi"("error in"=w2001, "task in"=w1999) -> ("error out"=w1996:errorcluster, "task out"=w1997:refnum<k24>)  [unwired: 8 in]
                            n655 = call <vilib>:"ULx Start Task.vi"("task in"=w1997, "error in"=w1996) -> ("task out"=w1998:refnum<k24>, "error out"=w2000:errorcluster)  [unwired: 12 in]
                          }
                        }
                      }
                    }
                    frame #1 {
                      n656 = case shown="No Error" w2056 {
                        tunnel: "GetLev" -> [w2067 _]
                        tunnel: w2060 -> [w2066 _]
                        tunnel: [w2065 w2504] -> w2059
                        tunnel: w2058 -> [w2064 w2505]
                        tunnel: w2056 -> [w2063 w2504]
                        tunnel: [w2062 w2505] -> w2057
                        frame No Error {
                          n657 = case shown="\"Timing\"" w2067 {
                            tunnel: w2064 -> [w2069 w2164 w2254 w2357 w2419 w2437 w2503]
                            tunnel: w2066 -> [w2073 w2166 w2250 w2353 w2417 w2434 _]
                            tunnel: w2063 -> [w2068 w2165 w2253 w2356 w2418 w2438 w2502]
                            tunnel: [w2072 w2162 w2251 w2354 w2415 w2436 w2500] -> w2065
                            tunnel: [w2070 w2163 w2252 w2355 w2416 w2435 w2501] -> w2062
                            frame "Read", Default {
                              n658 = for {
                                N: 8 -> [_]
                                tunnel: w2073 -> [w2080]
                                shift-right: [w2076] -> w2070
                                shift-left: w2069 -> [w2075]
                                shift-right: [w2079] -> w2072
                                shift-left: w2068 -> [w2074]
                                i -> [w2078]
                                n659 = case shown="0, Default" w2078 {
                                tunnel: [w2081 w2088 w2090 w2093 w2097 w2101 w2106 w2109] -> w2077
                                frame 0, Default {
                                n660 = Select(t=1, s="AutoS", f=0) -> (s? t:f=w2081:i32)
                                }
                                frame 1 {
                                n661 = Select(t=2, s="Avail", f=0) -> (s? t:f=w2088:i32)
                                }
                                frame 2 {
                                n662 = Select(t=3, s="Position", f=0) -> (s? t:f=w2090:i32)
                                }
                                frame 3 {
                                n663 = Select(t=4, s="OWrite", f=0) -> (s? t:f=w2093:i32)
                                }
                                frame 4 {
                                n664 = Select(t=5, s="ReadAll", f=0) -> (s? t:f=w2097:i32)
                                }
                                frame 5 {
                                n665 = Select(t=6, s="Total", f=0) -> (s? t:f=w2101:i32)
                                }
                                frame 6 {
                                n666 = Select(t=7, s="Raw", f=0) -> (s? t:f=w2106:i32)
                                }
                                frame 7 {
                                n667 = Select(t=8, s="Bools", f=0) -> (s? t:f=w2109:i32)
                                }
                                }
                                n668 = case shown="2" w2077 {
                                tunnel: w2080 -> [_ _ _ _ _ _ _ _ _]
                                tunnel: w2075 -> [w2113 w2119 w2128 w2134 w2137 w2145 w2150 w2155 w2160]
                                tunnel: w2074 -> [w2114 w2118 w2127 w2133 w2138 w2144 w2149 w2154 w2159]
                                tunnel: [w2114 w2117 w2126 w2132 w2135 w2142 w2147 w2152 w2157] -> w2079
                                tunnel: [w2113 w2115 w2125 w2131 w2136 w2143 w2148 w2153 w2158] -> w2076
                                frame 0, Default {
                                }
                                frame 1 {
                                n669 = call "ReadAutoStart.vi"("error in (no error)"=w2118, "task in"=w2119) -> ("error out"=w2117:errorcluster, "AutoStart"=→"AutoStart":bool, "task out"=w2115:refnum<k24>)  [unwired: 1 in]
                                }
                                frame 2 {
                                n670 = call "AvailableSamps.vi"("error in (no error)"=w2127, "task in"=w2128) -> ("error out"=w2126:errorcluster, "AvailableSamples"=w2124:u32, "task out"=w2125:refnum<k24>)  [unwired: 1 in]
                                "Available Samples" <- w2124
                                n671 = Greater?(x=w2124, y="Read when Available Samples is greater than this") -> (0:w2122:bool)
                                n672 = local write "Once"("y 2") -> ()
                                n673 = And(x=w2122, y="y 2") -> (x .and. y?=w2121:bool)
                                n674 = case shown="True" w2121 {
                                frame False {
                                }
                                frame True {
                                n675 = local write "Read"(TRUE ("Read")) -> ()
                                }
                                }
                                }
                                frame 3 {
                                n676 = call "CurrentReadPosition.vi"("error in (no error)"=w2133, "task in"=w2134) -> ("error out"=w2132:errorcluster, "CurrReadPosition"=→"CurrReadPos":u32, "task out"=w2131:refnum<k24>)  [unwired: 1 in]
                                }
                                frame 4 {
                                n677 = property class="IOTask"(reference=w2137, error in=w2138) -> (reference out=w2136:refnum<k24>, error out=w2135:errorcluster, "Read.AutoStatus"=→"AutoStatus":bool)
                                "OverWrite (Obs)" <- FALSE
                                }
                                frame 5 {
                                n678 = call "ReadAllData.vi"("error in (no error)"=w2144, "task in"=w2145) -> ("error out"=w2142:errorcluster, "ReadAll"=→"ReadAllAvailSamp":bool, "task out"=w2143:refnum<k24>)  [unwired: 1 in]
                                }
                                frame 6 {
                                n679 = call "TotalAcquired.vi"("error in (no error)"=w2149, "task in"=w2150) -> ("error out"=w2147:errorcluster, "TotalAcquired"=→"TotalPerAcquired":u32, "task out"=w2148:refnum<k24>)  [unwired: 1 in]
                                }
                                frame 7 {
                                n680 = call "ReadRawData.vi"("error in (no error)"=w2154, "task in"=w2155) -> ("error out"=w2152:errorcluster, "ReadRaw"=→"RawData":bool, "task out"=w2153:refnum<k24>)  [unwired: 1 in]
                                }
                                frame 8 {
                                n681 = call "NumberOfBools.vi"("error in (no error)"=w2159, "task in"=w2160) -> ("error out"=w2157:errorcluster, "NumberOfBools"=→"NumberOfBoolsPer":u32, "task out"=w2158:refnum<k24>)  [unwired: 1 in]
                                }
                                }
                              }
                            }
                            frame "Write" {
                              n682 = for {
                                N: 7 -> [_]
                                tunnel: w2166 -> [w2173]
                                shift-right: [w2170] -> w2163
                                shift-left: w2164 -> [w2171]
                                shift-right: [w2169] -> w2162
                                shift-left: w2165 -> [w2172]
                                i -> [w2168]
                                n683 = case shown="1" w2168 {
                                tunnel: [w2174 w2178 w2182 w2186 w2190 w2194 _] -> w2167
                                frame 0, Default {
                                n684 = Select(t=1, s="WrtPos", f=0) -> (s? t:f=w2174:i32)
                                }
                                frame 1 {
                                n685 = Select(t=2, s="Reg 2", f=0) -> (s? t:f=w2178:i32)
                                }
                                frame 2 {
                                n686 = Select(t=3, s="Gen", f=0) -> (s? t:f=w2182:i32)
                                }
                                frame 3 {
                                n687 = Select(t=4, s="Space", f=0) -> (s? t:f=w2186:i32)
                                }
                                frame 4 {
                                n688 = Select(t=5, s="Bools 2", f=0) -> (s? t:f=w2190:i32)
                                }
                                frame 5 {
                                n689 = Select(t=6, s="RelTo", f=0) -> (s? t:f=w2194:i32)
                                }
                                frame 6 {
                                n690 = Select(t=7, s="Offset 2", f=0) -> ()  [unwired: 1 out]
                                }
                                }
                                n691 = case shown="1" w2167 {
                                tunnel: w2173 -> [_ _ _ _ _ _ _ _]
                                tunnel: w2172 -> [w2201 w2207 w2211 w2216 w2229 w2242 w2244 w2249]
                                tunnel: w2171 -> [w2202 w2206 w2212 w2217 w2230 w2241 w2243 w2248]
                                tunnel: [w2202 w2205 w2210 w2215 w2232 w2241 w2243 w2247] -> w2170
                                tunnel: [w2201 w2204 w2209 w2214 w2231 w2242 w2244 w2246] -> w2169
                                frame 0, Default {
                                }
                                frame 1 {
                                n692 = call "CurrWritePos.vi"("error in (no error)"=w2207, "task in"=w2206) -> ("error out"=w2204:errorcluster, "CurrWritePos"=→"CurrentWritePosition":u32, "task out"=w2205:refnum<k24>)  [unwired: 1 in]
                                }
                                frame 2 {
                                n693 = call "WriteRegen.vi"("error in (no error)"=w2211, "task in"=w2212) -> ("error out"=w2209:errorcluster, "Regenerate"=→"Regenerate":bool, "task out"=w2210:refnum<k24>)  [unwired: 1 in]
                                }
                                frame 3 {
                                n694 = call "SamplesGenerated.vi"("error in (no error)"=w2216, "task in"=w2217) -> ("error out"=w2214:errorcluster, "SamplesGenerated"=→"Generated":u32, "task out"=w2215:refnum<k24>)  [unwired: 1 in]
                                }
                                frame 4 {
                                n695 = property class="IOTask"(reference=w2230, error in=w2229) -> (reference out=w2228:refnum<k24>, error out=w2227:errorcluster, "Write.SpaceAvailable"=w2223:u32)
                                "SpaceAvailable" <- w2223
                                n696 = local read "Regenerate"() -> (w2220:bool)
                                n697 = call "SpaceAvailable.vi"("error in (no error)"=w2227, "task in"=w2228) -> ("error out"=w2231:errorcluster, "SpaceAvailable"=w2226:u32, "task out"=w2232:refnum<k24>)  [unwired: 1 in]
                                "CWP - Generated" <- w2226
                                n698 = case shown="True" "Space 2" {
                                tunnel: [w2236 w2240] -> w2219
                                tunnel: w2226 -> [w2235 _]
                                tunnel: "Start when \"SpaceAvailable\"" -> [w2234 w2239]
                                tunnel: w2223 -> [_ w2238]
                                tunnel: ["< this." ("String 2") "> this." ("String 2")] -> w2222
                                frame False {
                                n699 = Less?(x=w2235, y=w2234) -> (x < y?=w2236:bool)
                                }
                                frame True {
                                n700 = Greater?(x=w2238, y=w2239) -> (0:w2240:bool)
                                }
                                }
                                "String 2" <- w2222
                                n701 = Not(x=w2220) -> (.not. x?=w2218:bool)
                                n702 = And(x=w2218, y=w2219) -> (x .and. y?=w2221:bool)
                                n703 = local write "Write"(w2221) -> ()
                                }
                                frame 6 {
                                }
                                frame 7 {
                                }
                                frame 5 {
                                n704 = call "NumberOfBoolsWr.vi"("error in (no error)"=w2249, "task in"=w2248) -> ("error out"=w2246:errorcluster, "NumBoolsWr"=→"BooleansPer":u32, "task out"=w2247:refnum<k24>)  [unwired: 1 in]
                                }
                                }
                              }
                            }
                            frame "Trigger" {
                              n705 = stacked-sequence {
                                seq-local: [w2257 _] -> [_ w2262]
                                seq-local: [w2256 _] -> [_ w2261]
                                tunnel: w2254 -> [w2258 _]
                                tunnel: w2253 -> [w2259 _]
                                tunnel: [_ w2265] -> w2252
                                tunnel: [_ w2264] -> w2251
                                tunnel: w2250 -> [_ w2263]
                                frame #0 {
                                n706 = call "TrigMode.vi"("error in (no error)"=w2259, "task in"=w2258) -> ("error out"=w2256:errorcluster, "TrigMode"=→"Mode":i32, "task out"=w2257:refnum<k24>)  [unwired: 1 in]
                                }
                                frame #1 {
                                n707 = case shown="\"Basic\", Default" "GtULxTrgP" {
                                tunnel: [w2271 w2322 w2337 w2350] -> w2265
                                tunnel: [w2270 w2321 w2336 w2348] -> w2264
                                tunnel: w2263 -> [w2269 _ _ _]
                                tunnel: w2262 -> [w2267 w2324 w2339 w2351]
                                tunnel: w2261 -> [w2266 w2323 w2338 w2349]
                                frame "Basic", Default {
                                n708 = for {
                                N: 3 -> [_]
                                shift-right: [w2276] -> w2271
                                shift-left: w2267 -> [w2278]
                                shift-right: [w2275] -> w2270
                                shift-left: w2266 -> [w2277]
                                tunnel: w2269 -> [w2274]
                                i -> [w2273]
                                n709 = case shown="2" w2273 {
                                tunnel: [w2299 w2303 w2307] -> w2272
                                frame 0, Default {
                                n710 = Select(t=1, s="Type", f=0) -> (s? t:f=w2299:i32)
                                }
                                frame 1 {
                                n711 = Select(t=2, s="Edge", f=0) -> (s? t:f=w2303:i32)
                                }
                                frame 2 {
                                n712 = Select(t=3, s="Other", f=0) -> (s? t:f=w2307:i32)
                                }
                                }
                                n713 = case shown="0, Default" w2272 {
                                tunnel: w2278 -> [w2280 w2285 w2289 w2297]
                                tunnel: w2277 -> [w2279 w2284 w2290 w2298]
                                tunnel: [w2280 w2283 w2288 w2295] -> w2276
                                tunnel: [w2279 w2282 w2287 w2296] -> w2275
                                tunnel: w2274 -> [_ _ _ _]
                                frame 0, Default {
                                }
                                frame 1 {
                                n714 = call "TrigBasicType.vi"("error in (no error)"=w2284, "task in"=w2285) -> ("error out"=w2282:errorcluster, "TrigType"=→"Type":i32, "task out"=w2283:refnum<k24>)  [unwired: 1 in]
                                }
                                frame 2 {
                                n715 = call "TrigBasicEdge.vi"("error in (no error)"=w2290, "task in"=w2289) -> ("error out"=w2287:errorcluster, "TrigEdge"=→"Edge":i32, "task out"=w2288:refnum<k24>)  [unwired: 1 in]
                                }
                                frame 3 {
                                n716 = call "TrigBasicProps.vi"("task in"=w2297, "error in (no error)"=w2298) -> ("Slope"=→"Slope":i32, "PretriggerCount"=→"PretriggerCount":i32, "task out"=w2295:refnum<k24>, "DigLevel"=→"DigitalLevel":i32, "AnalogLevel"=→"AnalogLevel":dbl, "error out"=w2296:errorcluster)  [unwired: 1 in]
                                }
                                }
                                }
                                }
                                frame "Gated" {
                                n717 = call "TrigGatedProps.vi"("task in"=w2324, "error in (no error)"=w2323) -> ("When"=→"When":i32, "Hysteresis"=→"Hysteresis":i32, "Position"=→"Position":i32, "WindowBottom"=→"WindowBottom":dbl, "Type"=→"Type":i32, "WindowTop"=→"WindowTop":dbl, "task out"=w2322:refnum<k24>, "AnalogLevel"=→"AnalogLevel":dbl, "DigitalLevel"=→"DigitalLevel":i32, "HighThreshold"=→"HighThreshold":dbl, "LowThreshold"=→"LowThreshold":dbl, "error out"=w2321:errorcluster)  [unwired: 6 in]
                                }
                                frame "Start" {
                                n718 = call "CompTrigStartProps.vi"("task in"=w2339, "error in (no error)"=w2338) -> ("AnalogHWTrigSense"=→"AnalogHWSense":i32, "TrigChannelStr"=→"TriggerChannelStr":string, "AnalogSWTrigSense"=→"AnalogSWSense":i32, "TriggerChannel"=→"Channel":i32, "CounterChanTrigSense"=→"CounterChannelSense":i32, "Variance"=→"Variance":dbl, "DigitalPatternTrigSense"=→"DigitalPatternSense":i32, "task out"=w2337:refnum<k24>, "Level"=→"Level":dbl, "Type"=→"Type":i32, "PretriggerCount"=→"PretriggerCount":i32, "ExtTTLTrigSense"=→"ExtTTLSense":i32, "error out"=w2336:errorcluster)  [unwired: 5 in]
                                }
                                frame "Stop" {
                                n719 = call "CompTrigStopProps.vi"("task in"=w2351, "error in (no error)"=w2349) -> ("TriggerChannelStr"=→"TriggerChannelStr":string, "AnalogSWTriggerSense"=→"AnalogSWSense":i32, "TriggerChannel"=→"Channel":i32, "CounterChannelTriggerSense"=→"CounterChannelSense":i32, "Variance"=→"Variance":dbl, "DigitalPatternTriggerSense"=→"DigitalPatternSense":i32, "task out"=w2350:refnum<k24>, "Level"=→"Level":dbl, "Type"=→"Type":i32, "error IO"=w2348:errorcluster)  [unwired: 8 in]
                                }
                                }
                                }
                              }
                            }
                            frame "Timing" {
                              n720 = for {
                                N: 5 -> [_]
                                shift-right: [w2362] -> w2355
                                shift-left: w2357 -> [w2364]
                                shift-right: [w2361] -> w2354
                                shift-left: w2356 -> [w2363]
                                tunnel: w2353 -> [w2360]
                                i -> [w2359]
                                n721 = case shown="4" w2359 {
                                tunnel: [w2392 w2396 w2400 w2404 w2411] -> w2358
                                frame 0, Default {
                                n722 = Select(t=1, s="Burst", f=0) -> (s? t:f=w2392:i32)
                                }
                                frame 1 {
                                n723 = Select(t=2, s="SIO", f=0) -> (s? t:f=w2396:i32)
                                }
                                frame 2 {
                                n724 = Select(t=3, s="DiWord", f=0) -> (s? t:f=w2400:i32)
                                }
                                frame 3 {
                                n725 = Select(t=4, s="DoWord", f=0) -> (s? t:f=w2404:i32)
                                }
                                frame 4 {
                                n726 = Or(x="UFlow", y="Actual Rate") -> (x .or. y?=w2409:bool)
                                n727 = Select(t=5, s=w2409, f=0) -> (s? t:f=w2411:i32)
                                }
                                }
                                n728 = case shown="1" w2358 {
                                tunnel: w2364 -> [w2366 w2371 w2373 w2379 w2386 w2391]
                                tunnel: w2363 -> [w2365 w2370 w2374 w2380 w2385 w2390]
                                tunnel: [w2366 w2368 w2373 w2378 w2384 w2389] -> w2362
                                tunnel: [w2365 w2367 w2374 w2377 w2383 w2388] -> w2361
                                tunnel: w2360 -> [_ _ _ _ _ _]
                                frame 0, Default {
                                }
                                frame 1 {
                                n729 = property class="IOTask"(reference=w2371, error in=w2370) -> (reference out=w2368:refnum<k24>, error out=w2367:errorcluster, "Timing.BurstIO"=→"BurstIO":bool)
                                }
                                frame 2 {
                                "SingleIO" <- FALSE ("SingleIO")
                                }
                                frame 3 {
                                n730 = call "DIWordXfer.vi"("error in (no error)"=w2380, "task in"=w2379) -> ("error out"=w2377:errorcluster, "DIDWord (obs)"=→"DI.DWord (obs)":bool, "DIWord"=→"DI.Word Xfer":bool, "task out"=w2378:refnum<k24>)
                                }
                                frame 4 {
                                n731 = call "DOWordXfer.vi"("error in (no error)"=w2385, "task in"=w2386) -> ("error out"=w2383:errorcluster, "DODWord (obs)"=→"DO.DWord (obs)":bool, "DOWord"=→"DO.Word Xfer":bool, "task out"=w2384:refnum<k24>)
                                }
                                frame 5 {
                                n732 = call "TimingRate.vi"("error in (no error)"=w2390, "task in"=w2391) -> ("error out"=w2388:errorcluster, "ActualRate"=→"Timing.ActualRate":sgl, "task out"=w2389:refnum<k24>)  [unwired: 1 in]
                                }
                                }
                              }
                            }
                            frame "AI" {
                              n733 = case shown="True" "Units" {
                                tunnel: w2419 -> [w2421 w2426]
                                tunnel: w2418 -> [w2420 w2425]
                                tunnel: w2417 -> [_ w2424]
                                tunnel: [w2421 w2423] -> w2416
                                tunnel: [w2420 w2422] -> w2415
                                frame False {
                                }
                                frame True {
                                n734 = stacked-sequence {
                                seq-local: [w2427 _] -> [_ w2431]
                                seq-local: [w2428 _] -> [_ w2430]
                                tunnel: w2426 -> [w2427 _]
                                tunnel: w2425 -> [w2428 _]
                                tunnel: w2424 -> [_ _]
                                tunnel: [_ w2433] -> w2423
                                tunnel: [_ w2432] -> w2422
                                frame #0 {
                                }
                                frame #1 {
                                n735 = call "TempUnits.vi"("error in (no error)"=w2430, "task in"=w2431) -> ("error out"=w2432:errorcluster, "Temp.Units"=→"Channel.AI.Temp.Units":i32, "task out"=w2433:refnum<k24>)  [unwired: 1 in]
                                }
                                }
                                }
                              }
                            }
                            frame "CI" {
                              n736 = stacked-sequence {
                                seq-local: [w2439 _] -> [_ w2444]
                                seq-local: [w2440 _] -> [_ w2443]
                                tunnel: w2438 -> [w2440 _]
                                tunnel: w2437 -> [w2439 _]
                                tunnel: [_ w2446] -> w2436
                                tunnel: [_ w2445] -> w2435
                                tunnel: w2434 -> [_ w2442]
                                frame #0 {
                                }
                                frame #1 {
                                n737 = case shown="\"ULx\", Default" w2442 {
                                tunnel: ["CIType" "GetmxCIPrp"] -> w2441
                                frame "ULx", Default {
                                }
                                frame "DAQMx" {
                                }
                                }
                                n738 = case shown="\"Frequency\", Default" w2441 {
                                tunnel: w2443 -> [w2455 w2461 w2484 w2493]
                                tunnel: w2444 -> [w2453 w2462 w2482 w2492]
                                tunnel: [w2454 w2459 w2483 w2490] -> w2446
                                tunnel: [w2452 w2460 w2481 w2491] -> w2445
                                tunnel: w2442 -> [_ _ _ _]
                                frame "Frequency", Default {
                                n739 = call "CIFreqProps.vi"("task in"=w2453, "error in (no error)"=w2455) -> ("task out"=w2452:refnum<k24>, "StartingEdge"=→"StartingEdge":i32, "Units"=→"Units":i32, "error out"=w2454:errorcluster, "MeasurementTime"=→"MeasurementTime":dbl)  [unwired: 1 in]
                                }
                                frame "Period" {
                                n740 = call "CIPeriodProps.vi"("task in"=w2462, "error in (no error)"=w2461) -> ("task out"=w2460:refnum<k24>, "StartingEdge"=→"StartingEdge":i32, "Units"=→"Units":i32, "error out"=w2459:errorcluster, "MeasurementTime"=→"MeasurementTime":dbl)  [unwired: 1 in]
                                }
                                frame "Edges" {
                                n741 = call "CIEdgesProps.vi"("task in"=w2482, "error in (no error)"=w2484) -> ("task out"=w2470:refnum<k24>, "Edge"=→"Edge":i32, "InitialCount"=→"InitialCount":u32, "error out"=w2469:errorcluster, "Direction"=→"MccDirection":i32, "Gate Function"=→"Gate Function":i32)
                                n742 = call "CtrCntrl.vi"("error in (no error)"=w2469, ".NET Refnum"=w2470) -> ("InvertGate"=→"InvertGate":bool, "Recycle"=→"Recycle":bool, "error out"=w2465:errorcluster, ".NET Refnum 2"=w2466:refnum<k24>, "OutputVal1"=→"Val 1":u64, "MinLimit"=→"Min":u64, "OutputVal0"=→"Val 0":u64, "MaxLimit"=→"Max":u64, "OutputOn"=→"Output":bool, "RangeLimitOn"=→"Range Limit":bool)
                                n743 = call "CtrProps.vi"("error in (no error)"=w2465, ".NET Refnum 2"=w2466) -> ("InitialState"=→"InitialState":i32, "ClearOnRead"=→"ClearOnRead":bool, "error out"=w2483:errorcluster, ".NET Refnum"=w2481:refnum<k24>)  [unwired: 6 in]
                                }
                                frame "Encoder" {
                                n744 = call "CIEncoderProps.vi"("task in"=w2492, "error in (no error)"=w2493) -> ("Units"=→"Units":i32, "DecodingType"=→"DecodingType":i32, "task out"=w2491:refnum<k24>, "PulsesPerRevolution"=→"PulsesPerRev":i32, "InitialAngle"=→"InitialAngle":dbl, "ZIndexMode"=→"ZIndexMode":i32, "error out"=w2490:errorcluster)  [unwired: 2 in]
                                }
                                }
                                }
                              }
                            }
                            frame "CO" {
                              n745 = call "COPulseProps.vi"("task in"=w2503, "error in (no error)"=w2502) -> ("DutyCycle"=→"DutyCycle":dbl, "HighTicks"=→"HighTicks":u32, "HighTime"=→"HighTime":dbl, "task out"=w2501:refnum<k24>, "LowTicks"=→"LowTicks":u32, "Frequency"=→"Frequency":dbl, "LowTime"=→"LowTime":dbl, "error out"=w2500:errorcluster)  [unwired: 1 in]
                            }
                          }
                        }
                        frame Error {
                        }
                      }
                    }
                  }
                }
                frame "Set Properties" {
                  n746 = case shown="\"Read\", Default" "SetLev" {
                    tunnel: w2511 -> [w2517 w2557 _ w2611 _ w2661 w2776]
                    tunnel: [w2515 w2559 w2605 w2608 w2658 w2663 w2772] -> w2510
                    tunnel: w2509 -> [w2514 w2561 w2605 w2609 w2658 w2660 w2774]
                    tunnel: w2508 -> [w2513 w2560 w2604 w2610 w2657 w2659 w2775]
                    tunnel: [w2512 w2558 w2604 w2607 w2657 w2664 w2771] -> w2506
                    frame "Read", Default {
                      n747 = for {
                        N: 3 -> [_]
                        tunnel: w2517 -> [w2522]
                        shift-right: [w2524] -> w2515
                        shift-left: w2514 -> [w2519]
                        shift-right: [w2523] -> w2512
                        shift-left: w2513 -> [w2518]
                        i -> [w2521]
                        n748 = case shown="0, Default" w2521 {
                          tunnel: [w2525 w2529 w2533] -> w2520
                          frame 0, Default {
                            n749 = Select(t=1, s="Auto", f=0) -> (s? t:f=w2525:i32)
                          }
                          frame 1 {
                            n750 = Select(t=2, s="OWrite", f=0) -> (s? t:f=w2529:i32)
                          }
                          frame 2 {
                            n751 = Select(t=3, s="ReadAll 2", f=0) -> (s? t:f=w2533:i32)
                          }
                        }
                        n752 = case shown="2" w2520 {
                          tunnel: w2519 -> [w2538 w2544 w2548 w2556]
                          tunnel: w2518 -> [w2537 w2543 w2549 w2555]
                          tunnel: [w2538 w2542 w2546 w2554] -> w2524
                          tunnel: [w2537 w2541 w2547 w2553] -> w2523
                          tunnel: w2522 -> [_ _ _ _]
                          frame 0, Default {
                          }
                          frame 1 {
                            n753 = call "SetReadAutostart.vi"("error in (no error)"=w2543, "Read.AutoStart"="Read.AutoStart", "task in"=w2544) -> ("error out"=w2541:errorcluster, "task out"=w2542:refnum<k24>)
                            n754 = local write "Auto"(FALSE ("Auto")) -> ()
                          }
                          frame 2 {
                            n755 = property class="IOTask"(reference=w2548, error in=w2549, "Read.AutoStatus"="AutoStatus 2") -> (reference out=w2546:refnum<k24>, error out=w2547:errorcluster)
                            n756 = local write "OWrite"(FALSE ("Auto 2")) -> ()
                          }
                          frame 3 {
                            n757 = call "SetReadAllData.vi"("error in (no error)"=w2555, "Read.AllData"="ReadAllAvailSamp", "task in"=w2556) -> ("error out"=w2553:errorcluster, "task out"=w2554:refnum<k24>)
                            n758 = local write "ReadAll 2"(FALSE ("ReadAll 2")) -> ()
                          }
                        }
                      }
                    }
                    frame "Write" {
                      n759 = for {
                        N: 4 -> [_]
                        shift-right: [w2566] -> w2559
                        shift-left: w2561 -> [w2567]
                        shift-right: [w2568] -> w2558
                        shift-left: w2560 -> [w2569]
                        tunnel: w2557 -> [w2563]
                        i -> [w2565]
                        n760 = case shown="0, Default" w2565 {
                          tunnel: [w2570 w2574 w2578 w2582] -> w2564
                          frame 0, Default {
                            n761 = Select(t=1, s="WrtPos", f=0) -> (s? t:f=w2570:i32)
                          }
                          frame 1 {
                            n762 = Select(t=2, s="Reg", f=0) -> (s? t:f=w2574:i32)
                          }
                          frame 2 {
                            n763 = Select(t=3, s="Rel", f=0) -> (s? t:f=w2578:i32)
                          }
                          frame 3 {
                            n764 = Select(t=4, s="Offset 3", f=0) -> (s? t:f=w2582:i32)
                          }
                        }
                        n765 = case shown="0, Default" w2564 {
                          tunnel: w2569 -> [w2586 w2593 w2599 w2600 w2602]
                          tunnel: [w2586 w2592 w2596 w2600 w2602] -> w2568
                          tunnel: w2567 -> [w2587 w2591 w2598 w2601 w2603]
                          tunnel: [w2587 w2590 w2597 w2601 w2603] -> w2566
                          tunnel: w2563 -> [_ _ _ _ _]
                          frame 0, Default {
                          }
                          frame 1 {
                            n766 = call "SetCurWrtPos.vi"("error in (no error)"=w2593, "CurrentWritePosition"="CurrentWritePosition", "task in"=w2591) -> ("error out"=w2592:errorcluster, "task out"=w2590:refnum<k24>)
                            n767 = local write "WrtPos"(FALSE ("WrtPos")) -> ()
                          }
                          frame 2 {
                            n768 = call "SetWrtRegen.vi"("error in (no error)"=w2599, "Regenerate"="Regenerate", "task in"=w2598) -> ("error out"=w2596:errorcluster, "task out"=w2597:refnum<k24>)
                            n769 = local write "Reg"(FALSE ("Reg")) -> ()
                          }
                          frame 3 {
                          }
                          frame 4 {
                          }
                        }
                      }
                    }
                    frame "Trigger" {
                    }
                    frame "Timing" {
                      n770 = for {
                        N: 4 -> [_]
                        tunnel: w2611 -> [w2618]
                        shift-right: [w2615] -> w2608
                        shift-left: w2609 -> [w2616]
                        shift-right: [w2614] -> w2607
                        shift-left: w2610 -> [w2617]
                        i -> [w2613]
                        n771 = case shown="0, Default" w2613 {
                          tunnel: [w2619 w2623 w2627 w2631] -> w2612
                          frame 0, Default {
                            n772 = Select(t=1, s="BurstIO 3", f=0) -> (s? t:f=w2619:i32)
                          }
                          frame 1 {
                            n773 = Select(t=2, s="SingleIO 3", f=0) -> (s? t:f=w2623:i32)
                          }
                          frame 2 {
                            n774 = Select(t=3, s="DIWord", f=0) -> (s? t:f=w2627:i32)
                          }
                          frame 3 {
                            n775 = Select(t=4, s="DOWord 2", f=0) -> (s? t:f=w2631:i32)
                          }
                        }
                        n776 = case shown="3" w2612 {
                          tunnel: w2618 -> [_ _ _ _ _]
                          tunnel: w2617 -> [w2635 w2638 w2641 w2649 w2655]
                          tunnel: w2616 -> [w2636 w2639 w2642 w2648 w2656]
                          tunnel: [w2636 w2639 w2642 w2647 w2653] -> w2615
                          tunnel: [w2635 w2638 w2641 w2646 w2654] -> w2614
                          frame 0, Default {
                          }
                          frame 1 {
                            n777 = local write "BurstIO 3"(FALSE ("BurstIO 3")) -> ()
                          }
                          frame 2 {
                            n778 = local write "SingleIO 3"(FALSE ("SingleIO 2")) -> ()
                          }
                          frame 3 {
                            n779 = call "SetDIWord.vi"("error in (no error)"=w2649, "DIDWord (obs)"="DIDWord", "DIWord"="DIWord", "task in"=w2648) -> ("error out"=w2646:errorcluster, "task out"=w2647:refnum<k24>)
                            n780 = local write "DIWord"(FALSE ("DIWord")) -> ()
                          }
                          frame 4 {
                            n781 = call "SetDOWord.vi"("error in (no error)"=w2655, "DODWord (obs)"="DODWord", "DOWord"="DOWord", "task in"=w2656) -> ("error out"=w2654:errorcluster, "task out"=w2653:refnum<k24>)
                            n782 = local write "DOWord 2"(FALSE ("DOWord 2")) -> ()
                          }
                        }
                      }
                    }
                    frame "AI" {
                    }
                    frame "CI" {
                      n783 = for {
                        N: 11 -> [_]
                        tunnel: w2661 -> [w2671]
                        shift-right: [w2669] -> w2664
                        shift-left: w2659 -> [w2670]
                        shift-right: [w2667] -> w2663
                        shift-left: w2660 -> [w2668]
                        i -> [w2666]
                        n784 = case shown="10" w2666 {
                          tunnel: [w2727 w2731 w2738 w2739 w2743 w2747 w2751 w2755 w2759 w2763 w2767] -> w2665
                          frame 0, Default {
                            n785 = Select(t=1, s="MinMax", f=0) -> (s? t:f=w2727:i32)
                          }
                          frame 1 {
                            n786 = Select(t=2, s="Set Dir", f=0) -> (s? t:f=w2731:i32)
                          }
                          frame 2 {
                            n787 = Select(t=3, s="Gate", f=0) -> (s? t:f=w2738:i32)
                          }
                          frame 3 {
                            n788 = Select(t=4, s="ClearOnRead 2", f=0) -> (s? t:f=w2739:i32)
                          }
                          frame 4 {
                            n789 = Select(t=5, s="RangeLimit", f=0) -> (s? t:f=w2743:i32)
                          }
                          frame 5 {
                            n790 = Select(t=6, s="OutputOn", f=0) -> (s? t:f=w2747:i32)
                          }
                          frame 6 {
                            n791 = Select(t=7, s="NoRecycle", f=0) -> (s? t:f=w2751:i32)
                          }
                          frame 7 {
                            n792 = Select(t=8, s="Invert Gate", f=0) -> (s? t:f=w2755:i32)
                          }
                          frame 8 {
                            n793 = Select(t=9, s="Mcc Direction", f=0) -> (s? t:f=w2759:i32)
                          }
                          frame 9 {
                            n794 = Select(t=10, s="Mcc Edge", f=0) -> (s? t:f=w2763:i32)
                          }
                          frame 10 {
                            n795 = Select(t=11, s="Init State", f=0) -> (s? t:f=w2767:i32)
                          }
                        }
                        n796 = case shown="3" w2665 {
                          tunnel: w2671 -> [_ _ _ _ _ _ _ _ _ _ _ _]
                          tunnel: w2670 -> [w2672 w2674 w2676 w2681 w2686 w2693 w2700 w2705 w2709 w2715 w2720 w2725]
                          tunnel: [w2672 w2674 w2676 w2679 w2684 w2691 w2698 w2703 w2708 w2713 w2718 w2723] -> w2669
                          tunnel: w2668 -> [w2673 w2675 w2677 w2682 w2687 w2694 w2701 w2706 w2711 w2716 w2721 w2726]
                          tunnel: [w2673 w2675 w2677 w2680 w2685 w2692 w2699 w2704 w2710 w2714 w2719 w2724] -> w2667
                          frame 0, Default {
                          }
                          frame 1 {
                          }
                          frame 2 {
                          }
                          frame 3 {
                            n797 = property class="IOTask"(reference=w2682, error in=w2681, "Channel.CI.CountEdges.GateFunction"="Gate Function 2") -> (reference out=w2680:refnum<k24>, error out=w2679:errorcluster)
                          }
                          frame 4 {
                            n798 = property class="IOTask"(reference=w2687, error in=w2686, "Channel.CI.CountEdges.ClearOnRead"="ClearOnRead") -> (reference out=w2685:refnum<k24>, error out=w2684:errorcluster)
                          }
                          frame 5 {
                            n799 = property class="IOTask"(reference=w2694, error in=w2693, "Channel.CI.CountEdges.RangeLimitOn"="RangeLimOn", "Channel.CI.CountEdges.Registers.MaxLimit"="MaxLimit", "Channel.CI.CountEdges.Registers.MinLimit"="MinLimit") -> (reference out=w2692:refnum<k24>, error out=w2691:errorcluster)
                          }
                          frame 6 {
                            n800 = property class="IOTask"(reference=w2701, error in=w2700, "Channel.CI.CountEdges.OutputOn"="Output", "Channel.CI.CountEdges.Registers.OutputVal0"="Out0", "Channel.CI.CountEdges.Registers.OutputVal1"="Out1") -> (reference out=w2699:refnum<k24>, error out=w2698:errorcluster)
                          }
                          frame 7 {
                            n801 = property class="IOTask"(reference=w2706, error in=w2705, "Channel.CI.CountEdges.Recycle"="Recycle") -> (reference out=w2704:refnum<k24>, error out=w2703:errorcluster)
                          }
                          frame 8 {
                            n802 = property class="IOTask"(reference=w2711, error in=w2709, "Channel.CI.CountEdges.InvertGate"="Invert Gate") -> (reference out=w2710:refnum<k24>, error out=w2708:errorcluster)
                          }
                          frame 9 {
                            n803 = property class="IOTask"(reference=w2716, error in=w2715, "Channel.CI.CountEdges.CountDirection"="MccDirection") -> (reference out=w2714:refnum<k24>, error out=w2713:errorcluster)
                          }
                          frame 10 {
                            n804 = property class="IOTask"(reference=w2721, error in=w2720, "Channel.CI.CountEdges.Edge"="MccEdge") -> (reference out=w2719:refnum<k24>, error out=w2718:errorcluster)
                          }
                          frame 11 {
                            n805 = property class="IOTask"(reference=w2726, error in=w2725, "Channel.CI.CountEdges.OutputInitialState"="Initial State") -> (reference out=w2724:refnum<k24>, error out=w2723:errorcluster)
                          }
                        }
                      }
                    }
                    frame "CO" {
                      n806 = for {
                        N: 2 -> [_]
                        tunnel: w2776 -> [w2781]
                        shift-right: [w2783] -> w2772
                        shift-left: w2774 -> [w2778]
                        shift-right: [w2782] -> w2771
                        shift-left: w2775 -> [w2777]
                        i -> [w2780]
                        n807 = case shown="1" w2780 {
                          tunnel: [w2784 w2788] -> w2779
                          frame 0, Default {
                            n808 = Select(t=1, s="Freq 3", f=0) -> (s? t:f=w2784:i32)
                          }
                          frame 1 {
                            n809 = Select(t=2, s="Duty", f=0) -> (s? t:f=w2788:i32)
                          }
                        }
                        n810 = case shown="1" w2779 {
                          tunnel: w2778 -> [w2793 w2798 w2801]
                          tunnel: w2777 -> [w2792 w2797 w2803]
                          tunnel: [w2793 w2796 w2800] -> w2783
                          tunnel: [w2792 w2795 w2802] -> w2782
                          tunnel: w2781 -> [_ _ _]
                          frame 0, Default {
                          }
                          frame 1 {
                            n811 = property class="IOTask"(reference=w2798, error in=w2797, "Channel.CO.Pulse.Frequency.Frequency"="Frequency") -> (reference out=w2796:refnum<k24>, error out=w2795:errorcluster)
                          }
                          frame 2 {
                            n812 = property class="IOTask"(reference=w2801, error in=w2803, "Channel.CO.Pulse.Frequency.DutyCycle"="DutyCycle") -> (reference out=w2800:refnum<k24>, error out=w2802:errorcluster)
                          }
                        }
                      }
                    }
                  }
                }
              }
            }
          }
          n813 = local write "Props"(w1952) -> ()
        }
        frame 14 {
          # "Task Control"
          n814 = for {
            N: 5 -> [_]
            tunnel: w2806 -> [w2811]
            tunnel: [FALSE] -> w2807
            n815 = Wait Until Next ms Multiple(millisecond multiple=w2811) -> ()  [unwired: 1 out]
            "TC" <- TRUE
          }
          n816 = local write "TC"(w2807) -> ()
          n817 = local write "NI\nTC"(FALSE ("TC")) -> ()
        }
      }
      n818 = Select(t=u32 20 ("millisecond multiple"), s=w23, f="Loop") -> (s? t:f=w25:u32)
      n819 = Wait Until Next ms Multiple(millisecond multiple=w25) -> ()  [unwired: 1 out]
    }
  }
  n820 = local write "message 2"("") -> ()
  n821 = local write "Task"(0 ("Task")) -> ()
  n822 = local write "Task Cleared"(w4) -> ()
  n823 = local write "Task Stopped"(w4) -> ()
  n824 = call <vilib>:"ULx Clear Task.vi"("task in"=w2) -> ()  [unwired: 14 in, 1 out]
  n825 = local write "stop"(w5) -> ()
